vi "数据编码.vi"(0 "table输入":string(combo), 5 "错误常量 2":errorcluster caption="错误输入", 9 "QN":string, 13 "MN":string, 14 "PW":string) -> (4 "错误常量":errorcluster caption="错误输出", 15 "通讯包字符串":string)   [LabVIEW 2016, in "数据传输系统.lvlib"]
panel:
  in  "时间戳 2":string
  out "核查数据发送次数":i32
  out "小时数据发送次数":i32
  out "长度":i32
  in  "数据块":T1
  out "通讯包":T2={"包头（2）"="##", "数据段长度（4）"="", "数据段"="", "CRC校验"="", "包尾"=""}
  # "范例代码：\n\n##0101QN=20160801085857223;ST=32;CN=1062;PW=100000;MN=010000A8900016F000169DC0;Flag=5\n;CP=&&RtdInterval=30&&1C80\\r\\n"
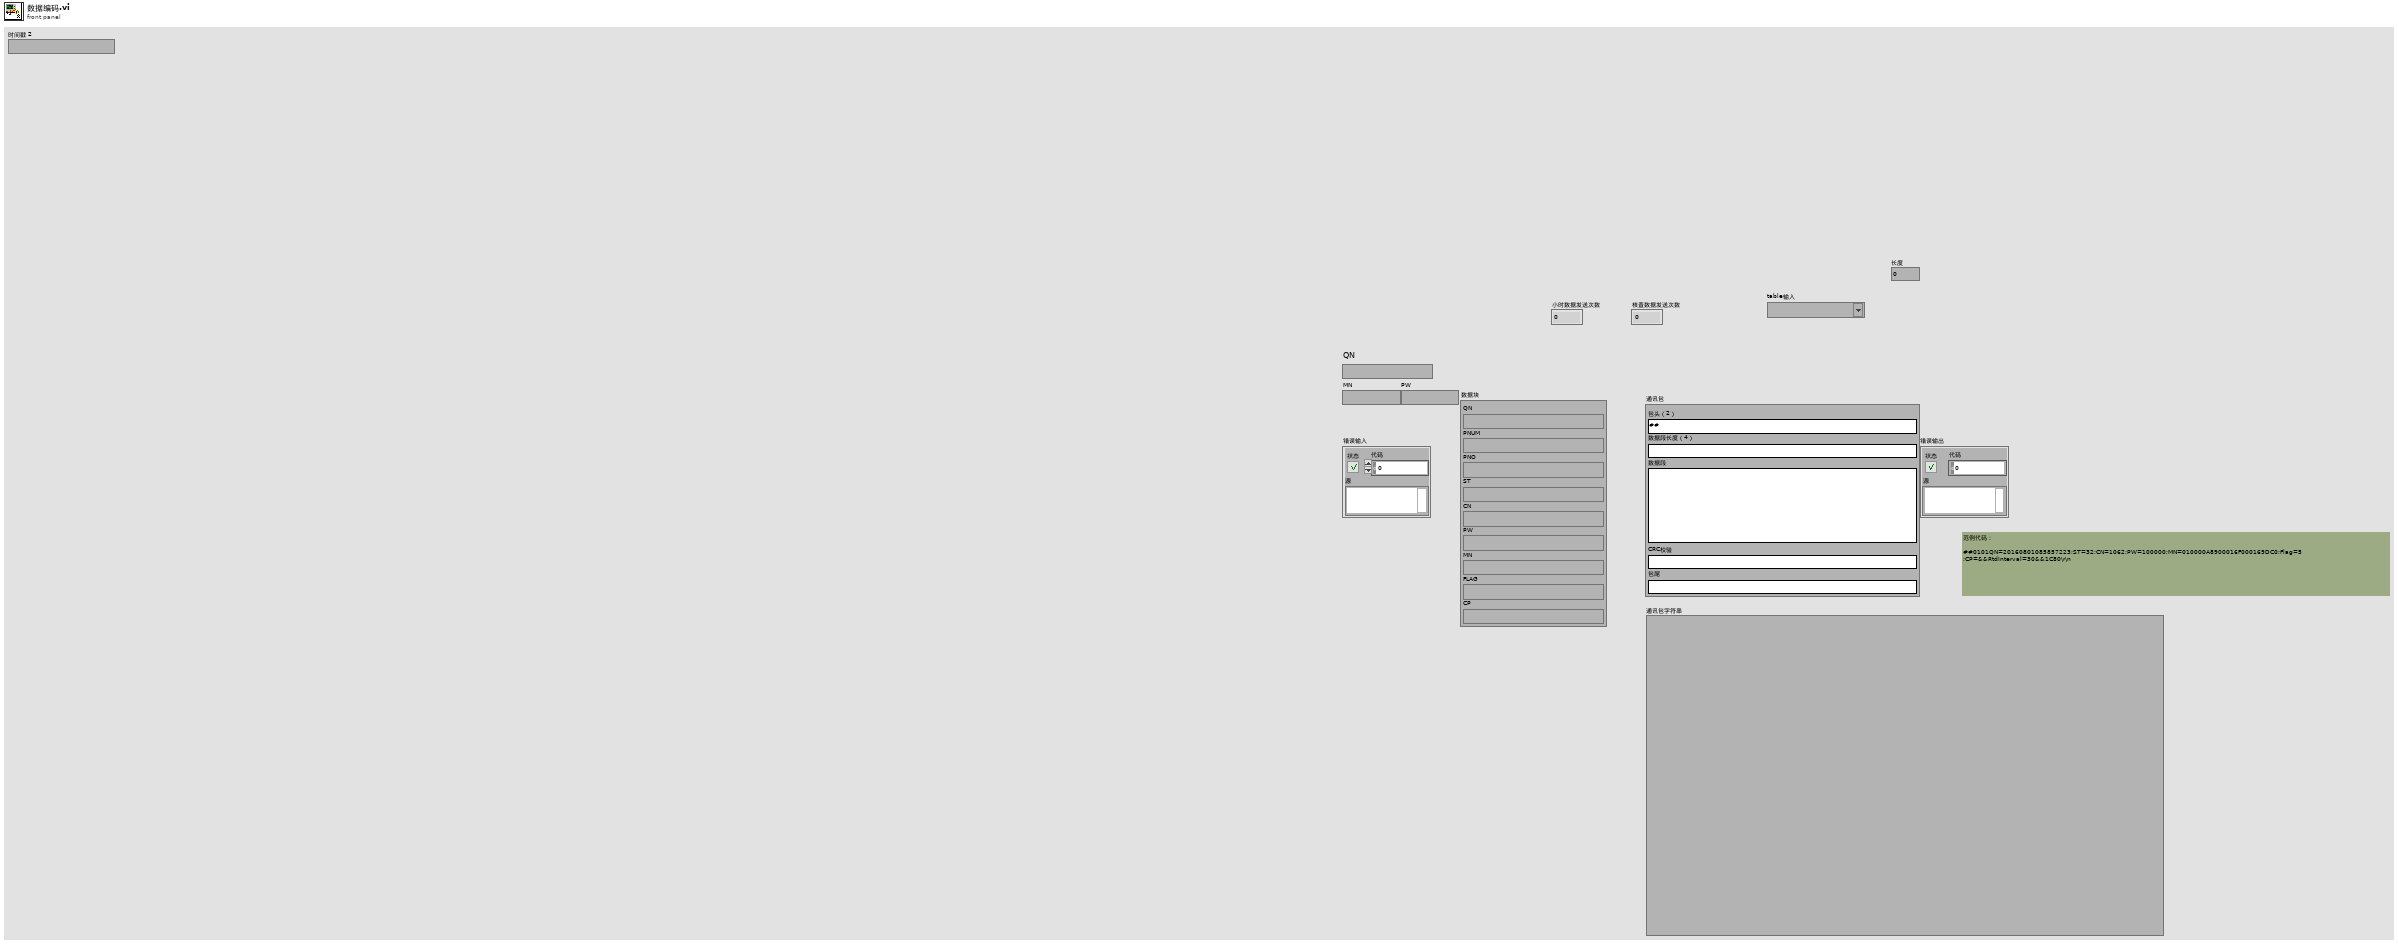
[diagram p1: front panel]
types:
  T1 = cluster{"QN":string, "ST":string, "CN":string, "PW":string, "MN":string, "FLAG":string, "PNUM":string, "PNO":string, "CP":string}
  T2 = cluster{"包头（2）":string, "数据段长度（4）":string, "数据段":string, "CRC校验":string, "包尾":string}
  T3 = cluster{"PH":string[][], "CODCr":string[][], "氨氮":string[][], "CODMn":string[][], "总氮":string[][], "总磷":string[][], "电导率":string[][], "水温":string[][], "DO":string[][], "浊度":string[][], "叶绿素":string[][], "藻密度":string[][], "铜":string[][], "盐度":string[][], "水位":string[][], "流速":string[][], "瞬时流量":string[][], "累积流量":string[][], "亚硝酸盐":string[][], "硫化物":string[][], "ORP":string[][], "铅":string[][], "镉":string[][], "锌":string[][], "镍":string[][], "锰":string[][], "汞":string[][]}
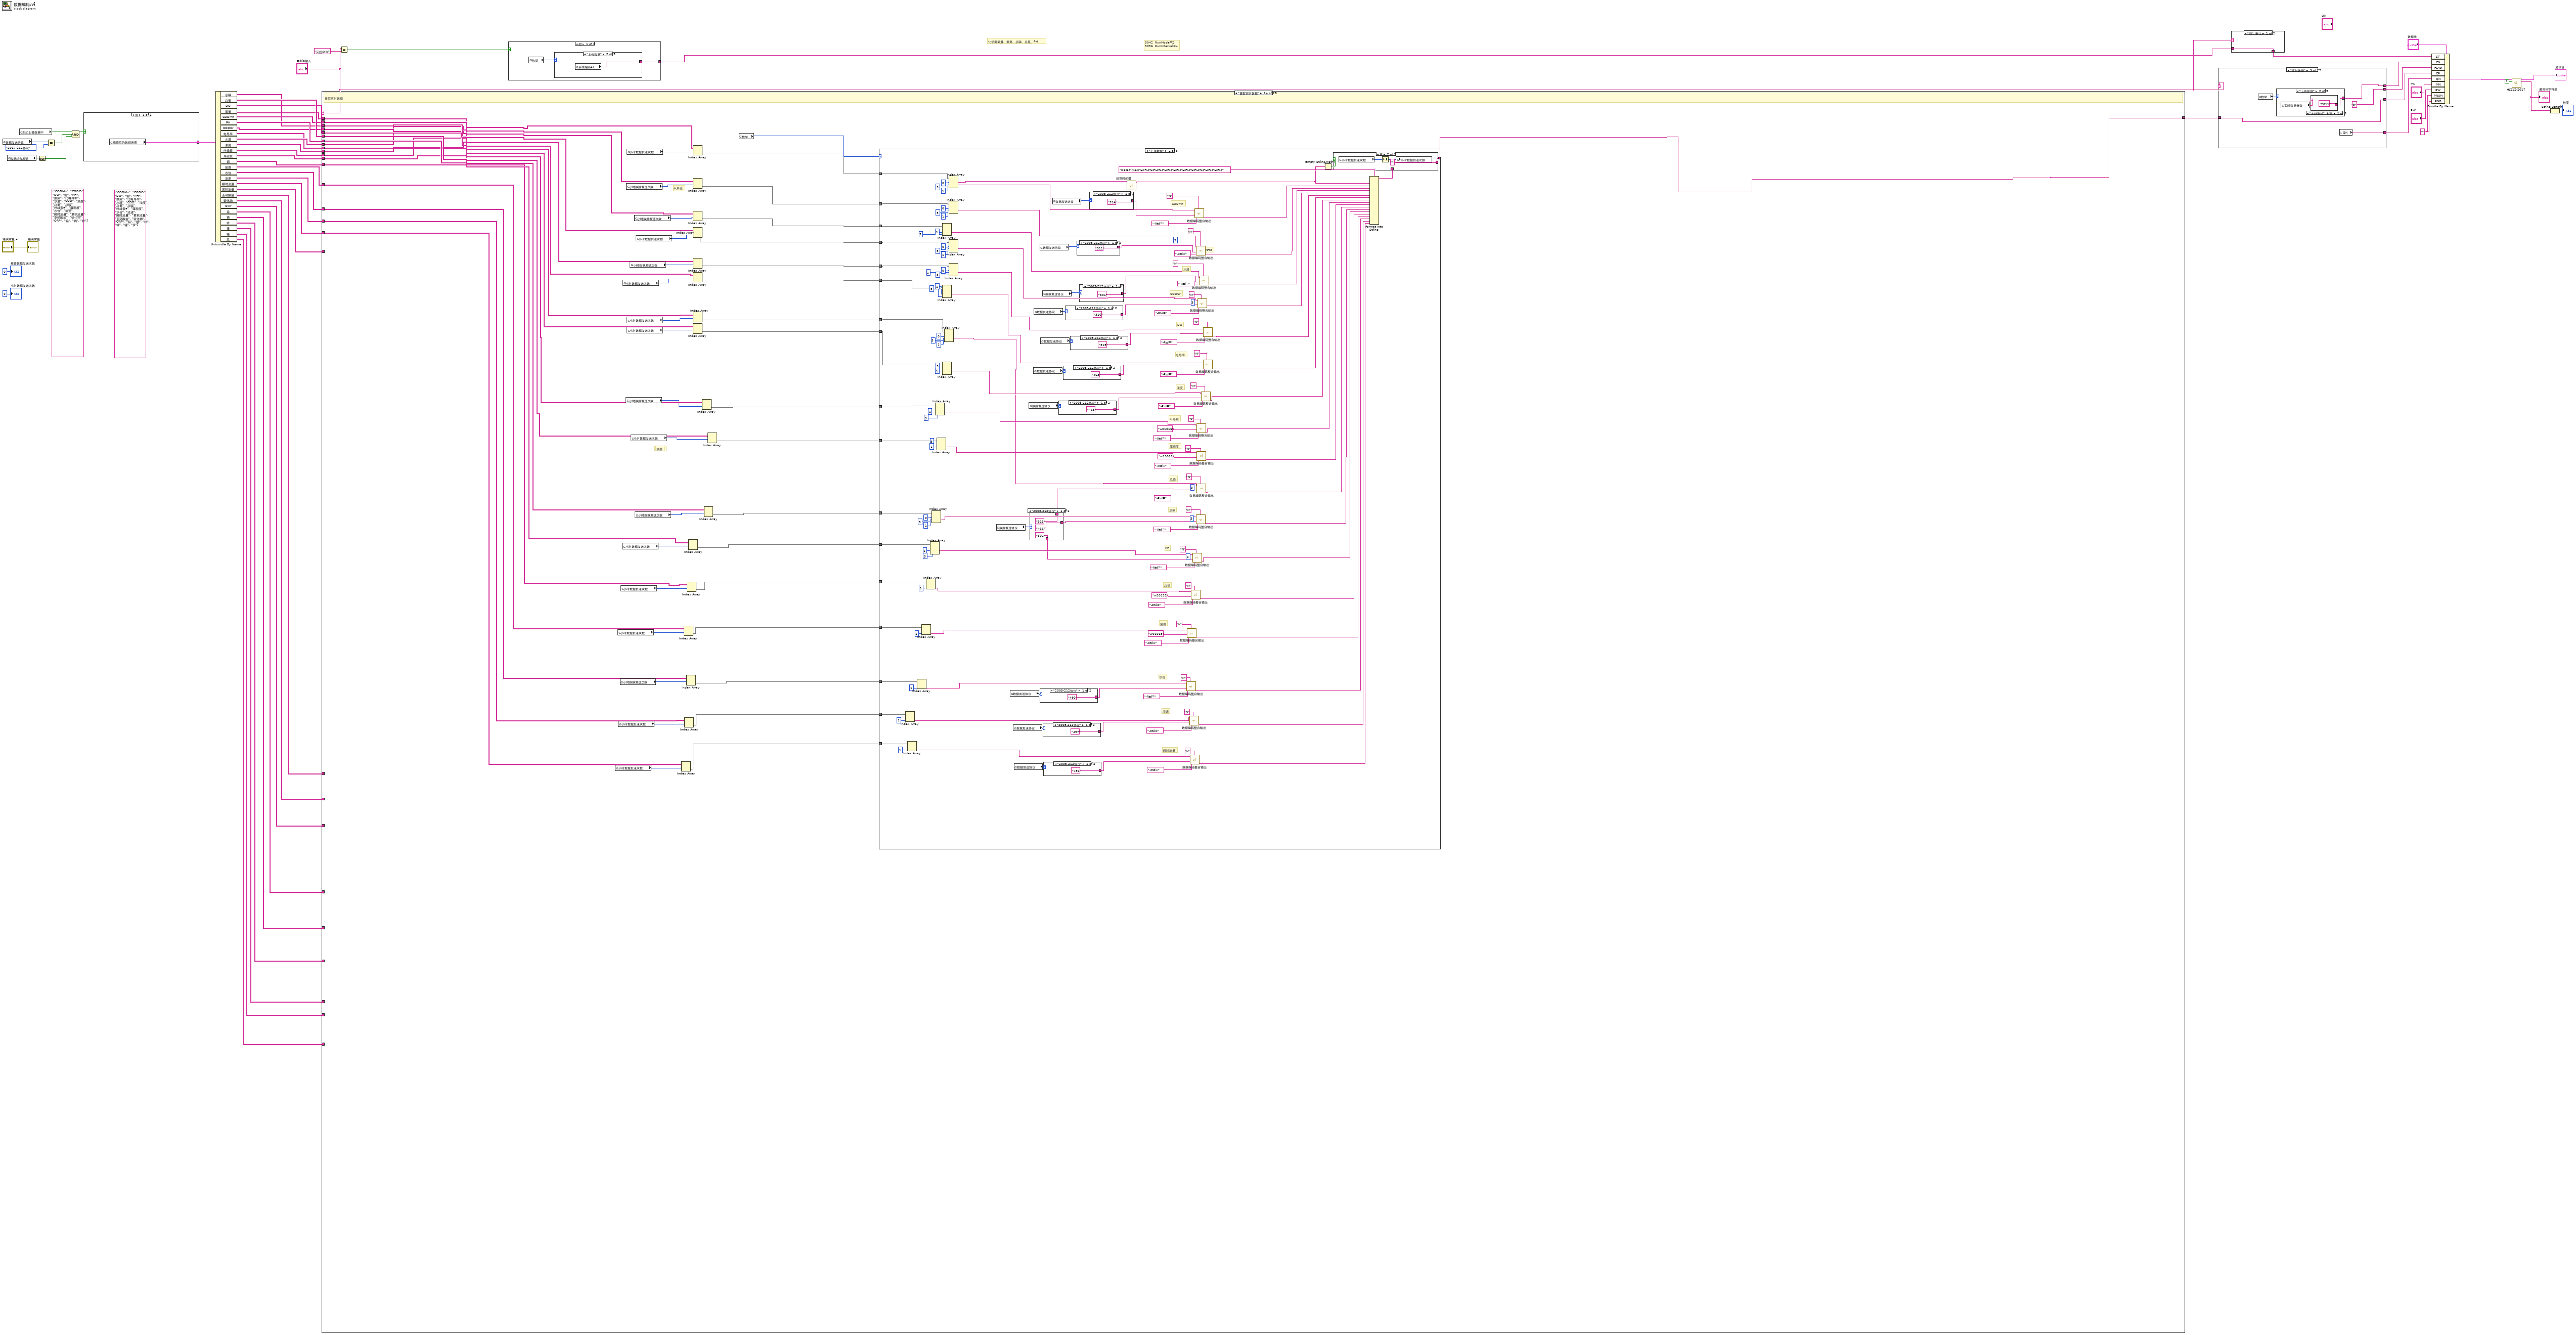
[diagram p0: block diagram]
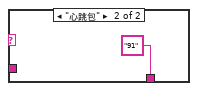
[diagram p2: hidden frame]
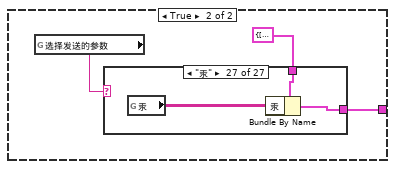
[diagram p3: hidden frame]
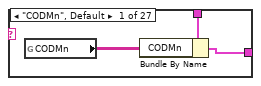
[diagram p4: hidden frame]
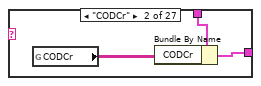
[diagram p5: hidden frame]
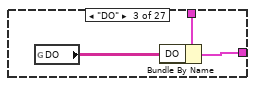
[diagram p6: hidden frame]
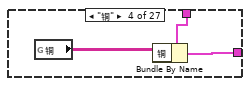
[diagram p7: hidden frame]
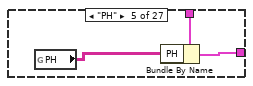
[diagram p8: hidden frame]
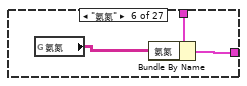
[diagram p9: hidden frame]
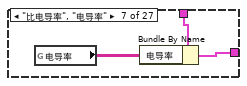
[diagram p10: hidden frame]
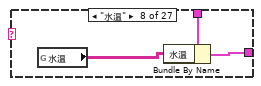
[diagram p11: hidden frame]
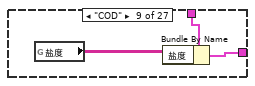
[diagram p12: hidden frame]
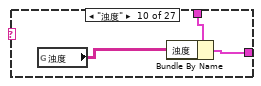
[diagram p13: hidden frame]
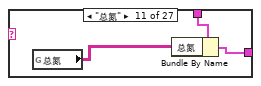
[diagram p14: hidden frame]
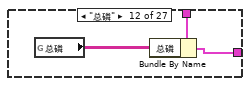
[diagram p15: hidden frame]
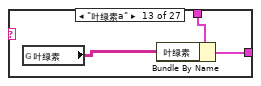
[diagram p16: hidden frame]
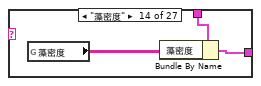
[diagram p17: hidden frame]
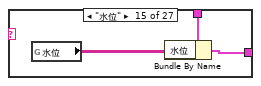
[diagram p18: hidden frame]
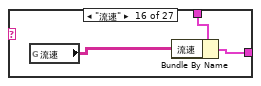
[diagram p19: hidden frame]
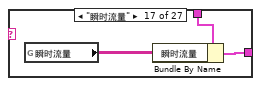
[diagram p20: hidden frame]
diagram:
  (unwired) string[] ["CODMn", "CODCr", "DO", "铜", "PH", "氨氮", "比电导率", "水温", "COD", "浊度", "总氮", "总磷", "叶绿素a", "藻密度", "水位", "流速", "瞬时流量", "累积流量", "亚硝酸盐", "硫化物", "ORP", "铅", "镉", "锌"] ("数组")
  (unwired) string[] ["CODMn", "CODCr", "DO", "铜", "PH", "氨氮", "比电导率", "水温", "COD", "浊度", "总氮", "总磷", "叶绿素a", "藻密度", "水位", "流速", "瞬时流量", "累积流量", "亚硝酸盐", "硫化物", "ORP", "铅", "镉", "锌", "镍", "锰", "汞"] ("数组")
  w42 = ""
  # "化学需氧量、氨氮、总磷、总氮、PH"
  # "3042  RunMode=2\n3056  RunInterval=4"
  n1 = global read "断电保存全局.vi" "数据发送协议"() -> (w15:enum16{"2005-212协议", "2017-212协议"})
  n2 = global read "断电保存全局.vi" "数据组合发送"() -> (w17:bool)
  n3 = global read "全局 数据发送重叠.vi" "主动上报数据中"() -> (w29:bool)
  n4 = Not(x=w17) -> (.not. x?=w16:bool)
  n5 = Equal?(x=w15, y=enum16{"2005-212协议", "2017-212协议"}."2017-212协议" ("数据发送版本")) -> (x = y?=w20:bool)
  n6 = Compound Arithmetic op=AND ("复合运算")(w29, w20, w16) -> (w21:bool)
  n7 = case shown="假" w21 {
    tunnel: [w58 w60] -> w30
    frame False {
      n8 = global read "插值后的新数组.vi" "插值后的数组元素"() -> (w58:T3)
    }
    frame True {
      n9 = global read "全局 水样时间.vi" "选择发送的参数"() -> (w61:string)
      n10 = case shown="\"汞\"" w61 {
        tunnel: T3 {"PH"=[], "CODCr"=[], "氨氮"=[], "CODMn"=[], "总氮"=[], "总磷"=[], "电导率"=[], "水温"=[], "DO"=[], "浊度"=[], "叶绿素"=[], "藻密度"=[], "铜"=[], "盐度"=[], "水位"=[], "流速"=[], "瞬时流量"=[], "累积流量"=[], "亚硝酸盐"=[], "硫化物"=[], "ORP"=[], "铅"=[], "镉"=[], "锌"=[], "镍"=[], "锰"=[], "汞"=[]} ("插值后的数组元素") -> [w63 w67 w70 w73 w76 w79 w82 w85 w88 w91 w94 w97 w100 w102 w106 w109 w111 w114 w117 w120 w123 w126 w129 w132 w135 w138 w141]
        tunnel: [w62 w65 w68 w71 w74 w77 w81 w84 w86 w89 w92 w95 w98 w101 w104 w107 w110 w113 w116 w119 w122 w125 w128 w131 w134 w137 w140] -> w60
        frame "CODMn", Default {
          n11 = global read "全局 所有参数.vi" "CODMn"() -> (w64:string[][])
          n12 = Bundle By Name(cluster=w63, "CODMn"=w64) -> (w62:T3)
        }
        frame "CODCr" {
          n13 = global read "全局 所有参数.vi" "CODCr"() -> (w66:string[][])
          n14 = Bundle By Name(cluster=w67, "CODCr"=w66) -> (w65:T3)
        }
        frame "DO" {
          n15 = global read "全局 所有参数.vi" "DO"() -> (w69:string[][])
          n16 = Bundle By Name(cluster=w70, "DO"=w69) -> (w68:T3)
        }
        frame "铜" {
          n17 = global read "全局 所有参数.vi" "铜"() -> (w72:string[][])
          n18 = Bundle By Name(cluster=w73, "铜"=w72) -> (w71:T3)
        }
        frame "PH" {
          n19 = global read "全局 所有参数.vi" "PH"() -> (w75:string[][])
          n20 = Bundle By Name(cluster=w76, "PH"=w75) -> (w74:T3)
        }
        frame "氨氮" {
          n21 = global read "全局 所有参数.vi" "氨氮"() -> (w78:string[][])
          n22 = Bundle By Name(cluster=w79, "氨氮"=w78) -> (w77:T3)
        }
        frame "比电导率", "电导率" {
          n23 = global read "全局 所有参数.vi" "电导率"() -> (w80:string[][])
          n24 = Bundle By Name(cluster=w82, "电导率"=w80) -> (w81:T3)
        }
        frame "水温" {
          n25 = global read "全局 所有参数.vi" "水温"() -> (w83:string[][])
          n26 = Bundle By Name(cluster=w85, "水温"=w83) -> (w84:T3)
        }
        frame "COD" {
          n27 = global read "全局 所有参数.vi" "盐度"() -> (w87:string[][])
          n28 = Bundle By Name(cluster=w88, "盐度"=w87) -> (w86:T3)
        }
        frame "浊度" {
          n29 = global read "全局 所有参数.vi" "浊度"() -> (w90:string[][])
          n30 = Bundle By Name(cluster=w91, "浊度"=w90) -> (w89:T3)
        }
        frame "总氮" {
          n31 = global read "全局 所有参数.vi" "总氮"() -> (w93:string[][])
          n32 = Bundle By Name(cluster=w94, "总氮"=w93) -> (w92:T3)
        }
        frame "总磷" {
          n33 = global read "全局 所有参数.vi" "总磷"() -> (w96:string[][])
          n34 = Bundle By Name(cluster=w97, "总磷"=w96) -> (w95:T3)
        }
        frame "叶绿素a" {
          n35 = global read "全局 所有参数.vi" "叶绿素"() -> (w99:string[][])
          n36 = Bundle By Name(cluster=w100, "叶绿素"=w99) -> (w98:T3)
        }
        frame "藻密度" {
          n37 = global read "全局 所有参数.vi" "藻密度"() -> (w103:string[][])
          n38 = Bundle By Name(cluster=w102, "藻密度"=w103) -> (w101:T3)
        }
        frame "水位" {
          n39 = global read "全局 所有参数.vi" "水位"() -> (w105:string[][])
          n40 = Bundle By Name(cluster=w106, "水位"=w105) -> (w104:T3)
        }
        frame "流速" {
          n41 = global read "全局 所有参数.vi" "流速"() -> (w108:string[][])
          n42 = Bundle By Name(cluster=w109, "流速"=w108) -> (w107:T3)
        }
        frame "瞬时流量" {
          n43 = global read "全局 所有参数.vi" "瞬时流量"() -> (w112:string[][])
          n44 = Bundle By Name(cluster=w111, "瞬时流量"=w112) -> (w110:T3)
        }
        frame "累积流量" {
          n45 = global read "全局 所有参数.vi" "累积流量"() -> (w115:string[][])
          n46 = Bundle By Name(cluster=w114, "累积流量"=w115) -> (w113:T3)
        }
        frame "亚硝氮" {
          n47 = global read "全局 所有参数.vi" "亚硝酸盐"() -> (w118:string[][])
          n48 = Bundle By Name(cluster=w117, "亚硝酸盐"=w118) -> (w116:T3)
        }
        frame "硫化物" {
          n49 = global read "全局 所有参数.vi" "硫化物"() -> (w121:string[][])
          n50 = Bundle By Name(cluster=w120, "硫化物"=w121) -> (w119:T3)
        }
        frame "ORP" {
          n51 = global read "全局 所有参数.vi" "ORP"() -> (w124:string[][])
          n52 = Bundle By Name(cluster=w123, "ORP"=w124) -> (w122:T3)
        }
        frame "铅" {
          n53 = global read "全局 所有参数.vi" "铅"() -> (w127:string[][])
          n54 = Bundle By Name(cluster=w126, "铅"=w127) -> (w125:T3)
        }
        frame "镉" {
          n55 = global read "全局 所有参数.vi" "镉"() -> (w130:string[][])
          n56 = Bundle By Name(cluster=w129, "镉"=w130) -> (w128:T3)
        }
        frame "锌" {
          n57 = global read "全局 所有参数.vi" "锌"() -> (w133:string[][])
          n58 = Bundle By Name(cluster=w132, "锌"=w133) -> (w131:T3)
        }
        frame "镍" {
          n59 = global read "全局 所有参数.vi" "镍"() -> (w136:string[][])
          n60 = Bundle By Name(cluster=w135, "镍"=w136) -> (w134:T3)
        }
        frame "锰" {
          n61 = global read "全局 所有参数.vi" "锰"() -> (w139:string[][])
          n62 = Bundle By Name(cluster=w138, "锰"=w139) -> (w137:T3)
        }
        frame "汞" {
          n63 = global read "全局 所有参数.vi" "汞"() -> (w142:string[][])
          n64 = Bundle By Name(cluster=w141, "汞"=w142) -> (w140:T3)
        }
      }
    }
  }
  n65 = Unbundle By Name(w30) -> ("总磷"=w23:string[][], "总氮"=w28:string[][], "DO"=w27:string[][], "氨氮"=w26:string[][], "CODMn"=w24:string[][], "PH"=w41:string[][], "CODCr"=w25:string[][], "电导率"=w19:string[][], "水温"=w40:string[][], "浊度"=w18:string[][], "叶绿素"=w39:string[][], "藻密度"=w36:string[][], "铜"=w35:string[][], "盐度"=w34:string[][], "水位"=w33:string[][], "流速"=w32:string[][], "瞬时流量"=w31:string[][], "累积流量"=w1:string[][], "亚硝酸盐"=w14:string[][], "硫化物"=w13:string[][], "ORP"=w12:string[][], "铅"=w10:string[][], "镉"=w9:string[][], "锌"=w8:string[][], "镍"=w7:string[][], "锰"=w6:string[][], "汞"=w5:string[][])
  n66 = case shown="\"提取实时数据\"" "table输入" {
    tunnel: [w144 w151 w165 w208 w231 _ w245 w254 w290 w1335 w1760 w1807 w1905 w2123 w2351 w2584 w2651 w2697 w2745 w2817 w2945 w3059 w3173 w3266 w3720 w3756 w3767 w3778] -> w37
    tunnel: w24 -> [_ _ _ _ _ _ _ _ w288 w1334 _ _ w1904 w2135 w2355 w2588 w2655 w2696 w2744 w2816 w2944 w3058 w3172 w3265 _ _ _ _]
    tunnel: w26 -> [_ _ _ _ _ _ _ _ w287 w1333 _ _ w1903 w2134 w2354 w2587 w2656 w2695 w2743 w2815 w2943 w3057 w3171 w3264 _ _ _ _]
    tunnel: w27 -> [_ _ _ _ _ _ _ _ w284 w1332 _ _ w1902 w2133 w2333 _ _ _ w2739 w2814 w2942 w3056 w3170 w3244 _ _ _ _]
    tunnel: w23 -> [_ _ _ _ _ _ _ _ w279 w1331 _ _ w1901 w2132 w2353 w2586 w2654 w2694 w2740 w2813 w2941 w3055 w3169 w3263 _ _ _ _]
    tunnel: w28 -> [_ _ _ _ _ _ _ _ w278 w1330 _ _ w1900 w2131 w2352 w2585 w2653 w2692 w2742 w2812 w2940 w3054 w3168 w3262 _ _ _ _]
    tunnel: w41 -> [_ _ _ _ _ _ _ _ w285 w1329 _ _ w1899 w2130 w2337 _ _ _ w2738 _ w2924 w3038 w3146 w3242 _ _ _ _]
    tunnel: w25 -> [_ _ _ _ _ _ _ _ w271 w1328 _ _ w1898 w2129 w2350 w2583 w2652 w2693 w2741 w2799 w2928 w3042 w3156 w3249 _ _ _ _]
    tunnel: w19 -> [_ _ _ _ _ _ _ _ w283 w1327 _ _ w1897 w2128 w2330 _ _ _ w2736 _ w2921 w3035 w3144 w3239 _ _ _ _]
    tunnel: w40 -> [_ _ _ _ _ _ _ _ w286 w1326 _ _ w1896 w2127 _ _ _ _ w2737 _ w2918 w3032 w3145 w3234 _ _ _ _]
    tunnel: w18 -> [_ _ _ _ _ _ _ _ w282 w1325 _ _ w1895 w2126 w2327 _ _ _ w2735 _ w2912 w3026 w3140 w3233 _ _ _ _]
    tunnel: w39 -> [_ _ _ _ _ _ _ _ w281 w1324 _ _ w1894 w2125 _ _ _ _ _ _ w2910 w3024 w3138 w3232 _ _ _ _]
    tunnel: w36 -> [_ _ _ _ _ _ _ _ w280 w1323 _ _ w1893 w2124 _ _ _ _ _ _ w2908 w3022 w3137 w3247 _ _ _ _]
    tunnel: w35 -> [_ _ _ _ _ _ _ _ w277 w1293 _ _ w1863 w2095 _ _ _ _ _ _ _ _ _ _ _ _ _ _]
    tunnel: w34 -> [_ _ _ _ _ _ _ _ w276 w1292 _ _ w1862 w2094 _ _ _ _ _ _ _ _ _ _ _ _ _ _]
    tunnel: w33 -> [_ _ _ _ _ _ _ _ w274 w1283 _ _ w1858 w2088 _ _ _ _ _ _ _ _ _ _ _ _ _ _]
    tunnel: w32 -> [_ _ _ _ _ _ _ _ w275 w1282 _ _ w1856 w2087 _ _ _ _ _ _ _ _ _ _ _ _ _ _]
    tunnel: w31 -> [_ _ _ _ _ _ _ _ w273 w1281 _ _ w1854 w2086 _ _ _ _ _ _ _ _ _ _ _ _ _ _]
    tunnel: w1 -> [_ _ _ _ _ _ _ _ w272 w1280 _ _ _ _ _ _ _ _ _ _ _ _ _ _ _ _ _ _]
    tunnel: w14 -> [_ _ _ _ _ _ _ _ w270 w1276 _ _ _ _ _ _ _ _ _ _ _ _ _ _ _ _ _ _]
    tunnel: w13 -> [_ _ _ _ _ _ _ _ w269 w1275 _ _ _ _ _ _ _ _ _ _ _ _ _ _ _ _ _ _]
    tunnel: w12 -> [_ _ _ _ _ _ _ _ w268 w1274 _ _ _ _ _ _ _ _ _ _ w2906 w3020 w3136 _ _ _ _ _]
    tunnel: w10 -> [_ _ _ _ _ _ _ _ w267 w1267 _ _ _ _ _ _ _ _ _ _ _ _ _ _ _ _ _ _]
    tunnel: w9 -> [_ _ _ _ _ _ _ _ w266 w1266 _ _ _ _ _ _ _ _ _ _ _ _ _ _ _ _ _ _]
    tunnel: w8 -> [_ _ _ _ _ _ _ _ w265 w1265 _ _ _ _ _ _ _ _ _ _ _ _ _ _ _ _ _ _]
    tunnel: w7 -> [_ _ _ _ _ _ _ _ w264 w1258 _ _ _ _ _ _ _ _ _ _ _ _ _ _ _ _ _ _]
    tunnel: w6 -> [_ _ _ _ _ _ _ _ w263 w1257 _ _ _ _ _ _ _ _ _ _ _ _ _ _ _ _ _ _]
    tunnel: w5 -> [_ _ _ _ _ _ _ _ w262 w1256 _ _ _ _ _ _ _ _ _ _ _ _ _ _ _ _ _ _]
    frame "反控命令" {
      n67 = global read "全局 反控命令枚举.vi" "反控命令枚举"() -> (w143:enum16{"返回请求应答", "返回执行结果"})
      n68 = case shown="\"返回执行结果\"" w143 {
        tunnel: ["QnRtn=1" w147] -> w144
        frame "返回请求应答", Default {
        }
        frame "返回执行结果" {
          n69 = global read "全局 反控命令枚举.vi" "执行结果定义"() -> (w148:u16)
          n70 = Number To Decimal String(number=w148) -> (decimal integer string=w146:string)  [unwired: 1 in]
          n71 = Concatenate Strings("ExeRtn=", w146) -> (w147:string)
        }
      }
    }
    frame "超标留样返回" {
      n72 = global read "全局1.vi" "枚举"() -> (w150:enum16{"返回请求应答", "上传数据", "返回执行结果"})
      n73 = case shown="\"返回请求应答\", 默认" w150 {
        tunnel: ["QnRtn=1" w153 "ExeRtn=1"] -> w151
        frame "返回请求应答", Default {
        }
        frame "上传数据" {
          n74 = global read "全局1.vi" "register values"() -> (w162:u16[])
          n75 = Index Array(array=w162, index=7 ("索引")) -> (element=w155:u16)
          n76 = Get Date/Time In Seconds() -> (seconds since 1Jan1904=w160:timestamp)
          n77 = Number To Decimal String(number=w155) -> (decimal integer string=w156:string)  [unwired: 1 in]
          n78 = Format Date/Time String(time format string (%c)="%Y%m%d%H%M%S" ("时间格式字符串(%c)"), seconds (now)=w160) -> (date/time string=w158:string)  [unwired: 1 in]
          n79 = Format Into String(format string="VaseNo=%s" ("格式字符串"), w156) -> (resulting string=w154:string)  [unwired: 2 in, 1 out]
          n80 = Format Into String(format string="DataTime=%s;%s" ("格式字符串"), w158, w154) -> (resulting string=w153:string)  [unwired: 2 in, 1 out]
        }
        frame "返回执行结果" {
        }
      }
    }
    frame "提取经纬度环境信息" {
      # "BDS纬度"
      # "BDS纬度"
      # "GPS纬度"
      # "GPS经度"
      # "湿度"
      # "温度"
      # "电压"
      # "时间"
      n81 = global read "全局1.vi" "枚举"() -> (w166:enum16{"返回请求应答", "上传数据", "返回执行结果"})
      n82 = case shown="\"上传数据\"" w166 {
        tunnel: ["QnRtn=1" w179 "ExeRtn=1"] -> w165
        frame "返回请求应答", Default {
        }
        frame "上传数据" {
          n83 = global read "全局 环境参数.vi" "columns输出"() -> (w176:string[])
          n84 = Array Subset(array=w176, index=1 ("索引")) -> (w177:string[])  [unwired: 1 in]
          n85 = for {
            tunnel: w177 -> [w185] mode=indexing
            tunnel: [w184] -> w178 mode=indexing
            n86 = case shown="\"BDS经度\"" w185 {
              tunnel: ["" "Volt=%s;" "Temp=%s;" ("格式字符串") "Hum=%s;" ("格式字符串") "Lng=%s;" "Lat=%s;" "Lng2=%s;" "Lat2=%s;"] -> w184
              frame "假", Default {
              }
              frame "电压" {
              }
              frame "室温" {
              }
              frame "湿度" {
              }
              frame "GPS经度" {
              }
              frame "GPS纬度" {
              }
              frame "BDS经度" {
              }
              frame "BDS纬度" {
              }
            }
          }
          n87 = global read "全局 环境参数.vi" "环境参数"() -> (w169:string[][])
          n88 = Index Array(array=w169, index (row)=0 ("索引 (行)")) -> (element=w172:string[])  [unwired: 1 in]
          n89 = Array Subset(array=w172, index=1 ("索引")) -> (w174:string[])  [unwired: 1 in]
          n90 = for {
            shift-right: [w199] -> w168
            shift-left: "" -> [w198]
            tunnel: w178 -> [w197] mode=indexing
            tunnel: w174 -> [w195] mode=indexing
            n91 = Fract/Exp String To Number(string=w195) -> (number=w196:dbl)  [unwired: 3 in, 1 out]
            n92 = Empty String/Path?(string/path=w195) -> (empty?=w201:bool)
            n93 = Number To Fractional String(number=w196) -> (F-format string=w194:string)  [unwired: 3 in]
            n94 = case shown="假" w201 {
              tunnel: [w204 w205] -> w200
              tunnel: w197 -> [w203 _]
              tunnel: w194 -> [w202 _]
              tunnel: w194 -> [_ w205]
              frame False {
                n95 = Format Into String(format string=w203, w202) -> (resulting string=w204:string)  [unwired: 2 in, 1 out]
              }
              frame True {
              }
            }
            n96 = Concatenate Strings(w198, w200) -> (w199:string)
          }
          n97 = Get Date/Time In Seconds() -> (seconds since 1Jan1904=w181:timestamp)
          n98 = Format Date/Time String(time format string (%c)="%Y%m%d%H%M%S" ("时间格式字符串(%c)"), seconds (now)=w181) -> (date/time string=w180:string)  [unwired: 1 in]
          n99 = Format Into String(format string="DataTime=%s;%s" ("格式字符串"), w180, w168) -> (resulting string=w179:string)  [unwired: 2 in, 1 out]
        }
        frame "返回执行结果" {
        }
      }
    }
    frame "提取现场系统信息" {
      n100 = global read "全局1.vi" "枚举"() -> (w207:enum16{"返回请求应答", "上传数据", "返回执行结果"})
      n101 = case shown="\"上传数据\"" w207 {
        tunnel: ["QnRtn=1" w228 "ExeRtn=1"] -> w208
        frame "返回请求应答", Default {
        }
        frame "上传数据" {
          n102 = global read "全局1.vi" "register values"() -> (w227:u16[])
          n103 = Get Date/Time In Seconds() -> (seconds since 1Jan1904=w213:timestamp)
          n104 = Index Array(array=w227, index #1=0 ("索引"), index #2=6 ("索引")) -> (element #1=w223:u16, element #2=w210:u16)
          n105 = Format Date/Time String(time format string (%c)="%Y%m%d%H%M%S%u" ("时间格式字符串(%c)"), seconds (now)=w213) -> (date/time string=w216:string)  [unwired: 1 in]
          n106 = Number To Decimal String(number=w223) -> (decimal integer string=w225:string)  [unwired: 1 in]
          n107 = Number To Decimal String(number=w210) -> (decimal integer string=w219:string)  [unwired: 1 in]
          n108 = Search and Replace String(input string=w216, search string="." ("搜索字符串")) -> (result string=w212:string)  [unwired: 6 in, 3 out]
          n109 = Format Into String(format string="RunMode=%s;" ("格式字符串"), w225) -> (resulting string=w222:string)  [unwired: 2 in, 1 out]
          n110 = Format Into String(format string="RunInterval=%s;" ("格式字符串"), w219) -> (resulting string=w220:string)  [unwired: 2 in, 1 out]
          n111 = Format Into String(format string="SystemTime=%s;" ("格式字符串"), w212) -> (resulting string=w217:string)  [unwired: 2 in, 1 out]
          n112 = Concatenate Strings(w222, w220, w217) -> (w228:string)
        }
        frame "返回执行结果" {
        }
      }
    }
    frame "提取监测仪表时间" {
      n113 = global read "全局1.vi" "枚举"() -> (w230:enum16{"返回请求应答", "上传数据", "返回执行结果"})
      n114 = case shown="\"上传数据\"" w230 {
        tunnel: ["QnRtn=1" w243 "ExeRtn=1"] -> w231
        frame "返回请求应答", Default {
        }
        frame "上传数据" {
          n115 = global read "全局 提取仪器参数.vi" "仪器编码"() -> (w233:string)
          n116 = Get Date/Time In Seconds() -> (seconds since 1Jan1904=w236:timestamp)
          n117 = Format Date/Time String(time format string (%c)="%Y%m%d%H%M%S%u" ("时间格式字符串(%c)"), seconds (now)=w236) -> (date/time string=w239:string)  [unwired: 1 in]
          n118 = Search and Replace String(input string=w239, search string="." ("搜索字符串")) -> (result string=w235:string)  [unwired: 6 in, 3 out]
          n119 = Format Into String(format string="PolId=%s;" ("格式字符串"), w233) -> (resulting string=w241:string)  [unwired: 2 in, 1 out]
          n120 = Format Into String(format string="SystemTime=%s;" ("格式字符串"), w235) -> (resulting string=w234:string)  [unwired: 2 in, 1 out]
          n121 = Concatenate Strings(w241, w234) -> (w243:string)
        }
        frame "返回执行结果" {
        }
      }
    }
    frame "心跳包", Default {
    }
    frame "提取数采仪时间" {
      (unwired) ""
      n122 = global read "全局1.vi" "枚举"() -> (w246:enum16{"返回请求应答", "上传数据", "返回执行结果"})
      n123 = case shown="\"上传数据\"" w246 {
        tunnel: ["QnRtn=1" w248 "ExeRtn=1"] -> w245
        frame "返回请求应答", Default {
        }
        frame "上传数据" {
          n124 = Get Date/Time In Seconds() -> (seconds since 1Jan1904=w252:timestamp)
          n125 = Format Date/Time String(time format string (%c)="%Y%m%d%H%M%S" ("时间格式字符串(%c)"), seconds (now)=w252) -> (date/time string=w249:string)  [unwired: 1 in]
          n126 = Concatenate Strings("SystemTime=", w249) -> (w248:string)
        }
        frame "返回执行结果" {
        }
      }
    }
    frame "提取实时数据间隔" {
      (unwired) ""
      n127 = global read "全局1.vi" "枚举"() -> (w255:enum16{"返回请求应答", "上传数据", "返回执行结果"})
      n128 = case shown="\"上传数据\"" w255 {
        tunnel: ["QnRtn=1" w259 "ExeRtn=1"] -> w254
        frame "返回请求应答", Default {
        }
        frame "上传数据" {
          n129 = global read "实时数据发送间隔全局.vi" "实时数据发送间隔"() -> (w258:u32)
          n130 = Number To Decimal String(number=w258) -> (decimal integer string=w257:string)  [unwired: 1 in]
          n131 = Concatenate Strings("RtdInterval=", w257) -> (w259:string)
        }
        frame "返回执行结果" {
        }
      }
    }
    frame "实时数据" {
      # "包含质控数据主动上传"
      n132 = global read "全局 实时数据参数.vi" "实时数据参数"() -> (w289:string)
      n133 = case shown="\"水样测试\", 默认" w289 {
        tunnel: [w318 w696 w747 w826 w1088 w1157] -> w290
        tunnel: w288 -> [w317 w695 w746 w813 w1086 w1155]
        tunnel: w287 -> [w316 w694 w745 w814 w1085 w1154]
        tunnel: w286 -> [w315 w693 w744 w815 _ _]
        tunnel: w285 -> [w314 w692 w743 w816 w1081 _]
        tunnel: w284 -> [w313 w691 w742 w817 w1080 _]
        tunnel: w283 -> [w312 w690 w741 w818 w1079 _]
        tunnel: w282 -> [w311 w689 w740 w819 w1078 _]
        tunnel: w281 -> [w310 w688 w739 w820 w1077 _]
        tunnel: w280 -> [w309 w687 w738 w821 w1076 _]
        tunnel: w279 -> [w308 w686 w737 w822 w1084 w1153]
        tunnel: w278 -> [w307 w685 w736 w823 w1083 w1152]
        tunnel: w271 -> [w306 w684 w735 w824 w1082 w1151]
        tunnel: w277 -> [w305 w683 w734 w812 _ _]
        tunnel: w276 -> [w304 w682 w733 w811 _ _]
        tunnel: w274 -> [w303 _ _ _ _ _]
        tunnel: w273 -> [w302 _ _ _ _ _]
        tunnel: w272 -> [w301 _ _ _ _ _]
        tunnel: w275 -> [w300 _ _ _ _ _]
        tunnel: w270 -> [w299 _ w732 _ w1073 w1150]
        tunnel: w269 -> [w298 _ w731 _ w1074 w1149]
        tunnel: w268 -> [w297 _ w730 _ w1075 w1148]
        tunnel: w267 -> [w296 _ _ _ _ _]
        tunnel: w266 -> [w295 _ _ _ _ _]
        tunnel: w265 -> [w294 _ _ _ _ _]
        tunnel: w264 -> [w293 _ _ _ _ _]
        tunnel: w263 -> [w292 _ _ _ _ _]
        tunnel: w262 -> [w291 _ _ _ _ _]
        frame "水样测试", Default {
          n134 = global read "全局1.vi" "枚举"() -> (w319:enum16{"返回请求应答", "上传数据", "返回执行结果"})
          n135 = case shown="\"上传数据\"" w319 {
            tunnel: ["QnRtn=1" w554 "ExeRtn=1"] -> w318
            tunnel: w317 -> [_ w566 _]
            tunnel: w316 -> [_ w565 _]
            tunnel: w315 -> [_ w564 _]
            tunnel: w314 -> [_ w563 _]
            tunnel: w313 -> [_ w562 _]
            tunnel: w312 -> [_ w561 _]
            tunnel: w311 -> [_ w560 _]
            tunnel: w310 -> [_ w559 _]
            tunnel: w309 -> [_ w558 _]
            tunnel: w308 -> [_ w557 _]
            tunnel: w307 -> [_ w556 _]
            tunnel: w306 -> [_ w555 _]
            tunnel: w305 -> [_ w513 _]
            tunnel: w304 -> [_ w512 _]
            tunnel: w303 -> [_ w509 _]
            tunnel: w300 -> [_ w508 _]
            tunnel: w302 -> [_ w507 _]
            tunnel: w301 -> [_ w439 _]
            tunnel: w299 -> [_ w446 _]
            tunnel: w298 -> [_ w445 _]
            tunnel: w297 -> [_ w444 _]
            tunnel: w296 -> [_ w359 _]
            tunnel: w295 -> [_ w358 _]
            tunnel: w294 -> [_ w357 _]
            tunnel: w293 -> [_ w326 _]
            tunnel: w292 -> [_ w325 _]
            tunnel: w291 -> [_ w324 _]
            frame "返回请求应答", Default {
            }
            frame "上传数据" {
              # "汞"
              # "锰"
              # "镍"
              # "锌"
              # "镉"
              # "铅"
              # "藻密度"
              # "叶绿素a"
              # "浊度"
              # "电导率"
              # "DO"
              # "水温"
              # "CODMn"
              # "ORP"
              # "硫化物"
              # "亚硝酸盐"
              # "CODCr"
              # "总氮"
              # "总磷"
              # "PH"
              # "NH3"
              n136 = global read "断电保存全局.vi" "数据发送协议"() -> (w475:enum16{"2005-212协议", "2017-212协议"})
              n137 = global read "断电保存全局.vi" "数据发送协议"() -> (w479:enum16{"2005-212协议", "2017-212协议"})
              n138 = global read "断电保存全局.vi" "数据发送协议"() -> (w474:enum16{"2005-212协议", "2017-212协议"})
              n139 = global read "断电保存全局.vi" "数据发送协议"() -> (w477:enum16{"2005-212协议", "2017-212协议"})
              n140 = global read "断电保存全局.vi" "数据发送协议"() -> (w478:enum16{"2005-212协议", "2017-212协议"})
              n141 = global read "断电保存全局.vi" "数据发送协议"() -> (w476:enum16{"2005-212协议", "2017-212协议"})
              n142 = case shown="\"2017-212协议\", 默认" w474 {
                tunnel: ["060" ("污染物编码") "w21003" ("污染物编码")] -> w550
                frame "2005-212协议" {
                }
                frame "2017-212协议", Default {
                }
              }
              n143 = case shown="\"2005-212协议\"" w475 {
                tunnel: ["001" ("污染物编码") "w01001" ("污染物编码")] -> w543
                frame "2005-212协议" {
                }
                frame "2017-212协议", Default {
                }
              }
              n144 = global read "全局 水样时间.vi" "选择发送的参数"() -> (w493:string)
              n145 = case shown="\"2005-212协议\"" w477 {
                tunnel: ["065" ("污染物编码") "w21001" ("污染物编码")] -> w528
                frame "2005-212协议" {
                }
                frame "2017-212协议", Default {
                }
              }
              n146 = case shown="\"2017-212协议\", 默认" w476 {
                tunnel: ["011" ("污染物编码") "w01018" ("污染物编码")] -> w522
                frame "2005-212协议" {
                }
                frame "2017-212协议", Default {
                }
              }
              n147 = case shown="\"2005-212协议\"" w478 {
                tunnel: ["101" ("污染物编码") "w21011" ("污染物编码")] -> w532
                frame "2005-212协议" {
                }
                frame "2017-212协议", Default {
                }
              }
              n148 = case shown="\"汞\"" w493 {
                tunnel: [w648 w649 w650 w651 w652 w653 w654 w655 w656 w657 w658 w659 w660 w661 w662 w663 w664 w665 w666 w667 w668 w669 w670 w671 w672 w673 w674] -> w491
                frame "CODMn", Default {
                  n149 = global read "全局 所有参数.vi" "CODMn"() -> (w648:string[][])
                }
                frame "CODCr" {
                  n150 = global read "全局 所有参数.vi" "CODCr"() -> (w649:string[][])
                }
                frame "DO" {
                  n151 = global read "全局 所有参数.vi" "DO"() -> (w650:string[][])
                }
                frame "铜" {
                  n152 = global read "全局 所有参数.vi" "铜"() -> (w651:string[][])
                }
                frame "PH" {
                  n153 = global read "全局 所有参数.vi" "PH"() -> (w652:string[][])
                }
                frame "氨氮" {
                  n154 = global read "全局 所有参数.vi" "氨氮"() -> (w653:string[][])
                }
                frame "比电导率", "电导率" {
                  n155 = global read "全局 所有参数.vi" "电导率"() -> (w654:string[][])
                }
                frame "水温" {
                  n156 = global read "全局 所有参数.vi" "水温"() -> (w655:string[][])
                }
                frame "COD" {
                  n157 = global read "全局 所有参数.vi" "盐度"() -> (w656:string[][])
                }
                frame "浊度" {
                  n158 = global read "全局 所有参数.vi" "浊度"() -> (w657:string[][])
                }
                frame "总氮" {
                  n159 = global read "全局 所有参数.vi" "总氮"() -> (w658:string[][])
                }
                frame "总磷" {
                  n160 = global read "全局 所有参数.vi" "总磷"() -> (w659:string[][])
                }
                frame "叶绿素a" {
                  n161 = global read "全局 所有参数.vi" "叶绿素"() -> (w660:string[][])
                }
                frame "藻密度" {
                  n162 = global read "全局 所有参数.vi" "藻密度"() -> (w661:string[][])
                }
                frame "水位" {
                  n163 = global read "全局 所有参数.vi" "水位"() -> (w662:string[][])
                }
                frame "流速" {
                  n164 = global read "全局 所有参数.vi" "流速"() -> (w663:string[][])
                }
                frame "瞬时流量" {
                  n165 = global read "全局 所有参数.vi" "瞬时流量"() -> (w664:string[][])
                }
                frame "累积流量" {
                  n166 = global read "全局 所有参数.vi" "累积流量"() -> (w665:string[][])
                }
                frame "亚硝氮" {
                  n167 = global read "全局 所有参数.vi" "亚硝酸盐"() -> (w666:string[][])
                }
                frame "硫化物" {
                  n168 = global read "全局 所有参数.vi" "硫化物"() -> (w667:string[][])
                }
                frame "ORP" {
                  n169 = global read "全局 所有参数.vi" "ORP"() -> (w668:string[][])
                }
                frame "铅" {
                  n170 = global read "全局 所有参数.vi" "铅"() -> (w669:string[][])
                }
                frame "镉" {
                  n171 = global read "全局 所有参数.vi" "镉"() -> (w670:string[][])
                }
                frame "锌" {
                  n172 = global read "全局 所有参数.vi" "锌"() -> (w671:string[][])
                }
                frame "镍" {
                  n173 = global read "全局 所有参数.vi" "镍"() -> (w672:string[][])
                }
                frame "锰" {
                  n174 = global read "全局 所有参数.vi" "锰"() -> (w673:string[][])
                }
                frame "汞" {
                  n175 = global read "全局 所有参数.vi" "汞"() -> (w674:string[][])
                }
              }
              n176 = global read "全局 小时数据发送次数.vi" "小时数据发送次数"() -> (w432:i32)
              n177 = global read "全局 小时数据发送次数.vi" "小时数据发送次数"() -> (w396:i32)
              n178 = global read "全局 小时数据发送次数.vi" "小时数据发送次数"() -> (w517:i32)
              n179 = global read "全局 小时数据发送次数.vi" "小时数据发送次数"() -> (w516:i32)
              n180 = global read "全局 小时数据发送次数.vi" "小时数据发送次数"() -> (w424:i32)
              n181 = global read "全局 小时数据发送次数.vi" "小时数据发送次数"() -> (w492:i32)
              n182 = global read "全局 小时数据发送次数.vi" "小时数据发送次数"() -> (w397:i32)
              n183 = global read "全局 小时数据发送次数.vi" "小时数据发送次数"() -> (w398:i32)
              n184 = global read "全局 小时数据发送次数.vi" "小时数据发送次数"() -> (w399:i32)
              n185 = global read "全局 小时数据发送次数.vi" "小时数据发送次数"() -> (w400:i32)
              n186 = global read "全局 小时数据发送次数.vi" "小时数据发送次数"() -> (w515:i32)
              n187 = case shown="\"2005-212协议\"" w479 {
                tunnel: w513 -> [_ w628]
                tunnel: w512 -> [_ w627]
                tunnel: [w571 w626] -> w511
                tunnel: [w571 w625] -> w510
                tunnel: w509 -> [_ w611]
                tunnel: w508 -> [_ w610]
                tunnel: w507 -> [w569 w609]
                tunnel: [w571 w608] -> w506
                tunnel: [w571 w607] -> w505
                tunnel: [w570 w606] -> w504
                tunnel: w439 -> [_ w583]
                tunnel: [w571 w582] -> w438
                frame "2005-212协议" {
                  w571 = "" ("编码输出")
                  # "瞬时流量"
                  n188 = global read "全局 小时数据发送次数.vi" "小时数据发送次数"() -> (w577:i32)
                  n189 = Index Array(array=w569, index (row)=w577) -> (element=w575:string[])  [unwired: 1 in]
                  n190 = Index Array(array=w575, index #1=5 ("索引"), index #2=1 ("索引")) -> (element #2=w574:string)  [unwired: 1 out]
                  n191 = call "数据编码整合输出.vi"("数据标识"="N", "数据类型"="-Rtd=", "污染物编码"="B01", "数据值"=w574) -> ("编码输出"=w570:string)  [unwired: 7 in]
                }
                frame "2017-212协议", Default {
                  # "累计流量"
                  # "瞬时流量"
                  # "流速"
                  # "水位"
                  # "盐度改COD"
                  # "总铜"
                  n192 = global read "全局 小时数据发送次数.vi" "小时数据发送次数"() -> (w630:i32)
                  n193 = global read "全局 小时数据发送次数.vi" "小时数据发送次数"() -> (w629:i32)
                  n194 = global read "全局 小时数据发送次数.vi" "小时数据发送次数"() -> (w624:i32)
                  n195 = global read "全局 小时数据发送次数.vi" "小时数据发送次数"() -> (w616:i32)
                  n196 = global read "全局 小时数据发送次数.vi" "小时数据发送次数"() -> (w615:i32)
                  n197 = global read "全局 小时数据发送次数.vi" "小时数据发送次数"() -> (w586:i32)
                  n198 = Index Array(array=w628, index (row)=w630) -> (element=w634:string[])  [unwired: 1 in]
                  n199 = Index Array(array=w627, index (row)=w629) -> (element=w633:string[])  [unwired: 1 in]
                  n200 = Index Array(array=w611, index (row)=w624) -> (element=w621:string[])  [unwired: 1 in]
                  n201 = Index Array(array=w610, index (row)=w616) -> (element=w620:string[])  [unwired: 1 in]
                  n202 = Index Array(array=w609, index (row)=w615) -> (element=w612:string[])  [unwired: 1 in]
                  n203 = Index Array(array=w583, index (row)=w586) -> (element=w589:string[])  [unwired: 1 in]
                  n204 = Index Array(array=w634, index #1=5 ("索引"), index #2=3 ("索引")) -> (element #1=w605:string, element #2=w604:string)
                  n205 = Index Array(array=w633, index #1=5 ("索引"), index #2=3 ("索引")) -> (element #1=w603:string, element #2=w602:string)
                  n206 = Index Array(array=w621, index #1=5 ("索引"), index #2=1 ("索引")) -> (element #2=w600:string)  [unwired: 1 out]
                  n207 = Index Array(array=w620, index #1=5 ("索引"), index #2=1 ("索引")) -> (element #2=w599:string)  [unwired: 1 out]
                  n208 = Index Array(array=w612, index #1=5 ("索引"), index #2=1 ("索引")) -> (element #2=w598:string)  [unwired: 1 out]
                  n209 = Index Array(array=w589, index #1=5 ("索引"), index #2=1 ("索引")) -> (element #2=w585:string)  [unwired: 1 out]
                  n210 = call "数据编码整合输出.vi"("数据标识"=w605, "数据类型"="-Rtd=", "污染物编码"="w20122", "数据值"=w604) -> ("编码输出"=w626:string)  [unwired: 7 in]
                  n211 = call "数据编码整合输出.vi"("数据标识"=w603, "数据类型"="-Rtd=", "污染物编码"="w01018", "数据值"=w602) -> ("编码输出"=w625:string)  [unwired: 7 in]
                  n212 = call "数据编码整合输出.vi"("数据标识"="N", "数据类型"="-Rtd=", "污染物编码"="e01201", "数据值"=w600) -> ("编码输出"=w608:string)  [unwired: 7 in]
                  n213 = call "数据编码整合输出.vi"("数据标识"="N", "数据类型"="-Rtd=", "污染物编码"="e01202", "数据值"=w599) -> ("编码输出"=w607:string)  [unwired: 7 in]
                  n214 = call "数据编码整合输出.vi"("数据标识"="N", "数据类型"="-Rtd=", "污染物编码"="e01203", "数据值"=w598) -> ("编码输出"=w606:string)  [unwired: 7 in]
                  n215 = call "数据编码整合输出.vi"("数据标识"="N", "数据类型"="-Rtd=", "污染物编码"="e01204", "数据值"=w585) -> ("编码输出"=w582:string)  [unwired: 7 in]
                }
              }
              n216 = global read "全局 小时数据发送次数.vi" "小时数据发送次数"() -> (w518:i32)
              n217 = global read "全局 小时数据发送次数.vi" "小时数据发送次数"() -> (w454:i32)
              n218 = global read "全局 小时数据发送次数.vi" "小时数据发送次数"() -> (w470:i32)
              n219 = global read "全局 小时数据发送次数.vi" "小时数据发送次数"() -> (w377:i32)
              n220 = global read "全局 小时数据发送次数.vi" "小时数据发送次数"() -> (w461:i32)
              n221 = global read "全局 小时数据发送次数.vi" "小时数据发送次数"() -> (w363:i32)
              n222 = global read "全局 小时数据发送次数.vi" "小时数据发送次数"() -> (w370:i32)
              n223 = global read "全局 小时数据发送次数.vi" "小时数据发送次数"() -> (w519:i32)
              n224 = global read "全局 小时数据发送次数.vi" "小时数据发送次数"() -> (w347:i32)
              n225 = global read "全局 小时数据发送次数.vi" "小时数据发送次数"() -> (w333:i32)
              n226 = global read "全局 小时数据发送次数.vi" "小时数据发送次数"() -> (w340:i32)
              n227 = Index Array(array=w491, index (row)=w492) -> (element=w490:string[])  [unwired: 1 in]
              n228 = Index Array(array=w565, index (row)=w517) -> (element=w547:string[])  [unwired: 1 in]
              n229 = Index Array(array=w566, index (row)=w432) -> (element=w434:string[])  [unwired: 1 in]
              n230 = Index Array(array=w564, index (row)=w424) -> (element=w428:string[])  [unwired: 1 in]
              n231 = Index Array(array=w562, index (row)=w396) -> (element=w420:string[])  [unwired: 1 in]
              n232 = Index Array(array=w563, index (row)=w516) -> (element=w541:string[])  [unwired: 1 in]
              n233 = Index Array(array=w561, index (row)=w397) -> (element=w413:string[])  [unwired: 1 in]
              n234 = Index Array(array=w490, index=0 ("索引")) -> (element=w488:string)
              n235 = Index Array(array=w560, index (row)=w398) -> (element=w412:string[])  [unwired: 1 in]
              n236 = Index Array(array=w558, index (row)=w400) -> (element=w401:string[])  [unwired: 1 in]
              n237 = Index Array(array=w559, index (row)=w399) -> (element=w408:string[])  [unwired: 1 in]
              n238 = Index Array(array=w557, index (row)=w518) -> (element=w534:string[])  [unwired: 1 in]
              n239 = Index Array(array=w547, index #1=3 ("索引"), index #2=5 ("索引")) -> (element #1=w546:string, element #2=w502:string)
              n240 = Index Array(array=w556, index (row)=w519) -> (element=w526:string[])  [unwired: 1 in]
              n241 = Index Array(array=w555, index (row)=w515) -> (element=w524:string[])  [unwired: 1 in]
              n242 = Index Array(array=w444, index (row)=w454) -> (element=w457:string[])  [unwired: 1 in]
              n243 = Index Array(array=w446, index (row)=w470) -> (element=w473:string[])  [unwired: 1 in]
              n244 = Index Array(array=w357, index (row)=w377) -> (element=w374:string[])  [unwired: 1 in]
              n245 = Index Array(array=w445, index (row)=w461) -> (element=w458:string[])  [unwired: 1 in]
              n246 = Index Array(array=w428, index #1=5 ("索引"), index #2=3 ("索引")) -> (element #1=w422:string, element #2=w423:string)
              n247 = Index Array(array=w359, index (row)=w363) -> (element=w360:string[])  [unwired: 1 in]
              n248 = Index Array(array=w358, index (row)=w370) -> (element=w373:string[])  [unwired: 1 in]
              n249 = Index Array(array=w434, index #1=3 ("索引"), index #2=0 ("索引"), index #3=5 ("索引")) -> (element #1=w433:string, element #3=w429:string)  [unwired: 1 out]
              n250 = Index Array(array=w324, index (row)=w347) -> (element=w344:string[])  [unwired: 1 in]
              n251 = Index Array(array=w420, index #1=5 ("索引"), index #2=3 ("索引")) -> (element #1=w393:string, element #2=w394:string)
              n252 = Index Array(array=w326, index (row)=w333) -> (element=w330:string[])  [unwired: 1 in]
              n253 = Index Array(array=w325, index (row)=w340) -> (element=w343:string[])  [unwired: 1 in]
              n254 = Index Array(array=w541, index #1=5 ("索引"), index #2=3 ("索引")) -> (element #1=w501:string, element #2=w500:string)
              n255 = Index Array(array=w413, index #1=5 ("索引"), index #2=3 ("索引")) -> (element #1=w392:string, element #2=w391:string)
              n256 = Index Array(array=w412, index #1=5 ("索引"), index #2=3 ("索引")) -> (element #1=w389:string, element #2=w390:string)
              n257 = Index Array(array=w401, index #1=5 ("索引"), index #2=3 ("索引")) -> (element #1=w385:string, element #2=w386:string)
              n258 = Index Array(array=w408, index #1=5 ("索引"), index #2=3 ("索引")) -> (element #1=w388:string, element #2=w387:string)
              n259 = Index Array(array=w534, index #1=5 ("索引"), index #2=3 ("索引")) -> (element #1=w499:string, element #2=w498:string)
              n260 = Index Array(array=w526, index #1=5 ("索引"), index #2=3 ("索引")) -> (element #1=w497:string, element #2=w496:string)
              n261 = Index Array(array=w524, index #1=5 ("索引"), index #2=3 ("索引")) -> (element #1=w495:string, element #2=w494:string)
              n262 = Index Array(array=w457, index #1=5 ("索引"), index #2=3 ("索引")) -> (element #1=w453:string, element #2=w452:string)
              n263 = Index Array(array=w473, index #1=5 ("索引"), index #2=3 ("索引")) -> (element #1=w469:string, element #2=w468:string)
              n264 = Index Array(array=w374, index #1=5 ("索引"), index #2=3 ("索引")) -> (element #1=w378:string, element #2=w379:string)
              n265 = Index Array(array=w458, index #1=5 ("索引"), index #2=3 ("索引")) -> (element #1=w462:string, element #2=w463:string)
              n266 = Index Array(array=w360, index #1=5 ("索引"), index #2=3 ("索引")) -> (element #1=w364:string, element #2=w365:string)
              n267 = Index Array(array=w373, index #1=5 ("索引"), index #2=3 ("索引")) -> (element #1=w369:string, element #2=w368:string)
              n268 = Index Array(array=w344, index #1=5 ("索引"), index #2=3 ("索引")) -> (element #1=w348:string, element #2=w349:string)
              n269 = Index Array(array=w330, index #1=5 ("索引"), index #2=3 ("索引")) -> (element #1=w334:string, element #2=w335:string)
              n270 = Index Array(array=w343, index #1=5 ("索引"), index #2=3 ("索引")) -> (element #1=w339:string, element #2=w338:string)
              n271 = call "规范时间戳.vi"("字符串"=w488) -> ("result string"=w486:string)  [unwired: 10 in]
              n272 = call "数据编码整合输出.vi"("数据标识"=w502, "数据类型"="-Rtd=", "污染物编码"=w550, "数据值"=w546) -> ("编码输出"=w549:string)  [unwired: 7 in]
              n273 = call "数据编码整合输出.vi"("数据标识"=w422, "数据类型"="-Rtd=", "污染物编码"="w01010", "数据值"=w423) -> ("编码输出"=w545:string)  [unwired: 7 in]
              n274 = call "数据编码整合输出.vi"("数据标识"=w393, "数据类型"="-Rtd=", "污染物编码"="w01009", "数据值"=w394) -> ("编码输出"=w539:string)  [unwired: 7 in]
              n275 = call "数据编码整合输出.vi"("数据标识"=w501, "数据类型"="-Rtd=", "污染物编码"=w543, "数据值"=w500) -> ("编码输出"=w540:string)  [unwired: 7 in]
              n276 = call "数据编码整合输出.vi"("数据标识"=w392, "数据类型"="-Rtd=", "污染物编码"="w01014", "数据值"=w391) -> ("编码输出"=w538:string)  [unwired: 7 in]
              n277 = call "数据编码整合输出.vi"("数据标识"=w389, "数据类型"="-Rtd=", "污染物编码"="w01003", "数据值"=w390) -> ("编码输出"=w537:string)  [unwired: 7 in]
              n278 = call "数据编码整合输出.vi"("数据标识"=w429, "数据类型"="-Rtd=", "污染物编码"="w01019", "数据值"=w433) -> ("编码输出"=w552:string)  [unwired: 7 in]
              n279 = call "数据编码整合输出.vi"("数据标识"=w385, "数据类型"="-Rtd=", "污染物编码"="w19011", "数据值"=w386) -> ("编码输出"=w535:string)  [unwired: 7 in]
              n280 = call "数据编码整合输出.vi"("数据标识"=w388, "数据类型"="-Rtd=", "污染物编码"="w01016", "数据值"=w387) -> ("编码输出"=w536:string)  [unwired: 7 in]
              n281 = call "数据编码整合输出.vi"("数据标识"=w499, "数据类型"="-Rtd=", "污染物编码"=w532, "数据值"=w498) -> ("编码输出"=w530:string)  [unwired: 7 in]
              n282 = call "数据编码整合输出.vi"("数据标识"=w497, "数据类型"="-Rtd=", "污染物编码"=w528, "数据值"=w496) -> ("编码输出"=w525:string)  [unwired: 7 in]
              n283 = call "数据编码整合输出.vi"("数据标识"=w495, "数据类型"="-Rtd=", "污染物编码"=w522, "数据值"=w494) -> ("编码输出"=w520:string)  [unwired: 7 in]
              n284 = call "数据编码整合输出.vi"("数据标识"=w453, "数据类型"="-Rtd=", "污染物编码"="w01100", "数据值"=w452) -> ("编码输出"=w447:string)  [unwired: 7 in]
              n285 = call "数据编码整合输出.vi"("数据标识"=w469, "数据类型"="-Rtd=", "污染物编码"="w21006", "数据值"=w468) -> ("编码输出"=w448:string)  [unwired: 7 in]
              n286 = call "数据编码整合输出.vi"("数据标识"=w378, "数据类型"="-Rtd=", "污染物编码"="w20123", "数据值"=w379) -> ("编码输出"=w353:string)  [unwired: 7 in]
              n287 = call "数据编码整合输出.vi"("数据标识"=w462, "数据类型"="-Rtd=", "污染物编码"="w21019", "数据值"=w463) -> ("编码输出"=w449:string)  [unwired: 7 in]
              n288 = call "数据编码整合输出.vi"("数据标识"=w364, "数据类型"="-Rtd=", "污染物编码"="w20120", "数据值"=w365) -> ("编码输出"=w351:string)  [unwired: 7 in]
              n289 = call "数据编码整合输出.vi"("数据标识"=w369, "数据类型"="-Rtd=", "污染物编码"="w20115", "数据值"=w368) -> ("编码输出"=w352:string)  [unwired: 7 in]
              n290 = call "数据编码整合输出.vi"("数据标识"=w348, "数据类型"="-Rtd=", "污染物编码"="w20111", "数据值"=w349) -> ("编码输出"=w321:string)  [unwired: 7 in]
              n291 = call "数据编码整合输出.vi"("数据标识"=w334, "数据类型"="-Rtd=", "污染物编码"="w20121", "数据值"=w335) -> ("编码输出"=w323:string)  [unwired: 7 in]
              n292 = call "数据编码整合输出.vi"("数据标识"=w339, "数据类型"="-Rtd=", "污染物编码"="w20124", "数据值"=w338) -> ("编码输出"=w322:string)  [unwired: 7 in]
              n293 = Format Into String(format string="DataTime=%s;", w486) -> (resulting string=w485:string)  [unwired: 2 in, 1 out]
              n294 = Format Into String(format string="%s%s%s%s%s%s%s%s%s%s%s%s%s%s%s%s%s%s%s%s%s%s%s%s%s%s%s" ("格式字符串"), w552, w549, w545, w540, w539, w538, w537, w536, w535, w530, w525, w520, w511, w510, w506, w505, w504, w438, w448, w449, w447, w351, w352, w353, w323, w322, w321) -> (resulting string=w484:string)  [unwired: 2 in, 1 out]
              n295 = Concatenate Strings(w485, w484) -> (w441:string)
              n296 = String Length(string=w441) -> (length=w443:i32)
              n297 = Empty String/Path?(string/path=w484) -> (empty?=w514:bool)
              n298 = Decrement(x=w443) -> (x-1=w442:i32)
              n299 = String Subset(string=w441, length (rest)=w442) -> (substring=w440:string)  [unwired: 1 in]
              n300 = case shown="假" w514 {
                tunnel: [w677 ""] -> w554
                tunnel: w440 -> [w677 _]
                frame False {
                  n301 = global read "全局 小时数据发送次数.vi" "小时数据发送次数"() -> (w676:i32)
                  n302 = Increment(x=w676) -> (x+1=w675:i32)
                  n303 = global write "全局 小时数据发送次数.vi" "小时数据发送次数"(w675) -> ()
                }
                frame True {
                  n304 = global read "全局 小时数据发送次数.vi" "小时数据发送次数"() -> (w679:i32)
                  n305 = Increment(x=w679) -> (x+1=w678:i32)
                  n306 = global write "全局 小时数据发送次数.vi" "小时数据发送次数"(w678) -> ()
                }
              }
            }
            frame "返回执行结果" {
            }
          }
        }
        frame "平行样测试" {
          n307 = global read "全局1.vi" "枚举"() -> (w697:enum16{"返回请求应答", "上传数据", "返回执行结果"})
          n308 = case shown="\"上传数据\"" w697 {
            tunnel: ["QnRtn=1" w720 "ExeRtn=1"] -> w696
            tunnel: w695 -> [_ w701 _]
            tunnel: w694 -> [_ w713 _]
            tunnel: w693 -> [_ _ _]
            tunnel: w692 -> [_ _ _]
            tunnel: w691 -> [_ _ _]
            tunnel: w690 -> [_ _ _]
            tunnel: w689 -> [_ _ _]
            tunnel: w688 -> [_ _ _]
            tunnel: w687 -> [_ _ _]
            tunnel: w686 -> [_ w710 _]
            tunnel: w685 -> [_ w708 _]
            tunnel: w684 -> [_ w704 _]
            tunnel: w683 -> [_ _ _]
            tunnel: w682 -> [_ _ _]
            frame "返回请求应答", Default {
            }
            frame "上传数据" {
              # "CODMn"
              n309 = global read "全局 小时数据发送次数.vi" "小时数据发送次数"() -> (w699:i32)
              n310 = Index Array(array=w701, index (row)=w699) -> (element=w718:string[])  [unwired: 1 in]
              n311 = Index Array(array=w718, index=0 ("索引")) -> (element=w715:string)
              n312 = call "规范时间戳.vi"("字符串"=w715) -> ("result string"=w716:string)  [unwired: 10 in]
              n313 = call "平行样集成干预数据组合(子VI).vi"("污染物编码"="w21001", "数据输入"=w708, "小时数据发送次数"=w699) -> ("输出组合"=w706:string)  [unwired: 8 in]
              n314 = call "平行样集成干预数据组合(子VI).vi"("污染物编码"="w01018", "数据输入"=w704, "小时数据发送次数"=w699) -> ("输出组合"=w703:string)  [unwired: 8 in]
              n315 = call "平行样集成干预数据组合(子VI).vi"("污染物编码"="w21011", "数据输入"=w710, "小时数据发送次数"=w699) -> ("输出组合"=w709:string)  [unwired: 8 in]
              n316 = call "平行样集成干预数据组合(子VI).vi"("污染物编码"="w21003", "数据输入"=w713, "小时数据发送次数"=w699) -> ("输出组合"=w712:string)  [unwired: 8 in]
              n317 = call "平行样集成干预数据组合(子VI).vi"("污染物编码"="w01019", "数据输入"=w701, "小时数据发送次数"=w699) -> ("输出组合"=w700:string)  [unwired: 8 in]
              n318 = Empty String/Path?(string/path=w715) -> (empty?=w719:bool)
              n319 = Format Into String(format string="DataTime=%s;%s%s%s%s%s" ("格式字符串"), w716, w700, w712, w709, w706, w703) -> (resulting string=w721:string)  [unwired: 2 in, 1 out]
              n320 = case shown="真" w719 {
                tunnel: [w725 ""] -> w720
                tunnel: w721 -> [w725 _]
                frame False {
                  n321 = global read "全局 小时数据发送次数.vi" "小时数据发送次数"() -> (w724:i32)
                  n322 = Increment(x=w724) -> (x+1=w723:i32)
                  n323 = global write "全局 小时数据发送次数.vi" "小时数据发送次数"(w723) -> ()
                }
                frame True {
                  n324 = global read "全局 小时数据发送次数.vi" "小时数据发送次数"() -> (w727:i32)
                  n325 = Increment(x=w727) -> (x+1=w726:i32)
                  n326 = global write "全局 小时数据发送次数.vi" "小时数据发送次数"(w726) -> ()
                }
              }
            }
            frame "返回执行结果" {
            }
          }
        }
        frame "集成干预测试" {
          n327 = global read "全局1.vi" "枚举"() -> (w748:enum16{"返回请求应答", "上传数据", "返回执行结果"})
          n328 = case shown="\"上传数据\"" w748 {
            tunnel: ["QnRtn=1" w801 "ExeRtn=1"] -> w747
            tunnel: w746 -> [_ w794 _]
            tunnel: w745 -> [_ w791 _]
            tunnel: w744 -> [_ w788 _]
            tunnel: w743 -> [_ w786 _]
            tunnel: w742 -> [_ w782 _]
            tunnel: w741 -> [_ w780 _]
            tunnel: w740 -> [_ w776 _]
            tunnel: w739 -> [_ w773 _]
            tunnel: w738 -> [_ w770 _]
            tunnel: w737 -> [_ w767 _]
            tunnel: w736 -> [_ w764 _]
            tunnel: w735 -> [_ w761 _]
            tunnel: w734 -> [_ _ _]
            tunnel: w733 -> [_ _ _]
            tunnel: w732 -> [_ w759 _]
            tunnel: w731 -> [_ w756 _]
            tunnel: w730 -> [_ w753 _]
            frame "返回请求应答", Default {
            }
            frame "上传数据" {
              # "CODMn"
              n329 = global read "全局 小时数据发送次数.vi" "小时数据发送次数"() -> (w752:i32)
              n330 = Index Array(array=w794, index (row)=w752) -> (element=w799:string[])  [unwired: 1 in]
              n331 = Index Array(array=w799, index=0 ("索引")) -> (element=w796:string)
              n332 = call "规范时间戳.vi"("字符串"=w796) -> ("result string"=w797:string)  [unwired: 10 in]
              n333 = call "平行样集成干预数据组合(子VI).vi"("污染物编码"="w21003", "数据输入"=w791, "小时数据发送次数"=w752) -> ("输出组合"=w790:string)  [unwired: 8 in]
              n334 = call "平行样集成干预数据组合(子VI).vi"("污染物编码"="w01019", "数据输入"=w794, "小时数据发送次数"=w752) -> ("输出组合"=w793:string)  [unwired: 8 in]
              n335 = call "平行样集成干预数据组合(子VI).vi"("污染物编码"="w01010", "数据输入"=w788, "小时数据发送次数"=w752) -> ("输出组合"=w787:string)  [unwired: 8 in]
              n336 = call "平行样集成干预数据组合(子VI).vi"("污染物编码"="w01001", "数据输入"=w786, "小时数据发送次数"=w752) -> ("输出组合"=w784:string)  [unwired: 8 in]
              n337 = call "平行样集成干预数据组合(子VI).vi"("污染物编码"="w01009", "数据输入"=w782, "小时数据发送次数"=w752) -> ("输出组合"=w781:string)  [unwired: 8 in]
              n338 = call "平行样集成干预数据组合(子VI).vi"("污染物编码"="w01003", "数据输入"=w776, "小时数据发送次数"=w752) -> ("输出组合"=w775:string)  [unwired: 8 in]
              n339 = call "平行样集成干预数据组合(子VI).vi"("污染物编码"="w01014", "数据输入"=w780, "小时数据发送次数"=w752) -> ("输出组合"=w778:string)  [unwired: 8 in]
              n340 = call "平行样集成干预数据组合(子VI).vi"("污染物编码"="w21019", "数据输入"=w756, "小时数据发送次数"=w752) -> ("输出组合"=w754:string)  [unwired: 8 in]
              n341 = call "平行样集成干预数据组合(子VI).vi"("污染物编码"="w01100", "数据输入"=w753, "小时数据发送次数"=w752) -> ("输出组合"=w750:string)  [unwired: 8 in]
              n342 = call "平行样集成干预数据组合(子VI).vi"("污染物编码"="w01016", "数据输入"=w773, "小时数据发送次数"=w752) -> ("输出组合"=w772:string)  [unwired: 8 in]
              n343 = call "平行样集成干预数据组合(子VI).vi"("污染物编码"="w19011", "数据输入"=w770, "小时数据发送次数"=w752) -> ("输出组合"=w769:string)  [unwired: 8 in]
              n344 = call "平行样集成干预数据组合(子VI).vi"("污染物编码"="w21001", "数据输入"=w764, "小时数据发送次数"=w752) -> ("输出组合"=w763:string)  [unwired: 8 in]
              n345 = call "平行样集成干预数据组合(子VI).vi"("污染物编码"="w21006", "数据输入"=w759, "小时数据发送次数"=w752) -> ("输出组合"=w757:string)  [unwired: 8 in]
              n346 = call "平行样集成干预数据组合(子VI).vi"("污染物编码"="w01018", "数据输入"=w761, "小时数据发送次数"=w752) -> ("输出组合"=w760:string)  [unwired: 8 in]
              n347 = call "平行样集成干预数据组合(子VI).vi"("污染物编码"="w21011", "数据输入"=w767, "小时数据发送次数"=w752) -> ("输出组合"=w766:string)  [unwired: 8 in]
              n348 = Empty String/Path?(string/path=w796) -> (empty?=w800:bool)
              n349 = Format Into String(format string="DataTime=%s;%s%s%s%s%s%s%s%s%s%s%s%s%s%s%s" ("格式字符串"), w797, w793, w790, w787, w784, w781, w778, w775, w772, w769, w766, w763, w760, w757, w754, w750) -> (resulting string=w802:string)  [unwired: 2 in, 1 out]
              n350 = case shown="真" w800 {
                tunnel: [w806 ""] -> w801
                tunnel: w802 -> [w806 _]
                frame False {
                  n351 = global read "全局 小时数据发送次数.vi" "小时数据发送次数"() -> (w805:i32)
                  n352 = Increment(x=w805) -> (x+1=w804:i32)
                  n353 = global write "全局 小时数据发送次数.vi" "小时数据发送次数"(w804) -> ()
                }
                frame True {
                  n354 = global read "全局 小时数据发送次数.vi" "小时数据发送次数"() -> (w808:i32)
                  n355 = Increment(x=w808) -> (x+1=w807:i32)
                  n356 = global write "全局 小时数据发送次数.vi" "小时数据发送次数"(w807) -> ()
                }
              }
            }
            frame "返回执行结果" {
            }
          }
        }
        frame "加标回收测试" {
          n357 = global read "全局1.vi" "枚举"() -> (w825:enum16{"返回请求应答", "上传数据", "返回执行结果"})
          n358 = case shown="\"上传数据\"" w825 {
            tunnel: ["QnRtn=1" w1048 "ExeRtn=1"] -> w826
            tunnel: w824 -> [_ w1054 _]
            tunnel: w823 -> [_ w1053 _]
            tunnel: w822 -> [_ w1052 _]
            tunnel: w821 -> [_ _ _]
            tunnel: w820 -> [_ _ _]
            tunnel: w819 -> [_ _ _]
            tunnel: w818 -> [_ _ _]
            tunnel: w817 -> [_ _ _]
            tunnel: w816 -> [_ _ _]
            tunnel: w815 -> [_ _ _]
            tunnel: w814 -> [_ w1051 _]
            tunnel: w813 -> [_ w1050 _]
            tunnel: w812 -> [_ _ _]
            tunnel: w811 -> [_ _ _]
            frame "返回请求应答", Default {
            }
            frame "上传数据" {
              # "w01001-Check=63.0,w01001-WaterTime=20160801080000,w01001-Water=45.23,w01001-Chroma=1000,w01001-Volume=0.2,w01001-DVolume=200,w01003-Flag=N;"
              # "CODCr"
              # "总氮"
              # "总磷"
              # "NH3"
              # "CODMn"
              n359 = global read "全局 小时数据发送次数.vi" "小时数据发送次数"() -> (w1055:i32)
              n360 = Index Array(array=w1053, index (row)=w1055) -> (element=w1060:string[])  [unwired: 1 in]
              n361 = Index Array(array=w1050, index (row)=w1055) -> (element=w1062:string[])  [unwired: 1 in]
              n362 = Index Array(array=w1051, index (row)=w1055) -> (element=w1064:string[])  [unwired: 1 in]
              n363 = Index Array(array=w1060, index #1=4 ("索引"), index #2=2 ("索引"), index #3=3 ("索引"), index #4=5 ("索引"), index #5=6 ("索引"), index #6=7 ("索引")) -> (element #1=w949:string, element #2=w843:string, element #3=w934:string, element #4=w933:string, element #5=w932:string, element #6=w931:string)
              n364 = Index Array(array=w1052, index (row)=w1055) -> (element=w1061:string[])  [unwired: 1 in]
              n365 = Index Array(array=w1054, index (row)=w1055) -> (element=w1059:string[])  [unwired: 1 in]
              n366 = Index Array(array=w1064, index #1=4 ("索引"), index #2=2 ("索引"), index #3=3 ("索引"), index #4=5 ("索引"), index #5=6 ("索引"), index #6=7 ("索引")) -> (element #1=w1019:string, element #2=w847:string, element #3=w999:string, element #4=w998:string, element #5=w997:string, element #6=w996:string)
              n367 = Index Array(array=w1062, index #1=0 ("索引"), index #2=4 ("索引"), index #3=2 ("索引"), index #4=3 ("索引"), index #5=5 ("索引"), index #6=6 ("索引"), index #7=7 ("索引")) -> (element #1=w1057:string, element #2=w1045:string, element #3=w869:string, element #4=w1037:string, element #5=w1034:string, element #6=w1030:string, element #7=w1029:string)
              n368 = Index Array(array=w1061, index #1=4 ("索引"), index #2=2 ("索引"), index #3=3 ("索引"), index #4=5 ("索引"), index #5=6 ("索引"), index #6=7 ("索引")) -> (element #1=w977:string, element #2=w845:string, element #3=w954:string, element #4=w953:string, element #5=w952:string, element #6=w951:string)
              n369 = Index Array(array=w1059, index #1=4 ("索引"), index #2=2 ("索引"), index #3=3 ("索引"), index #4=5 ("索引"), index #5=6 ("索引"), index #6=7 ("索引")) -> (element #1=w947:string, element #2=w841:string, element #3=w884:string, element #4=w885:string, element #5=w886:string, element #6=w887:string)
              n370 = call "规范时间戳.vi"("字符串"=w1057) -> ("result string"=w1056:string)  [unwired: 10 in]
              n371 = call "规范时间戳.vi"("字符串"=w869) -> ("result string"=w868:string)  [unwired: 10 in]
              n372 = call "规范时间戳.vi"("字符串"=w843) -> ("result string"=w842:string)  [unwired: 10 in]
              n373 = call "规范时间戳.vi"("字符串"=w845) -> ("result string"=w844:string)  [unwired: 10 in]
              n374 = call "规范时间戳.vi"("字符串"=w847) -> ("result string"=w846:string)  [unwired: 10 in]
              n375 = call "规范时间戳.vi"("字符串"=w841) -> ("result string"=w840:string)  [unwired: 10 in]
              n376 = call "核查数据编码整合输出.vi"("字段结束"=FALSE, "数据标识"="N" ("字符串"), "数据类型"="-Check=", "污染物编码"="w21011", "数据值"=w977) -> ("编码输出"=w976:string)  [unwired: 6 in]
              n377 = call "核查数据编码整合输出.vi"("字段结束"=FALSE, "数据标识"="N" ("字符串"), "数据类型"="-WaterTime=", "污染物编码"="w21011", "数据值"=w844) -> ("编码输出"=w959:string)  [unwired: 6 in]
              n378 = call "核查数据编码整合输出.vi"("字段结束"=FALSE, "数据标识"="N" ("字符串"), "数据类型"="-Water=", "污染物编码"="w21011", "数据精度"=2, "数据值"=w954) -> ("编码输出"=w958:string)  [unwired: 5 in]
              n379 = call "核查数据编码整合输出.vi"("字段结束"=TRUE, "数据标识"="N" ("字符串"), "数据类型"="-DVolume=", "污染物编码"="w21011", "数据值"=w951) -> ("编码输出"=w955:string)  [unwired: 6 in]
              n380 = call "核查数据编码整合输出.vi"("字段结束"=FALSE, "数据标识"="N" ("字符串"), "数据类型"="-Chroma=", "污染物编码"="w21011", "数据值"=w953) -> ("编码输出"=w957:string)  [unwired: 6 in]
              n381 = call "核查数据编码整合输出.vi"("字段结束"=FALSE, "数据标识"="N" ("字符串"), "数据类型"="-Volume=", "污染物编码"="w21011", "数据值"=w952) -> ("编码输出"=w956:string)  [unwired: 6 in]
              n382 = call "核查数据编码整合输出.vi"("字段结束"=FALSE, "数据标识"="N" ("字符串"), "数据类型"="-WaterTime=", "污染物编码"="w21001", "数据值"=w842) -> ("编码输出"=w929:string)  [unwired: 6 in]
              n383 = call "核查数据编码整合输出.vi"("字段结束"=FALSE, "数据类型"="-Volume=", "污染物编码"="w01019", "数据值"=w1030) -> ("编码输出"=w1022:string)  [unwired: 7 in]
              n384 = call "核查数据编码整合输出.vi"("字段结束"=FALSE, "数据标识"="N" ("字符串"), "数据类型"="-Check=", "污染物编码"="w21001", "数据值"=w949) -> ("编码输出"=w930:string)  [unwired: 6 in]
              n385 = call "核查数据编码整合输出.vi"("字段结束"=FALSE, "数据标识"="N" ("字符串"), "数据类型"="-Water=", "污染物编码"="w21001", "数据精度"=2, "数据值"=w934) -> ("编码输出"=w928:string)  [unwired: 5 in]
              n386 = call "核查数据编码整合输出.vi"("字段结束"=FALSE, "数据标识"="N" ("字符串"), "数据类型"="-Chroma=", "污染物编码"="w21001", "数据值"=w933) -> ("编码输出"=w927:string)  [unwired: 6 in]
              n387 = call "核查数据编码整合输出.vi"("字段结束"=FALSE, "数据标识"="N" ("字符串"), "数据类型"="-Volume=", "污染物编码"="w21001", "数据值"=w932) -> ("编码输出"=w926:string)  [unwired: 6 in]
              n388 = call "核查数据编码整合输出.vi"("字段结束"=TRUE, "数据标识"="N" ("字符串"), "数据类型"="-DVolume=", "污染物编码"="w21001", "数据值"=w931) -> ("编码输出"=w925:string)  [unwired: 6 in]
              n389 = call "核查数据编码整合输出.vi"("字段结束"=TRUE, "数据类型"="-DVolume=", "污染物编码"="w01019", "数据值"=w1029) -> ("编码输出"=w1021:string)  [unwired: 7 in]
              n390 = call "核查数据编码整合输出.vi"("字段结束"=FALSE, "数据类型"="-Chroma=", "污染物编码"="w01019", "数据值"=w1034) -> ("编码输出"=w1023:string)  [unwired: 7 in]
              n391 = call "核查数据编码整合输出.vi"("字段结束"=FALSE, "数据标识"="N" ("字符串"), "数据类型"="-Check=", "污染物编码"="w21003", "数据值"=w1019) -> ("编码输出"=w990:string)  [unwired: 6 in]
              n392 = call "核查数据编码整合输出.vi"("字段结束"=FALSE, "数据标识"="N" ("字符串"), "数据类型"="-WaterTime=", "污染物编码"="w21003", "数据值"=w846) -> ("编码输出"=w989:string)  [unwired: 6 in]
              n393 = call "核查数据编码整合输出.vi"("字段结束"=FALSE, "数据标识"="N" ("字符串"), "数据类型"="-Check=", "污染物编码"="w01019", "数据值"=w1045) -> ("编码输出"=w1026:string)  [unwired: 6 in]
              n394 = call "核查数据编码整合输出.vi"("字段结束"=FALSE, "数据类型"="-WaterTime=", "污染物编码"="w01019", "数据值"=w868) -> ("编码输出"=w1025:string)  [unwired: 7 in]
              n395 = call "核查数据编码整合输出.vi"("字段结束"=FALSE, "数据标识"="N" ("字符串"), "数据类型"="-Water=", "污染物编码"="w21003", "数据精度"=2, "数据值"=w999) -> ("编码输出"=w988:string)  [unwired: 5 in]
              n396 = call "核查数据编码整合输出.vi"("字段结束"=FALSE, "数据类型"="-Water=", "污染物编码"="w01019", "数据精度"=2, "数据值"=w1037) -> ("编码输出"=w1024:string)  [unwired: 6 in]
              n397 = call "核查数据编码整合输出.vi"("字段结束"=FALSE, "数据标识"="N" ("字符串"), "数据类型"="-Chroma=", "污染物编码"="w21003", "数据值"=w998) -> ("编码输出"=w987:string)  [unwired: 6 in]
              n398 = call "核查数据编码整合输出.vi"("字段结束"=FALSE, "数据标识"="N" ("字符串"), "数据类型"="-Volume=", "污染物编码"="w21003", "数据值"=w997) -> ("编码输出"=w986:string)  [unwired: 6 in]
              n399 = call "核查数据编码整合输出.vi"("字段结束"=TRUE, "数据标识"="N" ("字符串"), "数据类型"="-DVolume=", "污染物编码"="w21003", "数据值"=w996) -> ("编码输出"=w985:string)  [unwired: 6 in]
              n400 = call "核查数据编码整合输出.vi"("字段结束"=FALSE, "数据标识"="N" ("字符串"), "数据类型"="-Check=", "污染物编码"="w01018", "数据值"=w947) -> ("编码输出"=w902:string)  [unwired: 6 in]
              n401 = call "核查数据编码整合输出.vi"("字段结束"=FALSE, "数据标识"="N" ("字符串"), "数据类型"="-Water=", "污染物编码"="w01018", "数据精度"=2, "数据值"=w884) -> ("编码输出"=w900:string)  [unwired: 5 in]
              n402 = call "核查数据编码整合输出.vi"("字段结束"=FALSE, "数据标识"="N" ("字符串"), "数据类型"="-WaterTime=", "污染物编码"="w01018", "数据值"=w840) -> ("编码输出"=w901:string)  [unwired: 6 in]
              n403 = call "核查数据编码整合输出.vi"("字段结束"=FALSE, "数据标识"="N" ("字符串"), "数据类型"="-Chroma=", "污染物编码"="w01018", "数据值"=w885) -> ("编码输出"=w899:string)  [unwired: 6 in]
              n404 = call "核查数据编码整合输出.vi"("字段结束"=FALSE, "数据标识"="N" ("字符串"), "数据类型"="-Volume=", "污染物编码"="w01018", "数据值"=w886) -> ("编码输出"=w898:string)  [unwired: 6 in]
              n405 = call "核查数据编码整合输出.vi"("字段结束"=TRUE, "数据标识"="N" ("字符串"), "数据类型"="-DVolume=", "污染物编码"="w01018", "数据值"=w887) -> ("编码输出"=w897:string)  [unwired: 6 in]
              n406 = Concatenate Strings(w976, w959, w958, w957, w956, w955) -> (w945:string)
              n407 = Concatenate Strings(w1026, w1025, w1024, w1023, w1022, w1021) -> (w1020:string)
              n408 = Concatenate Strings(w990, w989, w988, w987, w986, w985) -> (w984:string)
              n409 = Concatenate Strings(w930, w929, w928, w927, w926, w925) -> (w880:string)
              n410 = Empty String/Path?(string/path=w1056) -> (empty?=w1047:bool)
              n411 = Concatenate Strings(w902, w901, w900, w899, w898, w897) -> (w879:string)
              n412 = Format Into String(format string="DataTime=%s;%s%s%s%s%s" ("格式字符串"), w1056, w1020, w984, w945, w880, w879) -> (resulting string=w1049:string)  [unwired: 2 in, 1 out]
              n413 = case shown="真" w1047 {
                tunnel: [w1068 ""] -> w1048
                tunnel: w1049 -> [w1068 _]
                frame False {
                  n414 = global read "全局 小时数据发送次数.vi" "小时数据发送次数"() -> (w1067:i32)
                  n415 = Increment(x=w1067) -> (x+1=w1066:i32)
                  n416 = global write "全局 小时数据发送次数.vi" "小时数据发送次数"(w1066) -> ()
                }
                frame True {
                  n417 = global read "全局 小时数据发送次数.vi" "小时数据发送次数"() -> (w1070:i32)
                  n418 = Increment(x=w1070) -> (x+1=w1069:i32)
                  n419 = global write "全局 小时数据发送次数.vi" "小时数据发送次数"(w1069) -> ()
                }
              }
            }
            frame "返回执行结果" {
            }
          }
        }
        frame "核查数据" {
          n420 = global read "全局1.vi" "枚举"() -> (w1087:enum16{"返回请求应答", "上传数据", "返回执行结果"})
          n421 = case shown="\"上传数据\"" w1087 {
            tunnel: ["QnRtn=1" w1135 "ExeRtn=1"] -> w1088
            tunnel: w1086 -> [_ w1128 _]
            tunnel: w1085 -> [_ w1133 _]
            tunnel: w1084 -> [_ w1125 _]
            tunnel: w1083 -> [_ w1122 _]
            tunnel: w1082 -> [_ w1119 _]
            tunnel: w1081 -> [_ w1116 _]
            tunnel: w1080 -> [_ w1113 _]
            tunnel: w1079 -> [_ w1110 _]
            tunnel: w1078 -> [_ w1107 _]
            tunnel: w1077 -> [_ w1095 _]
            tunnel: w1076 -> [_ w1092 _]
            tunnel: w1075 -> [_ w1104 _]
            tunnel: w1074 -> [_ w1101 _]
            tunnel: w1073 -> [_ w1098 _]
            frame "返回请求应答", Default {
            }
            frame "上传数据" {
              # "将非空数组的时间戳写入"
              n422 = global read "全局 小时数据发送次数.vi" "小时数据发送次数"() -> (w1091:i32)
              n423 = Index Array(array=w1128, index (row)=w1091) -> (element=w1134:string[])  [unwired: 1 in]
              n424 = Index Array(array=w1134, index=0 ("索引")) -> (element=w1132:string)
              n425 = call "规范分钟数据时间戳.vi"("字符串"=w1132) -> ("result string"=w1131:string)  [unwired: 10 in]
              n426 = call "标样核查数据组合(子VI).vi"("小时数据发送次数"=w1091, "数据输入"=w1098, "污染物编码"="w21006") -> ("输出组合"=w1097:string)  [unwired: 8 in]
              n427 = call "标样核查数据组合(子VI).vi"("小时数据发送次数"=w1091, "数据输入"=w1128, "污染物编码"="w01019") -> ("输出组合"=w1127:string)  [unwired: 8 in]
              n428 = call "标样核查数据组合(子VI).vi"("小时数据发送次数"=w1091, "数据输入"=w1104, "污染物编码"="w01100") -> ("输出组合"=w1103:string)  [unwired: 8 in]
              n429 = call "标样核查数据组合(子VI).vi"("小时数据发送次数"=w1091, "数据输入"=w1101, "污染物编码"="w21019") -> ("输出组合"=w1100:string)  [unwired: 8 in]
              n430 = call "标样核查数据组合(子VI).vi"("小时数据发送次数"=w1091, "数据输入"=w1092, "污染物编码"="w19011") -> ("输出组合"=w1090:string)  [unwired: 8 in]
              n431 = call "标样核查数据组合(子VI).vi"("小时数据发送次数"=w1091, "数据输入"=w1133, "污染物编码"="w21003") -> ("输出组合"=w1136:string)  [unwired: 8 in]
              n432 = call "标样核查数据组合(子VI).vi"("小时数据发送次数"=w1091, "数据输入"=w1095, "污染物编码"="w01016") -> ("输出组合"=w1094:string)  [unwired: 8 in]
              n433 = call "标样核查数据组合(子VI).vi"("小时数据发送次数"=w1091, "数据输入"=w1125, "污染物编码"="w21011") -> ("输出组合"=w1124:string)  [unwired: 8 in]
              n434 = call "标样核查数据组合(子VI).vi"("小时数据发送次数"=w1091, "数据输入"=w1122, "污染物编码"="w21001") -> ("输出组合"=w1121:string)  [unwired: 8 in]
              n435 = call "标样核查数据组合(子VI).vi"("小时数据发送次数"=w1091, "数据输入"=w1119, "污染物编码"="w01018") -> ("输出组合"=w1118:string)  [unwired: 8 in]
              n436 = call "标样核查数据组合(子VI).vi"("小时数据发送次数"=w1091, "数据输入"=w1116, "污染物编码"="w01001") -> ("输出组合"=w1115:string)  [unwired: 8 in]
              n437 = call "标样核查数据组合(子VI).vi"("小时数据发送次数"=w1091, "数据输入"=w1113, "污染物编码"="w01009") -> ("输出组合"=w1112:string)  [unwired: 8 in]
              n438 = call "标样核查数据组合(子VI).vi"("小时数据发送次数"=w1091, "数据输入"=w1110, "污染物编码"="w01014") -> ("输出组合"=w1109:string)  [unwired: 8 in]
              n439 = call "标样核查数据组合(子VI).vi"("小时数据发送次数"=w1091, "数据输入"=w1107, "污染物编码"="w01003") -> ("输出组合"=w1106:string)  [unwired: 8 in]
              n440 = Format Into String(format string="DataTime=%s;%s%s%s%s%s%s%s%s%s%s%s%s%s%s" ("格式字符串"), w1131, w1127, w1136, w1124, w1121, w1118, w1115, w1112, w1109, w1106, w1094, w1090, w1097, w1100, w1103) -> (resulting string=w1137:string)  [unwired: 2 in, 1 out]
              n441 = Empty String/Path?(string/path=w1131) -> (empty?=w1138:bool)
              n442 = case shown="假" w1138 {
                tunnel: [w1143 ""] -> w1135
                tunnel: w1137 -> [w1143 _]
                frame False {
                  n443 = global read "全局 小时数据发送次数.vi" "小时数据发送次数"() -> (w1142:i32)
                  n444 = Increment(x=w1142) -> (x+1=w1141:i32)
                  n445 = global write "全局 小时数据发送次数.vi" "小时数据发送次数"(w1141) -> ()
                }
                frame True {
                  n446 = global read "全局 小时数据发送次数.vi" "小时数据发送次数"() -> (w1145:i32)
                  n447 = Increment(x=w1145) -> (x+1=w1144:i32)
                  n448 = global write "全局 小时数据发送次数.vi" "小时数据发送次数"(w1144) -> ()
                }
              }
            }
            frame "返回执行结果" {
            }
          }
        }
        frame "空白测试", "跨度核查" {
          n449 = global read "全局1.vi" "枚举"() -> (w1156:enum16{"返回请求应答", "上传数据", "返回执行结果"})
          n450 = case shown="\"上传数据\"" w1156 {
            tunnel: ["QnRtn=1" w1221 "ExeRtn=1"] -> w1157
            tunnel: w1155 -> [_ w1227 _]
            tunnel: w1154 -> [_ w1226 _]
            tunnel: w1153 -> [_ w1225 _]
            tunnel: w1152 -> [_ w1224 _]
            tunnel: w1151 -> [_ w1223 _]
            tunnel: w1150 -> [_ w1198 _]
            tunnel: w1149 -> [_ w1197 _]
            tunnel: w1148 -> [_ w1196 _]
            frame "返回请求应答", Default {
            }
            frame "上传数据" {
              n451 = global read "全局 小时数据发送次数.vi" "小时数据发送次数"() -> (w1214:i32)
              n452 = global read "全局 小时数据发送次数.vi" "小时数据发送次数"() -> (w1215:i32)
              n453 = global read "全局 小时数据发送次数.vi" "小时数据发送次数"() -> (w1218:i32)
              n454 = global read "全局 小时数据发送次数.vi" "小时数据发送次数"() -> (w1217:i32)
              n455 = global read "全局 小时数据发送次数.vi" "小时数据发送次数"() -> (w1201:i32)
              n456 = global read "全局 小时数据发送次数.vi" "小时数据发送次数"() -> (w1200:i32)
              n457 = global read "全局 小时数据发送次数.vi" "小时数据发送次数"() -> (w1216:i32)
              n458 = global read "全局 小时数据发送次数.vi" "小时数据发送次数"() -> (w1199:i32)
              n459 = Index Array(array=w1226, index (row)=w1215) -> (element=w1243:string[])  [unwired: 1 in]
              n460 = Index Array(array=w1227, index (row)=w1214) -> (element=w1241:string[])  [unwired: 1 in]
              n461 = Index Array(array=w1224, index (row)=w1218) -> (element=w1237:string[])  [unwired: 1 in]
              n462 = Index Array(array=w1223, index (row)=w1217) -> (element=w1236:string[])  [unwired: 1 in]
              n463 = Index Array(array=w1197, index (row)=w1201) -> (element=w1207:string[])  [unwired: 1 in]
              n464 = Index Array(array=w1196, index (row)=w1200) -> (element=w1206:string[])  [unwired: 1 in]
              n465 = Index Array(array=w1225, index (row)=w1216) -> (element=w1240:string[])  [unwired: 1 in]
              n466 = Index Array(array=w1198, index (row)=w1199) -> (element=w1210:string[])  [unwired: 1 in]
              n467 = Index Array(array=w1243, index #1=3 ("索引"), index #2=7 ("索引")) -> (element #1=w1192:string, element #2=w1191:string)
              n468 = Index Array(array=w1241, index #1=0 ("索引"), index #2=3 ("索引"), index #3=7 ("索引")) -> (element #1=w1212:string, element #2=w1213:string, element #3=w1219:string)
              n469 = Index Array(array=w1237, index #1=3 ("索引"), index #2=7 ("索引")) -> (element #1=w1182:string, element #2=w1181:string)
              n470 = Index Array(array=w1236, index #1=3 ("索引"), index #2=7 ("索引")) -> (element #1=w1177:string, element #2=w1176:string)
              n471 = Index Array(array=w1207, index #1=3 ("索引"), index #2=7 ("索引")) -> (element #1=w1167:string, element #2=w1166:string)
              n472 = Index Array(array=w1206, index #1=3 ("索引"), index #2=7 ("索引")) -> (element #1=w1163:string, element #2=w1162:string)
              n473 = Index Array(array=w1240, index #1=3 ("索引"), index #2=7 ("索引")) -> (element #1=w1187:string, element #2=w1186:string)
              n474 = Index Array(array=w1210, index #1=3 ("索引"), index #2=7 ("索引")) -> (element #1=w1172:string, element #2=w1171:string)
              n475 = call "规范小时时间戳.vi"("字符串"=w1212) -> ("result string"=w1211:string)  [unwired: 10 in]
              n476 = call "零点跨度数据组合 (子VI).vi"("span value"="0", "standard value"=w1162, "check value"=w1163, "污染物编码"="w01100") -> ("组合输出"=w1159:string)  [unwired: 7 in]
              n477 = call "零点跨度数据组合 (子VI).vi"("span value"="0", "standard value"=w1166, "check value"=w1167, "污染物编码"="w21019") -> ("组合输出"=w1165:string)  [unwired: 7 in]
              n478 = call "零点跨度数据组合 (子VI).vi"("span value"="0", "standard value"=w1191, "check value"=w1192, "污染物编码"="w21003") -> ("组合输出"=w1189:string)  [unwired: 7 in]
              n479 = call "零点跨度数据组合 (子VI).vi"("span value"="0", "standard value"=w1219, "check value"=w1213, "污染物编码"="w01019") -> ("组合输出"=w1233:string)  [unwired: 7 in]
              n480 = call "零点跨度数据组合 (子VI).vi"("span value"="0", "standard value"=w1186, "check value"=w1187, "污染物编码"="w21011") -> ("组合输出"=w1185:string)  [unwired: 7 in]
              n481 = call "零点跨度数据组合 (子VI).vi"("span value"="0", "standard value"=w1181, "check value"=w1182, "污染物编码"="w21001") -> ("组合输出"=w1180:string)  [unwired: 7 in]
              n482 = call "零点跨度数据组合 (子VI).vi"("span value"="0", "standard value"=w1176, "check value"=w1177, "污染物编码"="w01018") -> ("组合输出"=w1175:string)  [unwired: 7 in]
              n483 = call "零点跨度数据组合 (子VI).vi"("span value"="0", "standard value"=w1171, "check value"=w1172, "污染物编码"="w21006") -> ("组合输出"=w1170:string)  [unwired: 7 in]
              n484 = Format Into String(format string="DataTime=%s;%s%s%s%s%s%s%s%s" ("格式字符串"), w1211, w1233, w1189, w1185, w1180, w1175, w1170, w1165, w1159) -> (resulting string=w1220:string)  [unwired: 2 in, 1 out]
              n485 = Empty String/Path?(string/path=w1211) -> (empty?=w1222:bool)
              n486 = case shown="假" w1222 {
                tunnel: [w1246 ""] -> w1221
                tunnel: w1220 -> [w1246 _]
                frame False {
                  n487 = global read "全局 小时数据发送次数.vi" "小时数据发送次数"() -> (w1248:i32)
                  n488 = Increment(x=w1248) -> (x+1=w1247:i32)
                  n489 = global write "全局 小时数据发送次数.vi" "小时数据发送次数"(w1247) -> ()
                }
                frame True {
                  n490 = global read "全局 小时数据发送次数.vi" "小时数据发送次数"() -> (w1250:i32)
                  n491 = Increment(x=w1250) -> (x+1=w1249:i32)
                  n492 = global write "全局 小时数据发送次数.vi" "小时数据发送次数"(w1249) -> ()
                }
              }
            }
            frame "返回执行结果" {
            }
          }
        }
      }
    }
    frame "小时数据" {
      # "藻密度"
      # "叶绿素"
      # "浊度"
      # "水温"
      # "发送小时数据"
      n493 = global read "全局 小时数据发送次数.vi" "小时数据发送次数"() -> (w1307:i32)
      n494 = global read "全局 小时数据发送次数.vi" "小时数据发送次数"() -> (w1308:i32)
      n495 = global read "全局 小时数据发送次数.vi" "小时数据发送次数"() -> (w1295:i32)
      n496 = global read "全局 小时数据发送次数.vi" "小时数据发送次数"() -> (w1291:i32)
      n497 = global read "全局 小时数据发送次数.vi" "小时数据发送次数"() -> (w1311:i32)
      n498 = global read "全局 小时数据发送次数.vi" "小时数据发送次数"() -> (w1290:i32)
      n499 = global read "全局 小时数据发送次数.vi" "小时数据发送次数"() -> (w1289:i32)
      n500 = global read "全局 小时数据发送次数.vi" "小时数据发送次数"() -> (w1288:i32)
      n501 = global read "全局 小时数据发送次数.vi" "小时数据发送次数"() -> (w1297:i32)
      n502 = global read "全局 小时数据发送次数.vi" "小时数据发送次数"() -> (w1317:i32)
      n503 = global read "全局 小时数据发送次数.vi" "小时数据发送次数"() -> (w1303:i32)
      n504 = global read "全局 小时数据发送次数.vi" "小时数据发送次数"() -> (w1315:i32)
      n505 = global read "全局 小时数据发送次数.vi" "小时数据发送次数"() -> (w1300:i32)
      n506 = global read "全局 小时数据发送次数.vi" "小时数据发送次数"() -> (w1269:i32)
      n507 = global read "全局 小时数据发送次数.vi" "小时数据发送次数"() -> (w1270:i32)
      n508 = global read "全局 小时数据发送次数.vi" "小时数据发送次数"() -> (w1278:i32)
      n509 = global read "全局 小时数据发送次数.vi" "小时数据发送次数"() -> (w1268:i32)
      n510 = global read "全局 小时数据发送次数.vi" "小时数据发送次数"() -> (w1277:i32)
      n511 = global read "全局 小时数据发送次数.vi" "小时数据发送次数"() -> (w1319:i32)
      n512 = global read "全局 小时数据发送次数.vi" "小时数据发送次数"() -> (w1279:i32)
      n513 = global read "全局 小时数据发送次数.vi" "小时数据发送次数"() -> (w1305:i32)
      n514 = global read "全局 小时数据发送次数.vi" "小时数据发送次数"() -> (w1313:i32)
      n515 = global read "全局 小时数据发送次数.vi" "小时数据发送次数"() -> (w1260:i32)
      n516 = global read "全局 小时数据发送次数.vi" "小时数据发送次数"() -> (w1259:i32)
      n517 = global read "全局 小时数据发送次数.vi" "小时数据发送次数"() -> (w1261:i32)
      n518 = global read "全局 小时数据发送次数.vi" "小时数据发送次数"() -> (w1301:i32)
      n519 = global read "全局 小时数据发送次数.vi" "小时数据发送次数"() -> (w1321:i32)
      n520 = Index Array(array=w1267, index (row)=w1270) -> (element=w1264:string[])  [unwired: 1 in]
      n521 = Index Array(array=w1276, index (row)=w1277) -> (element=w1273:string[])  [unwired: 1 in]
      n522 = Index Array(array=w1265, index (row)=w1269) -> (element=w1262:string[])  [unwired: 1 in]
      n523 = Index Array(array=w1274, index (row)=w1278) -> (element=w1271:string[])  [unwired: 1 in]
      n524 = Index Array(array=w1266, index (row)=w1268) -> (element=w1263:string[])  [unwired: 1 in]
      n525 = Index Array(array=w1275, index (row)=w1279) -> (element=w1272:string[])  [unwired: 1 in]
      n526 = Index Array(array=w1258, index (row)=w1259) -> (element=w1255:string[])  [unwired: 1 in]
      n527 = Index Array(array=w1328, index (row)=w1308) -> (element=w1309:string[])  [unwired: 1 in]
      n528 = Index Array(array=w1292, index (row)=w1295) -> (element=w1294:string[])  [unwired: 1 in]
      n529 = Index Array(array=w1283, index (row)=w1291) -> (element=w1287:string[])  [unwired: 1 in]
      n530 = Index Array(array=w1329, index (row)=w1311) -> (element=w1310:string[])  [unwired: 1 in]
      n531 = Index Array(array=w1282, index (row)=w1290) -> (element=w1286:string[])  [unwired: 1 in]
      n532 = Index Array(array=w1281, index (row)=w1289) -> (element=w1285:string[])  [unwired: 1 in]
      n533 = Index Array(array=w1280, index (row)=w1288) -> (element=w1284:string[])  [unwired: 1 in]
      n534 = Index Array(array=w1256, index (row)=w1260) -> (element=w1253:string[])  [unwired: 1 in]
      n535 = Index Array(array=w1293, index (row)=w1297) -> (element=w1296:string[])  [unwired: 1 in]
      n536 = Index Array(array=w1257, index (row)=w1261) -> (element=w1254:string[])  [unwired: 1 in]
      n537 = Index Array(array=w1333, index (row)=w1319) -> (element=w1318:string[])  [unwired: 1 in]
      n538 = Index Array(array=w1332, index (row)=w1317) -> (element=w1316:string[])  [unwired: 1 in]
      n539 = Index Array(array=w1331, index (row)=w1315) -> (element=w1314:string[])  [unwired: 1 in]
      n540 = Index Array(array=w1334, index (row)=w1321) -> (element=w1320:string[])  [unwired: 1 in]
      n541 = Index Array(array=w1327, index (row)=w1307) -> (element=w1306:string[])  [unwired: 1 in]
      n542 = Index Array(array=w1325, index (row)=w1303) -> (element=w1302:string[])  [unwired: 1 in]
      n543 = Index Array(array=w1326, index (row)=w1305) -> (element=w1304:string[])  [unwired: 1 in]
      n544 = Index Array(array=w1330, index (row)=w1313) -> (element=w1312:string[])  [unwired: 1 in]
      n545 = Index Array(array=w1323, index (row)=w1300) -> (element=w1298:string[])  [unwired: 1 in]
      n546 = Index Array(array=w1324, index (row)=w1301) -> (element=w1299:string[])  [unwired: 1 in]
      n547 = global read "全局1.vi" "枚举"() -> (w1322:enum16{"返回请求应答", "上传数据", "返回执行结果"})
      n548 = case shown="\"上传数据\"" w1322 {
        tunnel: ["QnRtn=1" w1563 "ExeRtn=1"] -> w1335
        tunnel: w1320 -> [_ w1590 _]
        tunnel: w1316 -> [_ w1604 _]
        tunnel: w1314 -> [_ w1603 _]
        tunnel: w1312 -> [_ w1602 _]
        tunnel: w1318 -> [_ w1600 _]
        tunnel: w1310 -> [_ w1589 _]
        tunnel: w1309 -> [_ w1595 _]
        tunnel: w1306 -> [_ w1592 _]
        tunnel: w1304 -> [_ w1591 _]
        tunnel: w1302 -> [_ w1588 _]
        tunnel: w1299 -> [_ w1587 _]
        tunnel: w1298 -> [_ w1586 _]
        tunnel: w1296 -> [_ w1568 _]
        tunnel: w1294 -> [_ w1567 _]
        tunnel: w1287 -> [_ w1562 _]
        tunnel: w1286 -> [_ w1561 _]
        tunnel: w1285 -> [_ w1560 _]
        tunnel: w1284 -> [_ w1559 _]
        tunnel: w1273 -> [_ w1480 _]
        tunnel: w1272 -> [_ w1479 _]
        tunnel: w1271 -> [_ w1478 _]
        tunnel: w1264 -> [_ w1380 _]
        tunnel: w1263 -> [_ w1379 _]
        tunnel: w1262 -> [_ w1378 _]
        tunnel: w1255 -> [_ w1347 _]
        tunnel: w1254 -> [_ w1346 _]
        tunnel: w1253 -> [_ w1345 _]
        frame "返回请求应答", Default {
          (unwired) 0 ("当前包数")
          n549 = global read "全局 数据数组大小.vi" "数据数组大小"() -> (w1336:i32)
          n550 = global write "全局1.vi" "枚举"(enum16{"返回请求应答", "上传数据", "返回执行结果"}."上传数据" ("枚举")) -> ()
          n551 = Equal To 0?(x=w1336) -> (x = 0?=w1337:bool)
          n552 = case shown="真" w1337 {
            frame False {
            }
            frame True {
              n553 = global read "全局 小时数据发送次数.vi" "小时数据发送次数"() -> (w1341:i32)
              n554 = Increment(x=w1341) -> (x+1=w1340:i32)
              n555 = global write "全局 小时数据发送次数.vi" "小时数据发送次数"(w1340) -> ()
            }
          }
        }
        frame "上传数据" {
          (unwired) 2 ("数据精度")
          (unwired) 3 ("数据精度")
          (unwired) 3 ("数据精度")
          (unwired) 3 ("数据精度")
          # "汞"
          # "锰"
          # "镍"
          # "锌"
          # "镉"
          # "铅"
          # "藻密度"
          # "叶绿素"
          # "浊度"
          # "电导率"
          # "DO"
          # "水温"
          # "CODMn"
          # "ORP"
          # "硫化物"
          # "亚硝酸盐"
          # "PH"
          # "总氮"
          # "总磷"
          # "CODCr"
          # "NH3"
          n556 = global read "断电保存全局.vi" "数据发送协议"() -> (w1513:enum16{"2005-212协议", "2017-212协议"})
          n557 = case shown="\"2017-212协议\", 默认" w1513 {
            tunnel: w1568 -> [_ w1730]
            tunnel: w1567 -> [_ w1729]
            tunnel: [w1684 w1728] -> w1566
            tunnel: [w1684 w1727] -> w1565
            tunnel: w1562 -> [_ w1714]
            tunnel: w1561 -> [_ w1713]
            tunnel: w1560 -> [w1676 w1712]
            tunnel: w1559 -> [_ w1711]
            tunnel: [w1684 w1710] -> w1558
            tunnel: [w1684 w1709] -> w1557
            tunnel: [w1677 w1708] -> w1556
            tunnel: [w1684 w1707] -> w1555
            frame "2005-212协议" {
              w1684 = "" ("编码输出")
              # "瞬时流量"
              n558 = Index Array(array=w1676, index #1=5 ("索引"), index #2=1 ("索引")) -> (element #2=w1682:string)  [unwired: 1 out]
              n559 = call "数据编码整合输出.vi"("数据标识"="N", "数据类型"="-Avg=", "污染物编码"="B01", "数据值"=w1682) -> ("编码输出"=w1677:string)  [unwired: 7 in]
            }
            frame "2017-212协议", Default {
              # "盐度改COD"
              # "总铜"
              n560 = Index Array(array=w1729, index #1=2 ("索引"), index #2=3 ("索引"), index #3=5 ("索引")) -> (element #1=w1701:string, element #2=w1700:string, element #3=w1685:string)
              n561 = Index Array(array=w1713, index=1 ("索引")) -> (element=w1689:string)
              n562 = Index Array(array=w1714, index=1 ("索引")) -> (element=w1690:string)
              n563 = Index Array(array=w1712, index=1 ("索引")) -> (element=w1691:string)
              n564 = Index Array(array=w1730, index #1=2 ("索引"), index #2=3 ("索引"), index #3=5 ("索引")) -> (element #1=w1704:string, element #2=w1703:string, element #3=w1687:string)
              n565 = Index Array(array=w1711, index=1 ("索引")) -> (element=w1692:string)
              n566 = case shown="\"M\"" w1704 {
                tunnel: [w1737 ""] -> w1702
                tunnel: w1703 -> [w1737 _]
                frame "N", Default {
                }
                frame "M" {
                }
              }
              n567 = case shown="\"M\"" w1701 {
                tunnel: [w1735 ""] -> w1699
                tunnel: w1700 -> [w1735 _]
                frame "N", Default {
                }
                frame "M" {
                }
              }
              n568 = call "数据编码整合输出.vi"("数据标识"="N" ("字符串"), "数据类型"="-Avg=", "污染物编码"="e01204", "数据值"=w1692) -> ("编码输出"=w1707:string)  [unwired: 7 in]
              n569 = call "数据编码整合输出.vi"("数据标识"="N" ("字符串"), "数据类型"="-Avg=", "污染物编码"="e01203", "数据值"=w1691) -> ("编码输出"=w1708:string)  [unwired: 7 in]
              n570 = call "数据编码整合输出.vi"("数据标识"=w1687, "数据类型"="-Avg=", "污染物编码"="w20122", "数据值"=w1702) -> ("编码输出"=w1728:string)  [unwired: 7 in]
              n571 = call "数据编码整合输出.vi"("数据标识"="N" ("字符串"), "数据类型"="-Avg=", "污染物编码"="e01201", "数据值"=w1690) -> ("编码输出"=w1710:string)  [unwired: 7 in]
              n572 = call "数据编码整合输出.vi"("数据标识"="N" ("字符串"), "数据类型"="-Avg=", "污染物编码"="e01202", "数据值"=w1689) -> ("编码输出"=w1709:string)  [unwired: 7 in]
              n573 = call "数据编码整合输出.vi"("数据标识"=w1685, "数据类型"="-Avg=", "污染物编码"="w01018", "数据值"=w1699) -> ("编码输出"=w1727:string)  [unwired: 7 in]
            }
          }
          n574 = Index Array(array=w1587, index #1=2 ("索引"), index #2=3 ("索引"), index #3=5 ("索引")) -> (element #1=w1423:string, element #2=w1425:string, element #3=w1410:string)
          n575 = Index Array(array=w1592, index #1=2 ("索引"), index #2=3 ("索引"), index #3=5 ("索引")) -> (element #1=w1430:string, element #2=w1431:string, element #3=w1414:string)
          n576 = Index Array(array=w1588, index #1=2 ("索引"), index #2=3 ("索引"), index #3=5 ("索引")) -> (element #1=w1428:string, element #2=w1427:string, element #3=w1412:string)
          n577 = Index Array(array=w1586, index #1=2 ("索引"), index #2=3 ("索引"), index #3=5 ("索引")) -> (element #1=w1422:string, element #2=w1421:string, element #3=w1408:string)
          n578 = Index Array(array=w1480, index #1=2 ("索引"), index #2=3 ("索引"), index #3=5 ("索引")) -> (element #1=w1491:string, element #2=w1489:string, element #3=w1493:string)
          n579 = Index Array(array=w1591, index #1=2 ("索引"), index #2=3 ("索引"), index #3=5 ("索引")) -> (element #1=w1457:string, element #2=w1458:string, element #3=w1453:string)
          n580 = Index Array(array=w1345, index #1=2 ("索引"), index #2=3 ("索引"), index #3=5 ("索引")) -> (element #1=w1372:string, element #2=w1370:string, element #3=w1374:string)
          n581 = Index Array(array=w1378, index #1=2 ("索引"), index #2=3 ("索引"), index #3=5 ("索引")) -> (element #1=w1383:string, element #2=w1385:string, element #3=w1381:string)
          n582 = Index Array(array=w1346, index #1=2 ("索引"), index #2=3 ("索引"), index #3=5 ("索引")) -> (element #1=w1359:string, element #2=w1361:string, element #3=w1357:string)
          n583 = Index Array(array=w1604, index #1=2 ("索引"), index #2=3 ("索引"), index #3=5 ("索引")) -> (element #1=w1434:string, element #2=w1433:string, element #3=w1416:string)
          n584 = Index Array(array=w1379, index #1=2 ("索引"), index #2=3 ("索引"), index #3=5 ("索引")) -> (element #1=w1396:string, element #2=w1394:string, element #3=w1398:string)
          n585 = Index Array(array=w1347, index #1=2 ("索引"), index #2=3 ("索引"), index #3=5 ("索引")) -> (element #1=w1354:string, element #2=w1352:string, element #3=w1356:string)
          n586 = Index Array(array=w1478, index #1=2 ("索引"), index #2=3 ("索引"), index #3=5 ("索引")) -> (element #1=w1503:string, element #2=w1501:string, element #3=w1505:string)
          n587 = Index Array(array=w1380, index #1=2 ("索引"), index #2=3 ("索引"), index #3=5 ("索引")) -> (element #1=w1401:string, element #2=w1403:string, element #3=w1399:string)
          n588 = Index Array(array=w1590, index #1=2 ("索引"), index #2=3 ("索引"), index #3=5 ("索引")) -> (element #1=w1466:string, element #2=w1465:string, element #3=w1462:string)
          n589 = Index Array(array=w1589, index #1=2 ("索引"), index #2=3 ("索引"), index #3=5 ("索引")) -> (element #1=w1536:string, element #2=w1535:string, element #3=w1519:string)
          n590 = Index Array(array=w1479, index #1=2 ("索引"), index #2=3 ("索引"), index #3=5 ("索引")) -> (element #1=w1498:string, element #2=w1496:string, element #3=w1507:string)
          n591 = Index Array(array=w1600, index #1=2 ("索引"), index #2=3 ("索引"), index #3=5 ("索引")) -> (element #1=w1546:string, element #2=w1548:string, element #3=w1527:string)
          n592 = Index Array(array=w1595, index #1=2 ("索引"), index #2=3 ("索引"), index #3=5 ("索引")) -> (element #1=w1544:string, element #2=w1545:string, element #3=w1525:string)
          n593 = Index Array(array=w1603, index #1=2 ("索引"), index #2=3 ("索引"), index #3=5 ("索引")) -> (element #1=w1542:string, element #2=w1541:string, element #3=w1523:string)
          n594 = global read "全局 水样时间.vi" "选择发送的参数"() -> (w1509:string)
          n595 = Index Array(array=w1602, index #1=2 ("索引"), index #2=3 ("索引"), index #3=5 ("索引")) -> (element #1=w1539:string, element #2=w1538:string, element #3=w1521:string)
          n596 = case shown="\"M\"" w1434 {
            tunnel: [w1627 ""] -> w1432
            tunnel: w1433 -> [w1627 _]
            frame "N", Default {
            }
            frame "M" {
            }
          }
          n597 = case shown="\"M\"" w1430 {
            tunnel: [w1625 ""] -> w1429
            tunnel: w1431 -> [w1625 _]
            frame "N", Default {
            }
            frame "M" {
            }
          }
          n598 = case shown="\"M\"" w1428 {
            tunnel: [w1623 ""] -> w1426
            tunnel: w1427 -> [w1623 _]
            frame "N", Default {
            }
            frame "M" {
            }
          }
          n599 = case shown="\"M\"" w1423 {
            tunnel: [w1621 ""] -> w1424
            tunnel: w1425 -> [w1621 _]
            frame "N", Default {
            }
            frame "M" {
            }
          }
          n600 = case shown="\"M\"" w1422 {
            tunnel: [w1619 ""] -> w1420
            tunnel: w1421 -> [w1619 _]
            frame "N", Default {
            }
            frame "M" {
            }
          }
          n601 = case shown="\"M\"" w1542 {
            tunnel: [w1743 ""] -> w1540
            tunnel: w1541 -> [w1743 _]
            frame "N", Default {
            }
            frame "M" {
            }
          }
          n602 = case shown="\"M\"" w1544 {
            tunnel: [w1745 ""] -> w1543
            tunnel: w1545 -> [w1745 _]
            frame "N", Default {
            }
            frame "M" {
            }
          }
          n603 = case shown="\"M\"" w1536 {
            tunnel: [w1739 ""] -> w1534
            tunnel: w1535 -> [w1739 _]
            frame "N", Default {
            }
            frame "M" {
            }
          }
          n604 = case shown="\"N\", 默认" w1491 {
            tunnel: [w1637 ""] -> w1492
            tunnel: w1489 -> [w1637 _]
            frame "N", Default {
            }
            frame "M" {
            }
          }
          n605 = case shown="\"M\"" w1539 {
            tunnel: [w1741 ""] -> w1537
            tunnel: w1538 -> [w1741 _]
            frame "N", Default {
            }
            frame "M" {
            }
          }
          n606 = case shown="\"N\", 默认" w1372 {
            tunnel: [w1607 ""] -> w1373
            tunnel: w1370 -> [w1607 _]
            frame "N", Default {
            }
            frame "M" {
            }
          }
          n607 = case shown="\"N\", 默认" w1383 {
            tunnel: [w1613 ""] -> w1382
            tunnel: w1385 -> [w1613 _]
            frame "N", Default {
            }
            frame "M" {
            }
          }
          n608 = case shown="\"N\", 默认" w1359 {
            tunnel: [w1609 ""] -> w1358
            tunnel: w1361 -> [w1609 _]
            frame "N", Default {
            }
            frame "M" {
            }
          }
          n609 = case shown="\"M\"" w1546 {
            tunnel: [w1747 ""] -> w1547
            tunnel: w1548 -> [w1747 _]
            frame "N", Default {
            }
            frame "M" {
            }
          }
          n610 = case shown="\"N\", 默认" w1396 {
            tunnel: [w1615 ""] -> w1397
            tunnel: w1394 -> [w1615 _]
            frame "N", Default {
            }
            frame "M" {
            }
          }
          n611 = case shown="\"N\", 默认" w1466 {
            tunnel: [w1631 ""] -> w1464
            tunnel: w1465 -> [w1631 _]
            frame "N", Default {
            }
            frame "M" {
            }
          }
          n612 = case shown="\"M\"" w1457 {
            tunnel: [w1629 ""] -> w1456
            tunnel: w1458 -> [w1629 _]
            frame "N", Default {
            }
            frame "M" {
            }
          }
          n613 = case shown="\"N\", 默认" w1354 {
            tunnel: [w1611 ""] -> w1355
            tunnel: w1352 -> [w1611 _]
            frame "N", Default {
            }
            frame "M" {
            }
          }
          n614 = case shown="\"N\", 默认" w1503 {
            tunnel: [w1633 ""] -> w1504
            tunnel: w1501 -> [w1633 _]
            frame "N", Default {
            }
            frame "M" {
            }
          }
          n615 = case shown="\"N\", 默认" w1401 {
            tunnel: [w1617 ""] -> w1400
            tunnel: w1403 -> [w1617 _]
            frame "N", Default {
            }
            frame "M" {
            }
          }
          n616 = case shown="\"N\", 默认" w1498 {
            tunnel: [w1635 ""] -> w1506
            tunnel: w1496 -> [w1635 _]
            frame "N", Default {
            }
            frame "M" {
            }
          }
          n617 = case shown="\"氨氮\"" w1509 {
            tunnel: [w1639 w1640 w1641 w1642 w1643 w1644 w1645 w1646 w1647 w1648 w1649 w1650 w1651 w1652 w1653 w1654 w1655 w1656 w1657 w1658 w1659 w1660 w1661 w1662 w1663 w1664 w1665] -> w1508
            frame "CODMn", Default {
              n618 = global read "全局 所有参数.vi" "CODMn"() -> (w1639:string[][])
            }
            frame "CODCr" {
              n619 = global read "全局 所有参数.vi" "CODCr"() -> (w1640:string[][])
            }
            frame "DO" {
              n620 = global read "全局 所有参数.vi" "DO"() -> (w1641:string[][])
            }
            frame "铜" {
              n621 = global read "全局 所有参数.vi" "铜"() -> (w1642:string[][])
            }
            frame "PH" {
              n622 = global read "全局 所有参数.vi" "PH"() -> (w1643:string[][])
            }
            frame "氨氮" {
              n623 = global read "全局 所有参数.vi" "氨氮"() -> (w1644:string[][])
            }
            frame "比电导率", "电导率" {
              n624 = global read "全局 所有参数.vi" "电导率"() -> (w1645:string[][])
            }
            frame "水温" {
              n625 = global read "全局 所有参数.vi" "水温"() -> (w1646:string[][])
            }
            frame "COD" {
              n626 = global read "全局 所有参数.vi" "盐度"() -> (w1647:string[][])
            }
            frame "浊度" {
              n627 = global read "全局 所有参数.vi" "浊度"() -> (w1648:string[][])
            }
            frame "总氮" {
              n628 = global read "全局 所有参数.vi" "总氮"() -> (w1649:string[][])
            }
            frame "总磷" {
              n629 = global read "全局 所有参数.vi" "总磷"() -> (w1650:string[][])
            }
            frame "叶绿素a" {
              n630 = global read "全局 所有参数.vi" "叶绿素"() -> (w1651:string[][])
            }
            frame "藻密度" {
              n631 = global read "全局 所有参数.vi" "藻密度"() -> (w1652:string[][])
            }
            frame "水位" {
              n632 = global read "全局流量数据小时.vi" "水位"() -> (w1653:string[][])
            }
            frame "流速" {
              n633 = global read "全局流量数据小时.vi" "流速"() -> (w1654:string[][])
            }
            frame "瞬时流量" {
              n634 = global read "全局流量数据小时.vi" "瞬时流量"() -> (w1655:string[][])
            }
            frame "累积流量" {
              n635 = global read "全局流量数据小时.vi" "累积流量"() -> (w1656:string[][])
            }
            frame "亚硝氮" {
              n636 = global read "全局 所有参数.vi" "亚硝酸盐"() -> (w1657:string[][])
            }
            frame "硫化物" {
              n637 = global read "全局 所有参数.vi" "硫化物"() -> (w1658:string[][])
            }
            frame "ORP" {
              n638 = global read "全局 所有参数.vi" "ORP"() -> (w1659:string[][])
            }
            frame "铅" {
              n639 = global read "全局 所有参数.vi" "铅"() -> (w1660:string[][])
            }
            frame "镉" {
              n640 = global read "全局 所有参数.vi" "镉"() -> (w1661:string[][])
            }
            frame "锌" {
              n641 = global read "全局 所有参数.vi" "锌"() -> (w1662:string[][])
            }
            frame "镍" {
              n642 = global read "全局 所有参数.vi" "镍"() -> (w1663:string[][])
            }
            frame "锰" {
              n643 = global read "全局 所有参数.vi" "锰"() -> (w1664:string[][])
            }
            frame "汞" {
              n644 = global read "全局 所有参数.vi" "汞"() -> (w1665:string[][])
            }
          }
          n645 = global read "全局 小时数据发送次数.vi" "小时数据发送次数"() -> (w1553:i32)
          n646 = Index Array(array=w1508, index (row)=w1553) -> (element=w1552:string[])  [unwired: 1 in]
          n647 = global read "断电保存全局.vi" "数据发送协议"() -> (w1512:enum16{"2005-212协议", "2017-212协议"})
          n648 = global read "断电保存全局.vi" "数据发送协议"() -> (w1511:enum16{"2005-212协议", "2017-212协议"})
          n649 = global read "断电保存全局.vi" "数据发送协议"() -> (w1510:enum16{"2005-212协议", "2017-212协议"})
          n650 = Index Array(array=w1552, index=0 ("索引")) -> (element=w1550:string)
          n651 = case shown="\"2017-212协议\", 默认" w1510 {
            tunnel: ["011" ("污染物编码") "w01018" ("污染物编码")] -> w1514
            frame "2005-212协议" {
            }
            frame "2017-212协议", Default {
            }
          }
          n652 = case shown="\"2017-212协议\", 默认" w1512 {
            tunnel: ["101" ("污染物编码") "w21011" ("污染物编码")] -> w1518
            tunnel: ["065" ("污染物编码") "w21001" ("污染物编码")] -> w1517
            tunnel: ["001" ("污染物编码") "w01001" ("污染物编码")] -> w1516
            frame "2005-212协议" {
            }
            frame "2017-212协议", Default {
            }
          }
          n653 = case shown="\"2005-212协议\"" w1511 {
            tunnel: ["060" ("污染物编码") "w21003" ("污染物编码")] -> w1515
            frame "2005-212协议" {
            }
            frame "2017-212协议", Default {
            }
          }
          n654 = call "数据编码整合输出.vi"("数据标识"=w1374, "数据类型"="-Avg=", "污染物编码"="w20111", "数据值"=w1373) -> ("编码输出"=w1342:string)  [unwired: 7 in]
          n655 = call "数据编码整合输出.vi"("数据标识"=w1381, "数据类型"="-Avg=", "污染物编码"="w20123", "数据值"=w1382) -> ("编码输出"=w1377:string)  [unwired: 7 in]
          n656 = call "数据编码整合输出.vi"("数据标识"=w1357, "数据类型"="-Avg=", "污染物编码"="w20124", "数据值"=w1358) -> ("编码输出"=w1343:string)  [unwired: 7 in]
          n657 = call "数据编码整合输出.vi"("数据标识"=w1398, "数据类型"="-Avg=", "污染物编码"="w20115", "数据值"=w1397) -> ("编码输出"=w1376:string)  [unwired: 7 in]
          n658 = call "数据编码整合输出.vi"("数据标识"=w1356, "数据类型"="-Avg=", "污染物编码"="w20121", "数据值"=w1355) -> ("编码输出"=w1344:string)  [unwired: 7 in]
          n659 = call "数据编码整合输出.vi"("数据标识"=w1505, "数据类型"="-Avg=", "污染物编码"="w01100", "数据值"=w1504) -> ("编码输出"=w1477:string)  [unwired: 7 in]
          n660 = call "数据编码整合输出.vi"("数据标识"=w1399, "数据类型"="-Avg=", "污染物编码"="w20120", "数据值"=w1400) -> ("编码输出"=w1375:string)  [unwired: 7 in]
          n661 = call "数据编码整合输出.vi"("数据标识"=w1493, "数据类型"="-Avg=", "污染物编码"="w21006", "数据值"=w1492) -> ("编码输出"=w1475:string)  [unwired: 7 in]
          n662 = call "数据编码整合输出.vi"("数据标识"=w1507, "数据类型"="-Avg=", "污染物编码"="w21019", "数据值"=w1506) -> ("编码输出"=w1476:string)  [unwired: 7 in]
          n663 = call "规范小时时间戳.vi"("字符串"=w1550) -> ("result string"=w1530:string)  [unwired: 10 in]
          n664 = call "数据编码整合输出.vi"("数据标识"=w1462, "数据类型"="-Avg=", "污染物编码"="w01019", "数据值"=w1464) -> ("编码输出"=w1585:string)  [unwired: 7 in]
          n665 = call "数据编码整合输出.vi"("数据标识"=w1453, "数据类型"="-Avg=", "污染物编码"="w01010", "数据值"=w1456) -> ("编码输出"=w1582:string)  [unwired: 7 in]
          n666 = call "数据编码整合输出.vi"("数据标识"=w1525, "数据类型"="-Avg=", "污染物编码"=w1514, "数据值"=w1543) -> ("编码输出"=w1580:string)  [unwired: 7 in]
          n667 = call "数据编码整合输出.vi"("数据标识"=w1527, "数据类型"="-Avg=", "污染物编码"=w1515, "数据值"=w1547) -> ("编码输出"=w1583:string)  [unwired: 7 in]
          n668 = call "数据编码整合输出.vi"("数据标识"=w1521, "数据类型"="-Avg=", "污染物编码"=w1517, "数据值"=w1537) -> ("编码输出"=w1571:string)  [unwired: 7 in]
          n669 = call "数据编码整合输出.vi"("数据标识"=w1519, "数据类型"="-Avg=", "污染物编码"=w1516, "数据值"=w1534) -> ("编码输出"=w1569:string)  [unwired: 7 in]
          n670 = call "数据编码整合输出.vi"("数据标识"=w1414, "数据类型"="-Avg=", "污染物编码"="w01014", "数据值"=w1429) -> ("编码输出"=w1578:string)  [unwired: 7 in]
          n671 = call "数据编码整合输出.vi"("数据标识"=w1416, "数据类型"="-Avg=", "污染物编码"="w01009", "数据值"=w1432) -> ("编码输出"=w1579:string)  [unwired: 7 in]
          n672 = call "数据编码整合输出.vi"("数据标识"=w1408, "数据类型"="-Avg=", "污染物编码"="w19011", "数据值"=w1420) -> ("编码输出"=w1575:string)  [unwired: 7 in]
          n673 = call "数据编码整合输出.vi"("数据标识"=w1412, "数据类型"="-Avg=", "污染物编码"="w01003", "数据值"=w1426) -> ("编码输出"=w1577:string)  [unwired: 7 in]
          n674 = call "数据编码整合输出.vi"("数据标识"=w1410, "数据类型"="-Avg=", "污染物编码"="w01016", "数据值"=w1424) -> ("编码输出"=w1576:string)  [unwired: 7 in]
          n675 = call "数据编码整合输出.vi"("数据标识"=w1523, "数据类型"="-Avg=", "污染物编码"=w1518, "数据值"=w1540) -> ("编码输出"=w1573:string)  [unwired: 7 in]
          n676 = Format Into String(format string="DataTime=%s;", w1530) -> (resulting string=w1533:string)  [unwired: 2 in, 1 out]
          n677 = Format Into String(format string="%s%s%s%s%s%s%s%s%s%s%s%s%s%s%s%s%s%s%s%s%s%s%s%s%s%s%s" ("格式字符串"), w1585, w1583, w1582, w1580, w1579, w1578, w1577, w1576, w1575, w1573, w1571, w1569, w1566, w1565, w1558, w1557, w1556, w1555, w1475, w1476, w1477, w1375, w1376, w1377, w1344, w1343, w1342) -> (resulting string=w1531:string)  [unwired: 2 in, 1 out]
          n678 = Empty String/Path?(string/path=w1531) -> (empty?=w1564:bool)
          n679 = Concatenate Strings(w1533, w1531) -> (w1472:string)
          n680 = String Length(string=w1472) -> (length=w1474:i32)
          n681 = Decrement(x=w1474) -> (x-1=w1473:i32)
          n682 = String Subset(string=w1472, length (rest)=w1473) -> (substring=w1471:string)  [unwired: 1 in]
          n683 = global read "全局 数据发送重叠.vi" "主动上报数据中"() -> (w1549:bool)
          n684 = case shown="假" w1564 {
            tunnel: [w1750 ""] -> w1563
            tunnel: w1471 -> [w1750 _]
            tunnel: w1549 -> [w1749 w1753]
            frame False {
              n685 = case shown="真" w1749 {
                frame False {
                  n686 = global read "全局 小时数据发送次数.vi" "小时数据发送次数"() -> (w1752:i32)
                  n687 = Increment(x=w1752) -> (x+1=w1751:i32)
                  n688 = global write "全局 小时数据发送次数.vi" "小时数据发送次数"(w1751) -> ()
                }
                frame True {
                }
              }
            }
            frame True {
              n689 = case shown="假" w1753 {
                frame False {
                  n690 = global read "全局 小时数据发送次数.vi" "小时数据发送次数"() -> (w1756:i32)
                  n691 = Increment(x=w1756) -> (x+1=w1755:i32)
                  n692 = global write "全局 小时数据发送次数.vi" "小时数据发送次数"(w1755) -> ()
                }
                frame True {
                }
              }
            }
          }
        }
        frame "返回执行结果" {
          (unwired) 0 ("当前包数")
          n693 = global write "全局1.vi" "枚举"(enum16{"返回请求应答", "上传数据", "返回执行结果"}."返回请求应答" ("枚举")) -> ()
        }
      }
    }
    frame "剖面多参数H" {
      # "发送小时数据"
      n694 = global read "全局1.vi" "枚举"() -> (w1759:enum16{"返回请求应答", "上传数据", "返回执行结果"})
      n695 = case shown="\"上传数据\"" w1759 {
        tunnel: ["QnRtn=1" w1769 "ExeRtn=1"] -> w1760
        frame "返回请求应答", Default {
          (unwired) 0 ("当前包数")
          n696 = global read "全局 数据数组大小.vi" "数据数组大小"() -> (w1761:i32)
          n697 = global write "全局1.vi" "枚举"(enum16{"返回请求应答", "上传数据", "返回执行结果"}."上传数据" ("枚举")) -> ()
          n698 = Equal To 0?(x=w1761) -> (x = 0?=w1762:bool)
          n699 = case shown="真" w1762 {
            frame False {
            }
            frame True {
              n700 = global read "全局 小时数据发送次数.vi" "小时数据发送次数"() -> (w1766:i32)
              n701 = Increment(x=w1766) -> (x+1=w1765:i32)
              n702 = global write "全局 小时数据发送次数.vi" "小时数据发送次数"(w1765) -> ()
            }
          }
        }
        frame "上传数据" {
          n703 = global read "断电保存全局.vi" "数据发送协议"() -> (w1768:enum16{"2005-212协议", "2017-212协议"})
          n704 = case shown="\"2017-212协议\", 默认" w1768 {
            tunnel: ["" ("编码输出") w1774] -> w1767
            frame "2005-212协议" {
            }
            frame "2017-212协议", Default {
              (unwired) "w01010" ("污染物编码")
              (unwired) "w01016" ("污染物编码")
              (unwired) "w01003" ("污染物编码")
              (unwired) "w01009" ("污染物编码")
              (unwired) "w01001" ("污染物编码")
              (unwired) "w01014" ("污染物编码")
              (unwired) "w01100" ("污染物编码")
              # "时间,测量模式,数据类型,数据标识,层数,Temp,SpCond,Cond,Sal,TDS,pH,pHmV,ORP,ODO%,ODOmg/L,Turb,Chla,Depth,"
              n705 = global read "全局 小时数据发送次数.vi" "小时数据发送次数"() -> (w1792:i32)
              n706 = global read "全局 所有参数.vi" "剖面多参数"() -> (w1795:string[][])
              n707 = Index Array(array=w1795, index (row)=w1792) -> (element=w1793:string[])  [unwired: 1 in]
              n708 = Index Array(array=w1793, index #1=0 ("索引")) -> (element #1=w1777:string, element #3=w1791:string, element #4=w1790:string, element #5=w1789:string, element #6=w1788:string, element #7=w1787:string, element #11=w1785:string, element #13=w1784:string, element #15=w1783:string, element #16=w1782:string, element #17=w1781:string)  [unwired: 16 in, 6 out]
              n709 = Build Array(w1788, w1787, w1785, w1784, w1783, w1782, w1781) -> (w1786:string[])
              n710 = call "剖面多参数组合(子VI).vi"("数据类型实时小时"="-Avg=", "数据值"=w1786, "层数"=w1789, "数据标识"=w1790, "数据类型"=w1791) -> ("编码输出"=w1773:string)  [unwired: 6 in]
              n711 = call "规范小时时间戳.vi"("字符串"=w1777) -> ("result string"=w1778:string)  [unwired: 10 in]
              n712 = Format Into String(format string="DataTime=%s;", w1778) -> (resulting string=w1779:string)  [unwired: 2 in, 1 out]
              n713 = Concatenate Strings(w1779, w1773) -> (w1775:string)
              n714 = Empty String/Path?(string/path=w1773) -> (empty?=w1776:bool)
              n715 = case shown="真" w1776 {
                tunnel: [w1796 ""] -> w1774
                tunnel: w1775 -> [w1796 _]
                frame False {
                }
                frame True {
                }
              }
            }
          }
          n716 = Empty String/Path?(string/path=w1767) -> (empty?=w1770:bool)
          n717 = case shown="假" w1770 {
            tunnel: [w1800 ""] -> w1769
            tunnel: w1767 -> [w1800 _]
            frame False {
              n718 = global read "全局 小时数据发送次数.vi" "小时数据发送次数"() -> (w1799:i32)
              n719 = Increment(x=w1799) -> (x+1=w1798:i32)
              n720 = global write "全局 小时数据发送次数.vi" "小时数据发送次数"(w1798) -> ()
            }
            frame True {
              n721 = global read "全局 小时数据发送次数.vi" "小时数据发送次数"() -> (w1802:i32)
              n722 = Increment(x=w1802) -> (x+1=w1801:i32)
              n723 = global write "全局 小时数据发送次数.vi" "小时数据发送次数"(w1801) -> ()
            }
          }
        }
        frame "返回执行结果" {
          (unwired) 0 ("当前包数")
          n724 = global write "全局1.vi" "枚举"(enum16{"返回请求应答", "上传数据", "返回执行结果"}."返回请求应答" ("枚举")) -> ()
        }
      }
    }
    frame "剖面多参数S" {
      # "发送实时数据"
      n725 = global read "全局1.vi" "枚举"() -> (w1806:enum16{"返回请求应答", "上传数据", "返回执行结果"})
      n726 = case shown="\"上传数据\"" w1806 {
        tunnel: ["QnRtn=1" w1816 "ExeRtn=1"] -> w1807
        frame "返回请求应答", Default {
          (unwired) 0 ("当前包数")
          n727 = global read "全局 数据数组大小.vi" "数据数组大小"() -> (w1808:i32)
          n728 = global write "全局1.vi" "枚举"(enum16{"返回请求应答", "上传数据", "返回执行结果"}."上传数据" ("枚举")) -> ()
          n729 = Equal To 0?(x=w1808) -> (x = 0?=w1809:bool)
          n730 = case shown="真" w1809 {
            frame False {
            }
            frame True {
              n731 = global read "全局 小时数据发送次数.vi" "小时数据发送次数"() -> (w1813:i32)
              n732 = Increment(x=w1813) -> (x+1=w1812:i32)
              n733 = global write "全局 小时数据发送次数.vi" "小时数据发送次数"(w1812) -> ()
            }
          }
        }
        frame "上传数据" {
          n734 = global read "断电保存全局.vi" "数据发送协议"() -> (w1815:enum16{"2005-212协议", "2017-212协议"})
          n735 = case shown="\"2017-212协议\", 默认" w1815 {
            tunnel: ["" ("编码输出") w1823] -> w1814
            frame "2005-212协议" {
            }
            frame "2017-212协议", Default {
              (unwired) "w01010" ("污染物编码")
              (unwired) "w01016" ("污染物编码")
              (unwired) "w01003" ("污染物编码")
              (unwired) "w01009" ("污染物编码")
              (unwired) "w01001" ("污染物编码")
              (unwired) "w01014" ("污染物编码")
              (unwired) "w01100" ("污染物编码")
              # "时间,测量模式,数据类型,数据标识,层数,Temp,SpCond,Cond,Sal,TDS,pH,pHmV,ORP,ODO%,ODOmg/L,Turb,Chla,Depth,"
              n736 = global read "全局 小时数据发送次数.vi" "小时数据发送次数"() -> (w1839:i32)
              n737 = global read "全局 所有参数.vi" "剖面多参数"() -> (w1842:string[][])
              n738 = Index Array(array=w1842, index (row)=w1839) -> (element=w1840:string[])  [unwired: 1 in]
              n739 = Index Array(array=w1840, index #1=0 ("索引")) -> (element #1=w1820:string, element #3=w1838:string, element #4=w1837:string, element #5=w1836:string, element #6=w1835:string, element #7=w1834:string, element #11=w1832:string, element #13=w1831:string, element #15=w1830:string, element #16=w1829:string, element #17=w1828:string)  [unwired: 16 in, 6 out]
              n740 = Build Array(w1835, w1834, w1832, w1831, w1830, w1829, w1828) -> (w1833:string[])
              n741 = call "剖面多参数组合(子VI).vi"("数据类型实时小时"="-Rtd=", "数据值"=w1833, "层数"=w1836, "数据标识"=w1837, "数据类型"=w1838) -> ("编码输出"=w1822:string)  [unwired: 6 in]
              n742 = call "规范时间戳.vi"("字符串"=w1820) -> ("result string"=w1819:string)  [unwired: 10 in]
              n743 = Format Into String(format string="DataTime=%s;", w1819) -> (resulting string=w1826:string)  [unwired: 2 in, 1 out]
              n744 = Concatenate Strings(w1826, w1822) -> (w1824:string)
              n745 = Empty String/Path?(string/path=w1822) -> (empty?=w1825:bool)
              n746 = case shown="假" w1825 {
                tunnel: [w1843 ""] -> w1823
                tunnel: w1824 -> [w1843 _]
                frame False {
                }
                frame True {
                }
              }
            }
          }
          n747 = Empty String/Path?(string/path=w1814) -> (empty?=w1817:bool)
          n748 = case shown="假" w1817 {
            tunnel: [w1847 ""] -> w1816
            tunnel: w1814 -> [w1847 _]
            frame False {
              n749 = global read "全局 小时数据发送次数.vi" "小时数据发送次数"() -> (w1846:i32)
              n750 = Increment(x=w1846) -> (x+1=w1845:i32)
              n751 = global write "全局 小时数据发送次数.vi" "小时数据发送次数"(w1845) -> ()
            }
            frame True {
              n752 = global read "全局 小时数据发送次数.vi" "小时数据发送次数"() -> (w1849:i32)
              n753 = Increment(x=w1849) -> (x+1=w1848:i32)
              n754 = global write "全局 小时数据发送次数.vi" "小时数据发送次数"(w1848) -> ()
            }
          }
        }
        frame "返回执行结果" {
          (unwired) 0 ("当前包数")
          n755 = global write "全局1.vi" "枚举"(enum16{"返回请求应答", "上传数据", "返回执行结果"}."返回请求应答" ("枚举")) -> ()
        }
      }
    }
    frame "提取小时数据" {
      # "藻密度"
      # "叶绿素"
      # "浊度"
      # "水温"
      # "发送小时数据"
      n756 = global read "全局 小时数据发送次数.vi" "小时数据发送次数"() -> (w1877:i32)
      n757 = global read "全局 小时数据发送次数.vi" "小时数据发送次数"() -> (w1860:i32)
      n758 = global read "全局 小时数据发送次数.vi" "小时数据发送次数"() -> (w1859:i32)
      n759 = global read "全局 小时数据发送次数.vi" "小时数据发送次数"() -> (w1878:i32)
      n760 = global read "全局 小时数据发送次数.vi" "小时数据发送次数"() -> (w1865:i32)
      n761 = global read "全局 小时数据发送次数.vi" "小时数据发送次数"() -> (w1881:i32)
      n762 = global read "全局 小时数据发送次数.vi" "小时数据发送次数"() -> (w1867:i32)
      n763 = global read "全局 小时数据发送次数.vi" "小时数据发送次数"() -> (w1887:i32)
      n764 = global read "全局 小时数据发送次数.vi" "小时数据发送次数"() -> (w1873:i32)
      n765 = global read "全局 小时数据发送次数.vi" "小时数据发送次数"() -> (w1885:i32)
      n766 = global read "全局 小时数据发送次数.vi" "小时数据发送次数"() -> (w1870:i32)
      n767 = global read "全局 小时数据发送次数.vi" "小时数据发送次数"() -> (w1861:i32)
      n768 = global read "全局 小时数据发送次数.vi" "小时数据发送次数"() -> (w1889:i32)
      n769 = global read "全局 小时数据发送次数.vi" "小时数据发送次数"() -> (w1875:i32)
      n770 = global read "全局 小时数据发送次数.vi" "小时数据发送次数"() -> (w1883:i32)
      n771 = global read "全局 小时数据发送次数.vi" "小时数据发送次数"() -> (w1871:i32)
      n772 = global read "全局 小时数据发送次数.vi" "小时数据发送次数"() -> (w1891:i32)
      n773 = Index Array(array=w1856, index (row)=w1860) -> (element=w1855:string[])  [unwired: 1 in]
      n774 = Index Array(array=w1854, index (row)=w1859) -> (element=w1853:string[])  [unwired: 1 in]
      n775 = Index Array(array=w1898, index (row)=w1878) -> (element=w1879:string[])  [unwired: 1 in]
      n776 = Index Array(array=w1862, index (row)=w1865) -> (element=w1864:string[])  [unwired: 1 in]
      n777 = Index Array(array=w1899, index (row)=w1881) -> (element=w1880:string[])  [unwired: 1 in]
      n778 = Index Array(array=w1863, index (row)=w1867) -> (element=w1866:string[])  [unwired: 1 in]
      n779 = Index Array(array=w1903, index (row)=w1889) -> (element=w1888:string[])  [unwired: 1 in]
      n780 = Index Array(array=w1902, index (row)=w1887) -> (element=w1886:string[])  [unwired: 1 in]
      n781 = Index Array(array=w1901, index (row)=w1885) -> (element=w1884:string[])  [unwired: 1 in]
      n782 = Index Array(array=w1904, index (row)=w1891) -> (element=w1890:string[])  [unwired: 1 in]
      n783 = Index Array(array=w1897, index (row)=w1877) -> (element=w1876:string[])  [unwired: 1 in]
      n784 = Index Array(array=w1858, index (row)=w1861) -> (element=w1857:string[])  [unwired: 1 in]
      n785 = Index Array(array=w1895, index (row)=w1873) -> (element=w1872:string[])  [unwired: 1 in]
      n786 = Index Array(array=w1896, index (row)=w1875) -> (element=w1874:string[])  [unwired: 1 in]
      n787 = Index Array(array=w1900, index (row)=w1883) -> (element=w1882:string[])  [unwired: 1 in]
      n788 = Index Array(array=w1893, index (row)=w1870) -> (element=w1868:string[])  [unwired: 1 in]
      n789 = Index Array(array=w1894, index (row)=w1871) -> (element=w1869:string[])  [unwired: 1 in]
      n790 = global read "全局1.vi" "枚举"() -> (w1892:enum16{"返回请求应答", "上传数据", "返回执行结果"})
      n791 = case shown="\"上传数据\"" w1892 {
        tunnel: ["QnRtn=1" w1982 "ExeRtn=1"] -> w1905
        tunnel: w1890 -> [_ w2036 _]
        tunnel: w1886 -> [_ w2049 _]
        tunnel: w1884 -> [_ w2048 _]
        tunnel: w1882 -> [_ w2047 _]
        tunnel: w1888 -> [_ w2046 _]
        tunnel: w1880 -> [_ w2035 _]
        tunnel: w1879 -> [_ w2040 _]
        tunnel: w1876 -> [_ w2038 _]
        tunnel: w1874 -> [_ w2037 _]
        tunnel: w1872 -> [_ w2034 _]
        tunnel: w1869 -> [_ w2033 _]
        tunnel: w1868 -> [_ w2032 _]
        tunnel: w1866 -> [_ w1987 _]
        tunnel: w1864 -> [_ w1986 _]
        tunnel: w1857 -> [_ w1919 _]
        tunnel: w1855 -> [_ w1917 _]
        tunnel: w1853 -> [_ w1915 _]
        frame "返回请求应答", Default {
          n792 = global read "全局 数据数组大小.vi" "数据数组大小"() -> (w1906:i32)
          n793 = Equal To 0?(x=w1906) -> (x = 0?=w1907:bool)
          n794 = case shown="真" w1907 {
            frame False {
            }
            frame True {
              n795 = global read "全局 小时数据发送次数.vi" "小时数据发送次数"() -> (w1910:i32)
              n796 = Increment(x=w1910) -> (x+1=w1909:i32)
              n797 = global write "全局 小时数据发送次数.vi" "小时数据发送次数"(w1909) -> ()
            }
          }
        }
        frame "上传数据" {
          (unwired) 2 ("数据精度")
          (unwired) 3 ("数据精度")
          (unwired) 3 ("数据精度")
          (unwired) 3 ("数据精度")
          (unwired) 3 ("数据精度")
          # "瞬时流量"
          # "流速"
          # "水位"
          # "盐度"
          # "总铜"
          # "PH"
          # "总氮"
          # "总磷"
          # "藻密度"
          # "叶绿素"
          # "浊度"
          # "电导率"
          # "DO"
          # "CODCr"
          # "水温"
          # "NH3"
          # "CODMn"
          n798 = Index Array(array=w2033, index #2=1 ("索引")) -> (element #2=w1968:string)  [unwired: 1 in, 1 out]
          n799 = Index Array(array=w2038, index #2=1 ("索引")) -> (element #2=w1970:string)  [unwired: 1 in, 1 out]
          n800 = Index Array(array=w2034, index #2=1 ("索引")) -> (element #2=w1969:string)  [unwired: 1 in, 1 out]
          n801 = Index Array(array=w1917, index #2=1 ("索引")) -> (element #2=w1916:string)  [unwired: 1 in, 1 out]
          n802 = Index Array(array=w1915, index #2=1 ("索引")) -> (element #2=w1914:string)  [unwired: 1 in, 1 out]
          n803 = Index Array(array=w2032, index #2=1 ("索引")) -> (element #2=w1967:string)  [unwired: 1 in, 1 out]
          n804 = Index Array(array=w2037, index #2=1 ("索引")) -> (element #2=w1973:string)  [unwired: 1 in, 1 out]
          n805 = Index Array(array=w2049, index #2=1 ("索引")) -> (element #2=w1971:string)  [unwired: 1 in, 1 out]
          n806 = Index Array(array=w2036, index #2=1 ("索引")) -> (element #1=w1956:string, element #2=w1975:string)  [unwired: 1 in]
          n807 = Index Array(array=w2035, index #2=1 ("索引")) -> (element #2=w1964:string)  [unwired: 1 in, 1 out]
          n808 = Index Array(array=w1986, index #2=1 ("索引")) -> (element #2=w1962:string)  [unwired: 1 in, 1 out]
          n809 = Index Array(array=w1919, index #2=1 ("索引")) -> (element #2=w1918:string)  [unwired: 1 in, 1 out]
          n810 = Index Array(array=w1987, index #2=1 ("索引")) -> (element #2=w1963:string)  [unwired: 1 in, 1 out]
          n811 = Index Array(array=w2046, index #2=1 ("索引")) -> (element #2=w1974:string)  [unwired: 1 in, 1 out]
          n812 = Index Array(array=w2040, index #2=1 ("索引")) -> (element #2=w1972:string)  [unwired: 1 in, 1 out]
          n813 = Index Array(array=w2048, index #2=1 ("索引")) -> (element #2=w1966:string)  [unwired: 1 in, 1 out]
          n814 = Index Array(array=w2047, index #2=1 ("索引")) -> (element #2=w1965:string)  [unwired: 1 in, 1 out]
          n815 = global read "断电保存全局.vi" "数据发送协议"() -> (w1944:enum16{"2005-212协议", "2017-212协议"})
          n816 = global read "断电保存全局.vi" "数据发送协议"() -> (w1938:enum16{"2005-212协议", "2017-212协议"})
          n817 = global read "断电保存全局.vi" "数据发送协议"() -> (w1939:enum16{"2005-212协议", "2017-212协议"})
          n818 = global read "断电保存全局.vi" "数据发送协议"() -> (w1929:enum16{"2005-212协议", "2017-212协议"})
          n819 = global read "断电保存全局.vi" "数据发送协议"() -> (w1950:enum16{"2005-212协议", "2017-212协议"})
          n820 = global read "断电保存全局.vi" "数据发送协议"() -> (w1926:enum16{"2005-212协议", "2017-212协议"})
          n821 = global read "断电保存全局.vi" "数据发送协议"() -> (w1940:enum16{"2005-212协议", "2017-212协议"})
          n822 = global read "断电保存全局.vi" "数据发送协议"() -> (w1921:enum16{"2005-212协议", "2017-212协议"})
          n823 = global read "断电保存全局.vi" "数据发送协议"() -> (w1952:enum16{"2005-212协议", "2017-212协议"})
          n824 = global read "断电保存全局.vi" "数据发送协议"() -> (w1942:enum16{"2005-212协议", "2017-212协议"})
          n825 = global read "断电保存全局.vi" "数据发送协议"() -> (w1948:enum16{"2005-212协议", "2017-212协议"})
          n826 = case shown="\"2005-212协议\"" w1938 {
            tunnel: ["465" ("污染物编码") "w01003" ("污染物编码")] -> w1935
            frame "2005-212协议" {
            }
            frame "2017-212协议", Default {
            }
          }
          n827 = case shown="\"2005-212协议\"" w1944 {
            tunnel: ["314" ("污染物编码") "w01019" ("污染物编码")] -> w1943
            frame "2005-212协议" {
            }
            frame "2017-212协议", Default {
            }
          }
          n828 = case shown="\"2005-212协议\"" w1939 {
            tunnel: ["463" ("污染物编码") "w01014" ("污染物编码")] -> w1936
            frame "2005-212协议" {
            }
            frame "2017-212协议", Default {
            }
          }
          n829 = case shown="\"2005-212协议\"" w1929 {
            tunnel: ["490" ("污染物编码") "w01003" ("污染物编码")] -> w1928
            frame "2005-212协议" {
            }
            frame "2017-212协议", Default {
            }
          }
          n830 = case shown="\"2005-212协议\"" w1950 {
            tunnel: ["316" ("污染物编码") "w01018" ("污染物编码")] -> w1949
            frame "2005-212协议" {
            }
            frame "2017-212协议", Default {
            }
          }
          n831 = case shown="\"2005-212协议\"" w1926 {
            tunnel: ["497" ("污染物编码") "w01003" ("污染物编码")] -> w1927
            frame "2005-212协议" {
            }
            frame "2017-212协议", Default {
            }
          }
          n832 = case shown="\"2005-212协议\"" w1940 {
            tunnel: ["315" ("污染物编码") "w01009" ("污染物编码")] -> w1937
            frame "2005-212协议" {
            }
            frame "2017-212协议", Default {
            }
          }
          n833 = case shown="\"2005-212协议\"" w1921 {
            tunnel: ["492" ("污染物编码") "w01003" ("污染物编码")] -> w1920
            frame "2005-212协议" {
            }
            frame "2017-212协议", Default {
            }
          }
          n834 = case shown="\"2005-212协议\"" w1952 {
            tunnel: ["311" ("污染物编码") "w21003" ("污染物编码")] -> w1951
            frame "2005-212协议" {
            }
            frame "2017-212协议", Default {
            }
          }
          n835 = case shown="\"2005-212协议\"" w1942 {
            tunnel: ["301" ("污染物编码") "w01010" ("污染物编码")] -> w1941
            frame "2005-212协议" {
            }
            frame "2017-212协议", Default {
            }
          }
          n836 = case shown="\"2005-212协议\"" w1948 {
            tunnel: ["313" ("污染物编码") "w21011" ("污染物编码")] -> w1947
            tunnel: ["466" ("污染物编码") "w21001" ("污染物编码")] -> w1946
            tunnel: ["302" ("污染物编码") "w01001" ("污染物编码")] -> w1945
            frame "2005-212协议" {
            }
            frame "2017-212协议", Default {
            }
          }
          n837 = call "规范小时时间戳.vi"("字符串"=w1956) -> ("result string"=w1957:string)  [unwired: 10 in]
          n838 = call "数据编码整合输出.vi"("数据标识"="N" ("字符串"), "数据类型"="-Avg=", "污染物编码"=w1943, "数据值"=w1975) -> ("编码输出"=w2031:string)  [unwired: 7 in]
          n839 = call "数据编码整合输出.vi"("数据标识"="N" ("字符串"), "数据类型"="-Avg=", "污染物编码"=w1941, "数据值"=w1973) -> ("编码输出"=w2023:string)  [unwired: 7 in]
          n840 = call "数据编码整合输出.vi"("数据标识"="N" ("字符串"), "数据类型"="-Avg=", "污染物编码"=w1949, "数据值"=w1972) -> ("编码输出"=w2020:string)  [unwired: 7 in]
          n841 = call "数据编码整合输出.vi"("数据标识"="N" ("字符串"), "数据类型"="-Avg=", "污染物编码"=w1951, "数据值"=w1974) -> ("编码输出"=w2026:string)  [unwired: 7 in]
          n842 = call "数据编码整合输出.vi"("数据标识"="N" ("字符串"), "数据类型"="-Avg=", "污染物编码"="w20122", "数据值"=w1963) -> ("编码输出"=w1985:string)  [unwired: 7 in]
          n843 = call "数据编码整合输出.vi"("数据标识"="N" ("字符串"), "数据类型"="-Avg=", "污染物编码"=w1946, "数据值"=w1965) -> ("编码输出"=w1997:string)  [unwired: 7 in]
          n844 = call "数据编码整合输出.vi"("数据标识"="N" ("字符串"), "数据类型"="-Avg=", "污染物编码"=w1945, "数据值"=w1964) -> ("编码输出"=w1994:string)  [unwired: 7 in]
          n845 = call "数据编码整合输出.vi"("数据标识"="N" ("字符串"), "数据类型"="-Avg=", "污染物编码"="w01015", "数据值"=w1962) -> ("编码输出"=w1984:string)  [unwired: 7 in]
          n846 = call "数据编码整合输出.vi"("数据标识"="N" ("字符串"), "数据类型"="-Avg=", "污染物编码"=w1936, "数据值"=w1970) -> ("编码输出"=w2014:string)  [unwired: 7 in]
          n847 = call "数据编码整合输出.vi"("数据标识"="N" ("字符串"), "数据类型"="-Avg=", "污染物编码"=w1937, "数据值"=w1971) -> ("编码输出"=w2017:string)  [unwired: 7 in]
          n848 = call "数据编码整合输出.vi"("数据标识"="N" ("字符串"), "数据类型"="-Avg=", "污染物编码"="w19011", "数据值"=w1967) -> ("编码输出"=w2003:string)  [unwired: 7 in]
          n849 = call "数据编码整合输出.vi"("数据标识"="N" ("字符串"), "数据类型"="-Avg=", "污染物编码"=w1935, "数据值"=w1969) -> ("编码输出"=w2011:string)  [unwired: 7 in]
          n850 = call "数据编码整合输出.vi"("数据标识"="N" ("字符串"), "数据类型"="-Avg=", "污染物编码"="w01016", "数据值"=w1968) -> ("编码输出"=w2007:string)  [unwired: 7 in]
          n851 = call "数据编码整合输出.vi"("数据标识"="N" ("字符串"), "数据类型"="-Avg=", "污染物编码"=w1947, "数据值"=w1966) -> ("编码输出"=w2000:string)  [unwired: 7 in]
          n852 = call "数据编码整合输出.vi"("数据标识"="N" ("字符串"), "数据类型"="-Avg=", "污染物编码"=w1928, "数据值"=w1918) -> ("编码输出"=w1913:string)  [unwired: 7 in]
          n853 = call "数据编码整合输出.vi"("数据标识"="N" ("字符串"), "数据类型"="-Avg=", "污染物编码"=w1927, "数据值"=w1916) -> ("编码输出"=w1912:string)  [unwired: 7 in]
          n854 = call "数据编码整合输出.vi"("数据标识"="N" ("字符串"), "数据类型"="-Avg=", "污染物编码"=w1920, "数据值"=w1914) -> ("编码输出"=w1911:string)  [unwired: 7 in]
          n855 = Format Into String(format string="DataTime=%s;", w1957) -> (resulting string=w1961:string)  [unwired: 2 in, 1 out]
          n856 = Format Into String(format string="%s%s%s%s%s%s%s%s%s%s%s%s%s%s%s%s%s" ("格式字符串"), w2031, w2026, w2023, w2020, w2017, w2014, w2011, w2007, w2003, w2000, w1997, w1994, w1985, w1984, w1913, w1912, w1911) -> (resulting string=w1959:string)  [unwired: 2 in, 1 out]
          n857 = Concatenate Strings(w1961, w1959) -> (w1958:string)
          n858 = Empty String/Path?(string/path=w1959) -> (empty?=w1983:bool)
          n859 = case shown="假" w1983 {
            tunnel: [w2078 ""] -> w1982
            tunnel: w1958 -> [w2078 _]
            frame False {
              n860 = global read "全局 小时数据发送次数.vi" "小时数据发送次数"() -> (w2077:i32)
              n861 = Increment(x=w2077) -> (x+1=w2076:i32)
              n862 = global write "全局 小时数据发送次数.vi" "小时数据发送次数"(w2076) -> ()
            }
            frame True {
              n863 = global read "全局 小时数据发送次数.vi" "小时数据发送次数"() -> (w2080:i32)
              n864 = Increment(x=w2080) -> (x+1=w2079:i32)
              n865 = global write "全局 小时数据发送次数.vi" "小时数据发送次数"(w2079) -> ()
            }
          }
        }
        frame "返回执行结果" {
        }
      }
    }
    frame "提取实时数据" {
      # "叶绿素"
      # "浊度"
      # "电导率"
      # "提取实时数据"
      n866 = global read "全局 小时数据发送次数.vi" "小时数据发送次数"() -> (w2089:i32)
      n867 = global read "全局 小时数据发送次数.vi" "小时数据发送次数"() -> (w2096:i32)
      n868 = global read "全局 小时数据发送次数.vi" "小时数据发送次数"() -> (w2090:i32)
      n869 = global read "全局 小时数据发送次数.vi" "小时数据发送次数"() -> (w2091:i32)
      n870 = global read "全局 小时数据发送次数.vi" "小时数据发送次数"() -> (w2097:i32)
      n871 = global read "全局 小时数据发送次数.vi" "小时数据发送次数"() -> (w2111:i32)
      n872 = global read "全局 小时数据发送次数.vi" "小时数据发送次数"() -> (w2107:i32)
      n873 = global read "全局 小时数据发送次数.vi" "小时数据发送次数"() -> (w2101:i32)
      n874 = global read "全局 小时数据发送次数.vi" "小时数据发送次数"() -> (w2119:i32)
      n875 = global read "全局 小时数据发送次数.vi" "小时数据发送次数"() -> (w2121:i32)
      n876 = global read "全局 小时数据发送次数.vi" "小时数据发送次数"() -> (w2115:i32)
      n877 = global read "全局 小时数据发送次数.vi" "小时数据发送次数"() -> (w2103:i32)
      n878 = global read "全局 小时数据发送次数.vi" "小时数据发送次数"() -> (w2117:i32)
      n879 = global read "全局 小时数据发送次数.vi" "小时数据发送次数"() -> (w2100:i32)
      n880 = global read "全局 小时数据发送次数.vi" "小时数据发送次数"() -> (w2105:i32)
      n881 = global read "全局 小时数据发送次数.vi" "小时数据发送次数"() -> (w2113:i32)
      n882 = global read "全局 小时数据发送次数.vi" "小时数据发送次数"() -> (w2108:i32)
      n883 = Index Array(array=w2086, index (row)=w2089) -> (element=w2083:string[])  [unwired: 1 in]
      n884 = Index Array(array=w2094, index (row)=w2096) -> (element=w2092:string[])  [unwired: 1 in]
      n885 = Index Array(array=w2087, index (row)=w2090) -> (element=w2084:string[])  [unwired: 1 in]
      n886 = Index Array(array=w2088, index (row)=w2091) -> (element=w2085:string[])  [unwired: 1 in]
      n887 = Index Array(array=w2095, index (row)=w2097) -> (element=w2093:string[])  [unwired: 1 in]
      n888 = Index Array(array=w2130, index (row)=w2111) -> (element=w2110:string[])  [unwired: 1 in]
      n889 = Index Array(array=w2135, index (row)=w2121) -> (element=w2120:string[])  [unwired: 1 in]
      n890 = Index Array(array=w2134, index (row)=w2119) -> (element=w2118:string[])  [unwired: 1 in]
      n891 = Index Array(array=w2127, index (row)=w2105) -> (element=w2104:string[])  [unwired: 1 in]
      n892 = Index Array(array=w2129, index (row)=w2108) -> (element=w2109:string[])  [unwired: 1 in]
      n893 = Index Array(array=w2133, index (row)=w2117) -> (element=w2116:string[])  [unwired: 1 in]
      n894 = Index Array(array=w2128, index (row)=w2107) -> (element=w2106:string[])  [unwired: 1 in]
      n895 = Index Array(array=w2132, index (row)=w2115) -> (element=w2114:string[])  [unwired: 1 in]
      n896 = Index Array(array=w2126, index (row)=w2103) -> (element=w2102:string[])  [unwired: 1 in]
      n897 = Index Array(array=w2125, index (row)=w2101) -> (element=w2099:string[])  [unwired: 1 in]
      n898 = Index Array(array=w2131, index (row)=w2113) -> (element=w2112:string[])  [unwired: 1 in]
      n899 = Index Array(array=w2124, index (row)=w2100) -> (element=w2098:string[])  [unwired: 1 in]
      n900 = global read "全局1.vi" "枚举"() -> (w2122:enum16{"返回请求应答", "上传数据", "返回执行结果"})
      n901 = case shown="\"上传数据\"" w2122 {
        tunnel: ["QnRtn=1" w2199 "ExeRtn=1"] -> w2123
        tunnel: w2120 -> [_ w2274 _]
        tunnel: w2116 -> [_ w2289 _]
        tunnel: w2114 -> [_ w2288 _]
        tunnel: w2112 -> [_ w2287 _]
        tunnel: w2118 -> [_ w2285 _]
        tunnel: w2110 -> [_ w2273 _]
        tunnel: w2109 -> [_ w2279 _]
        tunnel: w2106 -> [_ w2276 _]
        tunnel: w2104 -> [_ w2275 _]
        tunnel: w2102 -> [_ w2272 _]
        tunnel: w2099 -> [_ w2271 _]
        tunnel: w2098 -> [_ w2270 _]
        tunnel: w2093 -> [_ w2209 _]
        tunnel: w2092 -> [_ w2208 _]
        tunnel: w2085 -> [_ w2147 _]
        tunnel: w2084 -> [_ w2146 _]
        tunnel: w2083 -> [_ w2145 _]
        frame "返回请求应答", Default {
          n902 = global read "全局 数据数组大小.vi" "数据数组大小"() -> (w2136:i32)
          n903 = Equal To 0?(x=w2136) -> (x = 0?=w2137:bool)
          n904 = case shown="假" w2137 {
            frame False {
            }
            frame True {
              n905 = global read "全局 小时数据发送次数.vi" "小时数据发送次数"() -> (w2140:i32)
              n906 = Increment(x=w2140) -> (x+1=w2139:i32)
              n907 = global write "全局 小时数据发送次数.vi" "小时数据发送次数"(w2139) -> ()
            }
          }
        }
        frame "上传数据" {
          (unwired) 2 ("数据精度")
          (unwired) 3 ("数据精度")
          (unwired) 3 ("数据精度")
          (unwired) "-Rtd=" ("数据类型")
          (unwired) 3 ("数据精度")
          (unwired) 3 ("精度")
          # "瞬时流量"
          # "流速"
          # "水位"
          # "盐度"
          # "总铜"
          # "PH"
          # "总氮"
          # "总磷"
          # "藻密度"
          # "叶绿素"
          # "浊度"
          # "电导率"
          # "DO"
          # "CODCr"
          # "水温"
          # "NH3"
          # "CODMn"
          n908 = Index Array(array=w2146, index #2=1 ("索引")) -> (element #2=w2148:string)  [unwired: 1 in, 1 out]
          n909 = Index Array(array=w2145, index #2=1 ("索引")) -> (element #2=w2144:string)  [unwired: 1 in, 1 out]
          n910 = Index Array(array=w2147, index #2=1 ("索引")) -> (element #2=w2149:string)  [unwired: 1 in, 1 out]
          n911 = Index Array(array=w2208, index #2=1 ("索引")) -> (element #2=w2166:string)  [unwired: 1 in, 1 out]
          n912 = Index Array(array=w2209, index #2=1 ("索引")) -> (element #2=w2165:string)  [unwired: 1 in, 1 out]
          n913 = Index Array(array=w2273, index #2=1 ("索引"), index #3=5 ("索引")) -> (element #2=w2214:string)  [unwired: 1 in, 2 out]
          n914 = Index Array(array=w2287, index #1=0 ("索引"), index #2=1 ("索引"), index #3=5 ("索引")) -> (element #2=w2216:string)  [unwired: 2 out]
          n915 = Index Array(array=w2271, index #2=1 ("索引"), index #3=5 ("索引")) -> (element #2=w2222:string)  [unwired: 1 in, 2 out]
          n916 = Index Array(array=w2270, index #2=1 ("索引"), index #3=5 ("索引")) -> (element #2=w2220:string)  [unwired: 1 in, 2 out]
          n917 = Index Array(array=w2275, index #2=1 ("索引"), index #3=5 ("索引")) -> (element #2=w2243:string)  [unwired: 1 in, 2 out]
          n918 = Index Array(array=w2276, index #2=1 ("索引"), index #3=5 ("索引")) -> (element #2=w2234:string)  [unwired: 1 in, 2 out]
          n919 = Index Array(array=w2272, index #2=1 ("索引"), index #3=5 ("索引")) -> (element #2=w2225:string)  [unwired: 1 in, 2 out]
          n920 = Index Array(array=w2288, index #1=0 ("索引"), index #2=1 ("索引"), index #3=5 ("索引")) -> (element #2=w2218:string)  [unwired: 2 out]
          n921 = Index Array(array=w2274, index #1=0 ("索引"), index #2=1 ("索引"), index #3=5 ("索引")) -> (element #1=w2213:string, element #2=w2249:string)  [unwired: 1 out]
          n922 = Index Array(array=w2285, index #1=0 ("索引"), index #2=1 ("索引"), index #3=5 ("索引")) -> (element #2=w2245:string)  [unwired: 2 out]
          n923 = Index Array(array=w2279, index #1=0 ("索引"), index #2=1 ("索引"), index #3=5 ("索引")) -> (element #2=w2238:string)  [unwired: 2 out]
          n924 = Index Array(array=w2289, index #1=0 ("索引"), index #2=1 ("索引"), index #3=5 ("索引")) -> (element #2=w2236:string)  [unwired: 2 out]
          n925 = global read "断电保存全局.vi" "数据发送协议"() -> (w2184:enum16{"2005-212协议", "2017-212协议"})
          n926 = global read "断电保存全局.vi" "数据发送协议"() -> (w2159:enum16{"2005-212协议", "2017-212协议"})
          n927 = global read "断电保存全局.vi" "数据发送协议"() -> (w2156:enum16{"2005-212协议", "2017-212协议"})
          n928 = global read "断电保存全局.vi" "数据发送协议"() -> (w2151:enum16{"2005-212协议", "2017-212协议"})
          n929 = global read "断电保存全局.vi" "数据发送协议"() -> (w2188:enum16{"2005-212协议", "2017-212协议"})
          n930 = case shown="\"2005-212协议\"" w2184 {
            tunnel: ["313" ("污染物编码") "w21011" ("污染物编码")] -> w2183
            tunnel: ["466" ("污染物编码") "w21001" ("污染物编码")] -> w2182
            tunnel: ["302" ("污染物编码") "w01001" ("污染物编码")] -> w2181
            frame "2005-212协议" {
            }
            frame "2017-212协议", Default {
            }
          }
          n931 = global read "断电保存全局.vi" "数据发送协议"() -> (w2189:enum16{"2005-212协议", "2017-212协议"})
          n932 = global read "断电保存全局.vi" "数据发送协议"() -> (w2195:enum16{"2005-212协议", "2017-212协议"})
          n933 = global read "断电保存全局.vi" "数据发送协议"() -> (w2196:enum16{"2005-212协议", "2017-212协议"})
          n934 = case shown="\"2005-212协议\"" w2159 {
            tunnel: ["490" ("污染物编码") "w01003" ("污染物编码")] -> w2158
            frame "2005-212协议" {
            }
            frame "2017-212协议", Default {
            }
          }
          n935 = global read "断电保存全局.vi" "数据发送协议"() -> (w2190:enum16{"2005-212协议", "2017-212协议"})
          n936 = global read "断电保存全局.vi" "数据发送协议"() -> (w2194:enum16{"2005-212协议", "2017-212协议"})
          n937 = case shown="\"2005-212协议\"" w2156 {
            tunnel: ["497" ("污染物编码") "w01003" ("污染物编码")] -> w2157
            frame "2005-212协议" {
            }
            frame "2017-212协议", Default {
            }
          }
          n938 = case shown="\"2005-212协议\"" w2151 {
            tunnel: ["492" ("污染物编码") "w01003" ("污染物编码")] -> w2150
            frame "2005-212协议" {
            }
            frame "2017-212协议", Default {
            }
          }
          n939 = global read "断电保存全局.vi" "数据发送协议"() -> (w2198:enum16{"2005-212协议", "2017-212协议"})
          n940 = case shown="\"2005-212协议\"" w2188 {
            tunnel: ["465" ("污染物编码") "w01003" ("污染物编码")] -> w2185
            frame "2005-212协议" {
            }
            frame "2017-212协议", Default {
            }
          }
          n941 = case shown="\"2005-212协议\"" w2189 {
            tunnel: ["463" ("污染物编码") "w01014" ("污染物编码")] -> w2186
            frame "2005-212协议" {
            }
            frame "2017-212协议", Default {
            }
          }
          n942 = case shown="\"2005-212协议\"" w2195 {
            tunnel: ["316" ("污染物编码") "w01018" ("污染物编码")] -> w2191
            frame "2005-212协议" {
            }
            frame "2017-212协议", Default {
            }
          }
          n943 = case shown="\"2005-212协议\"" w2190 {
            tunnel: ["315" ("污染物编码") "w01009" ("污染物编码")] -> w2187
            frame "2005-212协议" {
            }
            frame "2017-212协议", Default {
            }
          }
          n944 = case shown="\"2005-212协议\"" w2196 {
            tunnel: ["311" ("污染物编码") "w21003" ("污染物编码")] -> w2193
            frame "2005-212协议" {
            }
            frame "2017-212协议", Default {
            }
          }
          n945 = case shown="\"2005-212协议\"" w2194 {
            tunnel: ["301" ("污染物编码") "w01010" ("污染物编码")] -> w2192
            frame "2005-212协议" {
            }
            frame "2017-212协议", Default {
            }
          }
          n946 = case shown="\"2005-212协议\"" w2198 {
            tunnel: ["314" ("污染物编码") "w01019" ("污染物编码")] -> w2197
            frame "2005-212协议" {
            }
            frame "2017-212协议", Default {
            }
          }
          n947 = call "规范时间戳.vi"("字符串"=w2213) -> ("result string"=w2212:string)  [unwired: 10 in]
          n948 = call "数据编码整合输出.vi"("数据标识"="N" ("字符串"), "数据类型"="-Rtd=", "污染物编码"=w2158, "数据值"=w2149) -> ("编码输出"=w2143:string)  [unwired: 7 in]
          n949 = call "数据编码整合输出.vi"("数据标识"="N" ("字符串"), "数据类型"="-Rtd=", "污染物编码"="w01015", "数据值"=w2166) -> ("编码输出"=w2202:string)  [unwired: 7 in]
          n950 = call "数据编码整合输出.vi"("数据标识"="N" ("字符串"), "数据类型"="-Rtd=", "污染物编码"=w2157, "数据值"=w2148) -> ("编码输出"=w2142:string)  [unwired: 7 in]
          n951 = call "数据编码整合输出.vi"("数据标识"="N" ("字符串"), "数据类型"="-Rtd=", "污染物编码"=w2150, "数据值"=w2144) -> ("编码输出"=w2141:string)  [unwired: 7 in]
          n952 = call "数据编码整合输出.vi"("数据标识"="N" ("字符串"), "数据类型"="-Rtd=", "污染物编码"="w20122", "数据值"=w2165) -> ("编码输出"=w2203:string)  [unwired: 7 in]
          n953 = call "数据编码整合输出.vi"("数据标识"="N" ("字符串"), "数据类型"="-Rtd=", "污染物编码"=w2181, "数据值"=w2214) -> ("编码输出"=w2215:string)  [unwired: 7 in]
          n954 = call "数据编码整合输出.vi"("数据标识"="N" ("字符串"), "数据类型"="-Rtd=", "污染物编码"=w2197, "数据值"=w2249) -> ("编码输出"=w2248:string)  [unwired: 7 in]
          n955 = call "数据编码整合输出.vi"("数据标识"="N" ("字符串"), "数据类型"="-Rtd=", "污染物编码"=w2193, "数据值"=w2245) -> ("编码输出"=w2244:string)  [unwired: 7 in]
          n956 = call "数据编码整合输出.vi"("数据标识"="N" ("字符串"), "数据类型"="-Rtd=", "污染物编码"=w2182, "数据值"=w2216) -> ("编码输出"=w2217:string)  [unwired: 7 in]
          n957 = call "数据编码整合输出.vi"("数据标识"="N" ("字符串"), "数据类型"="-Rtd=", "污染物编码"="w01016", "数据值"=w2222) -> ("编码输出"=w2223:string)  [unwired: 7 in]
          n958 = call "数据编码整合输出.vi"("数据标识"="N" ("字符串"), "数据类型"="-Rtd=", "污染物编码"="w19011", "数据值"=w2220) -> ("编码输出"=w2221:string)  [unwired: 7 in]
          n959 = call "数据编码整合输出.vi"("数据标识"="N" ("字符串"), "污染物编码"=w2183, "数据值"=w2218) -> ("编码输出"=w2219:string)  [unwired: 8 in]
          n960 = call "数据编码整合输出.vi"("数据标识"="N" ("字符串"), "数据类型"="-Rtd=", "污染物编码"=w2191, "数据值"=w2238) -> ("编码输出"=w2237:string)  [unwired: 7 in]
          n961 = call "数据编码整合输出.vi"("数据标识"="N" ("字符串"), "数据类型"="-Rtd=", "污染物编码"=w2192, "数据值"=w2243) -> ("编码输出"=w2242:string)  [unwired: 7 in]
          n962 = call "数据编码整合输出.vi"("数据标识"="N" ("字符串"), "数据类型"="-Rtd=", "污染物编码"=w2185, "数据值"=w2225) -> ("编码输出"=w2224:string)  [unwired: 7 in]
          n963 = call "数据编码整合输出.vi"("数据标识"="N" ("字符串"), "数据类型"="-Rtd=", "污染物编码"=w2186, "数据值"=w2234) -> ("编码输出"=w2233:string)  [unwired: 7 in]
          n964 = call "数据编码整合输出.vi"("数据标识"="N" ("字符串"), "数据类型"="-Rtd=", "污染物编码"=w2187, "数据值"=w2236) -> ("编码输出"=w2235:string)  [unwired: 7 in]
          n965 = Empty String/Path?(string/path=w2212) -> (empty?=w2201:bool)
          n966 = Format Into String(format string="DataTime=%s;%s%s%s%s%s%s%s%s%s%s%s%s%s%s%s%s%s" ("格式字符串"), w2212, w2248, w2244, w2242, w2237, w2235, w2233, w2224, w2223, w2221, w2219, w2217, w2215, w2203, w2202, w2143, w2142, w2141) -> (resulting string=w2200:string)  [unwired: 2 in, 1 out]
          n967 = case shown="真" w2201 {
            tunnel: [w2320 ""] -> w2199
            tunnel: w2200 -> [w2320 _]
            frame False {
              n968 = global read "全局 小时数据发送次数.vi" "小时数据发送次数"() -> (w2322:i32)
              n969 = Increment(x=w2322) -> (x+1=w2321:i32)
              n970 = global write "全局 小时数据发送次数.vi" "小时数据发送次数"(w2321) -> ()
            }
            frame True {
              n971 = global read "全局 小时数据发送次数.vi" "小时数据发送次数"() -> (w2324:i32)
              n972 = Increment(x=w2324) -> (x+1=w2323:i32)
              n973 = global write "全局 小时数据发送次数.vi" "小时数据发送次数"(w2323) -> ()
            }
          }
        }
        frame "返回执行结果" {
        }
      }
    }
    frame "核查数据" {
      # "提取标样核查数据"
      n974 = global read "全局 小时数据发送次数.vi" "小时数据发送次数"() -> (w2329:i32)
      n975 = global read "全局 小时数据发送次数.vi" "小时数据发送次数"() -> (w2346:i32)
      n976 = global read "全局 小时数据发送次数.vi" "小时数据发送次数"() -> (w2348:i32)
      n977 = global read "全局 小时数据发送次数.vi" "小时数据发送次数"() -> (w2344:i32)
      n978 = global read "全局 小时数据发送次数.vi" "小时数据发送次数"() -> (w2340:i32)
      n979 = global read "全局 小时数据发送次数.vi" "小时数据发送次数"() -> (w2332:i32)
      n980 = global read "全局 小时数据发送次数.vi" "小时数据发送次数"() -> (w2338:i32)
      n981 = global read "全局 小时数据发送次数.vi" "小时数据发送次数"() -> (w2335:i32)
      n982 = global read "全局 小时数据发送次数.vi" "小时数据发送次数"() -> (w2342:i32)
      n983 = Index Array(array=w2327, index (row)=w2329) -> (element=w2328:string[])  [unwired: 1 in]
      n984 = Index Array(array=w2354, index (row)=w2346) -> (element=w2345:string[])  [unwired: 1 in]
      n985 = Index Array(array=w2355, index (row)=w2348) -> (element=w2347:string[])  [unwired: 1 in]
      n986 = Index Array(array=w2353, index (row)=w2344) -> (element=w2343:string[])  [unwired: 1 in]
      n987 = Index Array(array=w2350, index (row)=w2340) -> (element=w2339:string[])  [unwired: 1 in]
      n988 = Index Array(array=w2330, index (row)=w2332) -> (element=w2331:string[])  [unwired: 1 in]
      n989 = Index Array(array=w2337, index (row)=w2338) -> (element=w2336:string[])  [unwired: 1 in]
      n990 = Index Array(array=w2333, index (row)=w2335) -> (element=w2334:string[])  [unwired: 1 in]
      n991 = Index Array(array=w2352, index (row)=w2342) -> (element=w2341:string[])  [unwired: 1 in]
      n992 = global read "全局1.vi" "枚举"() -> (w2349:enum16{"返回请求应答", "上传数据", "返回执行结果"})
      n993 = case shown="\"上传数据\"" w2349 {
        tunnel: ["QnRtn=1" w2406 "ExeRtn=1"] -> w2351
        tunnel: w2347 -> [_ w2426 _]
        tunnel: w2343 -> [_ w2425 _]
        tunnel: w2341 -> [_ w2424 _]
        tunnel: w2345 -> [_ w2422 _]
        tunnel: w2339 -> [_ w2410 _]
        tunnel: w2336 -> [_ w2385 _]
        tunnel: w2334 -> [_ w2377 _]
        tunnel: w2331 -> [_ w2373 _]
        tunnel: w2328 -> [_ w2365 _]
        frame "返回请求应答", Default {
          n994 = global read "全局 数据数组大小.vi" "数据数组大小"() -> (w2357:i32)
          n995 = Equal To 0?(x=w2357) -> (x = 0?=w2356:bool)
          n996 = case shown="真" w2356 {
            frame False {
            }
            frame True {
              n997 = global read "全局 小时数据发送次数.vi" "小时数据发送次数"() -> (w2360:i32)
              n998 = Increment(x=w2360) -> (x+1=w2359:i32)
              n999 = global write "全局 小时数据发送次数.vi" "小时数据发送次数"(w2359) -> ()
            }
          }
        }
        frame "上传数据" {
          # "将非空数组的时间戳写入"
          n1000 = Index Array(array=w2365, index #1=0 ("索引"), index #2=3 ("索引"), index #3=7 ("索引")) -> (element #2=w2366:string, element #3=w2367:string)  [unwired: 1 out]
          n1001 = Index Array(array=w2373, index #1=0 ("索引"), index #2=3 ("索引"), index #3=7 ("索引")) -> (element #2=w2372:string, element #3=w2371:string)  [unwired: 1 out]
          n1002 = Index Array(array=w2385, index #1=0 ("索引"), index #2=3 ("索引"), index #3=7 ("索引")) -> (element #2=w2384:string, element #3=w2383:string)  [unwired: 1 out]
          n1003 = Index Array(array=w2377, index #1=0 ("索引"), index #2=3 ("索引"), index #3=7 ("索引")) -> (element #2=w2378:string, element #3=w2379:string)  [unwired: 1 out]
          n1004 = Index Array(array=w2424, index #1=0 ("索引"), index #2=3 ("索引"), index #3=7 ("索引")) -> (element #2=w2394:string, element #3=w2393:string)  [unwired: 1 out]
          n1005 = Index Array(array=w2422, index #1=0 ("索引"), index #2=3 ("索引"), index #3=7 ("索引")) -> (element #1=w2405:string, element #2=w2400:string, element #3=w2399:string)
          n1006 = Index Array(array=w2426, index #1=0 ("索引"), index #2=3 ("索引"), index #3=7 ("索引")) -> (element #2=w2403:string, element #3=w2402:string)  [unwired: 1 out]
          n1007 = Index Array(array=w2425, index #1=0 ("索引"), index #2=3 ("索引"), index #3=7 ("索引")) -> (element #2=w2396:string, element #3=w2395:string)  [unwired: 1 out]
          n1008 = Index Array(array=w2410, index #1=0 ("索引"), index #2=3 ("索引"), index #3=7 ("索引")) -> (element #2=w2389:string, element #3=w2391:string)  [unwired: 1 out]
          n1009 = case shown="\"真\", 默认" w2366 {
            tunnel: [w2430 w2441] -> w2361
            tunnel: w2366 -> [w2430 w2435]
            tunnel: w2367 -> [_ w2434]
            frame "" {
            }
            frame "真", Default {
              n1010 = call "核查数据编码整合输出.vi"("字段结束"=FALSE, "数据标识"="N" ("字符串"), "数据类型"="-Check=", "污染物编码"="w01003", "数据值"=w2435) -> ("编码输出"=w2442:string)  [unwired: 6 in]
              n1011 = call "核查数据编码整合输出.vi"("字段结束"=TRUE, "数据标识"="N" ("字符串"), "数据类型"="-StandardValue=", "污染物编码"="w01003", "数据精度"=2, "数据值"=w2434) -> ("编码输出"=w2438:string)  [unwired: 5 in]
              n1012 = Concatenate Strings(w2442, w2438) -> (w2441:string)
            }
          }
          n1013 = case shown="\"真\", 默认" w2378 {
            tunnel: w2378 -> [w2460 w2473]
            tunnel: [w2460 w2470] -> w2363
            tunnel: w2379 -> [_ w2466]
            frame "" {
            }
            frame "真", Default {
              n1014 = call "核查数据编码整合输出.vi"("字段结束"=FALSE, "数据标识"="N" ("字符串"), "数据类型"="-Check=", "污染物编码"="w01009", "数据值"=w2473) -> ("编码输出"=w2471:string)  [unwired: 6 in]
              n1015 = call "核查数据编码整合输出.vi"("字段结束"=TRUE, "数据标识"="N" ("字符串"), "数据类型"="-StandardValue=", "污染物编码"="w01009", "数据精度"=2, "数据值"=w2466) -> ("编码输出"=w2467:string)  [unwired: 5 in]
              n1016 = Concatenate Strings(w2471, w2467) -> (w2470:string)
            }
          }
          n1017 = case shown="\"真\", 默认" w2372 {
            tunnel: [w2445 w2456] -> w2362
            tunnel: w2372 -> [w2445 w2448]
            tunnel: w2371 -> [_ w2447]
            frame "" {
            }
            frame "真", Default {
              n1018 = call "核查数据编码整合输出.vi"("字段结束"=FALSE, "数据标识"="N" ("字符串"), "数据类型"="-Check=", "污染物编码"="w01014", "数据值"=w2448) -> ("编码输出"=w2457:string)  [unwired: 6 in]
              n1019 = call "核查数据编码整合输出.vi"("字段结束"=TRUE, "数据标识"="N" ("字符串"), "数据类型"="-StandardValue=", "污染物编码"="w01014", "数据精度"=2, "数据值"=w2447) -> ("编码输出"=w2453:string)  [unwired: 5 in]
              n1020 = Concatenate Strings(w2457, w2453) -> (w2456:string)
            }
          }
          n1021 = case shown="\"真\", 默认" w2384 {
            tunnel: w2384 -> [w2475 w2488]
            tunnel: [w2475 w2485] -> w2364
            tunnel: w2383 -> [_ w2481]
            frame "" {
            }
            frame "真", Default {
              n1022 = call "核查数据编码整合输出.vi"("字段结束"=FALSE, "数据标识"="N" ("字符串"), "数据类型"="-Check=", "污染物编码"="w01001", "数据值"=w2488) -> ("编码输出"=w2486:string)  [unwired: 6 in]
              n1023 = call "核查数据编码整合输出.vi"("字段结束"=TRUE, "数据标识"="N" ("字符串"), "数据类型"="-StandardValue=", "污染物编码"="w01001", "数据精度"=2, "数据值"=w2481) -> ("编码输出"=w2482:string)  [unwired: 5 in]
              n1024 = Concatenate Strings(w2486, w2482) -> (w2485:string)
            }
          }
          n1025 = case shown="\"真\", 默认" w2403 {
            tunnel: w2403 -> [w2550 w2563]
            tunnel: [w2550 w2559] -> w2401
            tunnel: w2402 -> [_ w2554]
            frame "" {
            }
            frame "真", Default {
              # "CODMn"
              n1026 = call "核查数据编码整合输出.vi"("字段结束"=FALSE, "数据标识"="N" ("字符串"), "数据类型"="-Check=", "污染物编码"="w01019", "数据值"=w2563) -> ("编码输出"=w2560:string)  [unwired: 6 in]
              n1027 = call "核查数据编码整合输出.vi"("字段结束"=TRUE, "数据标识"="N" ("字符串"), "数据类型"="-StandardValue=", "污染物编码"="w01019", "数据精度"=2, "数据值"=w2554) -> ("编码输出"=w2555:string)  [unwired: 5 in]
              n1028 = Concatenate Strings(w2560, w2555) -> (w2559:string)
            }
          }
          n1029 = case shown="\"真\", 默认" w2389 {
            tunnel: w2389 -> [w2490 w2503]
            tunnel: [w2490 w2500] -> w2390
            tunnel: w2391 -> [_ w2496]
            frame "" {
            }
            frame "真", Default {
              n1030 = call "核查数据编码整合输出.vi"("字段结束"=FALSE, "数据标识"="N" ("字符串"), "数据类型"="-Check=", "污染物编码"="w01018", "数据值"=w2503) -> ("编码输出"=w2501:string)  [unwired: 6 in]
              n1031 = call "核查数据编码整合输出.vi"("字段结束"=TRUE, "数据标识"="N" ("字符串"), "数据类型"="-StandardValue=", "污染物编码"="w01018", "数据精度"=2, "数据值"=w2496) -> ("编码输出"=w2497:string)  [unwired: 5 in]
              n1032 = Concatenate Strings(w2501, w2497) -> (w2500:string)
            }
          }
          n1033 = case shown="\"真\", 默认" w2400 {
            tunnel: w2400 -> [w2535 w2548]
            tunnel: [w2535 w2545] -> w2398
            tunnel: w2399 -> [_ w2541]
            frame "" {
            }
            frame "真", Default {
              n1034 = call "核查数据编码整合输出.vi"("字段结束"=FALSE, "数据标识"="N" ("字符串"), "数据类型"="-Check=", "污染物编码"="w21003", "数据值"=w2548) -> ("编码输出"=w2546:string)  [unwired: 6 in]
              n1035 = call "核查数据编码整合输出.vi"("字段结束"=TRUE, "数据标识"="N" ("字符串"), "数据类型"="-StandardValue=", "污染物编码"="w21003", "数据精度"=2, "数据值"=w2541) -> ("编码输出"=w2542:string)  [unwired: 5 in]
              n1036 = Concatenate Strings(w2546, w2542) -> (w2545:string)
            }
          }
          n1037 = case shown="\"真\", 默认" w2396 {
            tunnel: w2396 -> [w2520 w2533]
            tunnel: [w2520 w2530] -> w2397
            tunnel: w2395 -> [_ w2526]
            frame "" {
            }
            frame "真", Default {
              n1038 = call "核查数据编码整合输出.vi"("字段结束"=FALSE, "数据标识"="N" ("字符串"), "数据类型"="-Check=", "污染物编码"="w21011", "数据值"=w2533) -> ("编码输出"=w2531:string)  [unwired: 6 in]
              n1039 = call "核查数据编码整合输出.vi"("字段结束"=TRUE, "数据标识"="N" ("字符串"), "数据类型"="-StandardValue=", "污染物编码"="w21011", "数据精度"=2, "数据值"=w2526) -> ("编码输出"=w2527:string)  [unwired: 5 in]
              n1040 = Concatenate Strings(w2531, w2527) -> (w2530:string)
            }
          }
          n1041 = case shown="\"真\", 默认" w2394 {
            tunnel: w2394 -> [w2505 w2518]
            tunnel: [w2505 w2515] -> w2392
            tunnel: w2393 -> [_ w2511]
            frame "" {
            }
            frame "真", Default {
              n1042 = call "核查数据编码整合输出.vi"("字段结束"=FALSE, "数据标识"="N" ("字符串"), "数据类型"="-Check=", "污染物编码"="w21001", "数据值"=w2518) -> ("编码输出"=w2516:string)  [unwired: 6 in]
              n1043 = call "核查数据编码整合输出.vi"("字段结束"=TRUE, "数据标识"="N" ("字符串"), "数据类型"="-StandardValue=", "污染物编码"="w21001", "数据精度"=2, "数据值"=w2511) -> ("编码输出"=w2512:string)  [unwired: 5 in]
              n1044 = Concatenate Strings(w2516, w2512) -> (w2515:string)
            }
          }
          n1045 = call "规范时间戳.vi"("字符串"=w2405) -> ("result string"=w2404:string)  [unwired: 10 in]
          n1046 = Format Into String(format string="DataTime=%s;%s%s%s%s%s%s%s%s%s" ("格式字符串"), w2404, w2401, w2398, w2397, w2392, w2390, w2364, w2363, w2362, w2361) -> (resulting string=w2407:string)  [unwired: 2 in, 1 out]
          n1047 = Empty String/Path?(string/path=w2404) -> (empty?=w2408:bool)
          n1048 = case shown="假" w2408 {
            tunnel: [w2567 ""] -> w2406
            tunnel: w2407 -> [w2567 _]
            frame False {
              n1049 = global read "全局 小时数据发送次数.vi" "小时数据发送次数"() -> (w2566:i32)
              n1050 = Increment(x=w2566) -> (x+1=w2565:i32)
              n1051 = global write "全局 小时数据发送次数.vi" "小时数据发送次数"(w2565) -> ()
            }
            frame True {
              n1052 = global read "全局 小时数据发送次数.vi" "小时数据发送次数"() -> (w2569:i32)
              n1053 = Increment(x=w2569) -> (x+1=w2568:i32)
              n1054 = global write "全局 小时数据发送次数.vi" "小时数据发送次数"(w2568) -> ()
            }
          }
        }
        frame "返回执行结果" {
        }
      }
    }
    frame "空白测试", "跨度核查", "零点核查" {
      # "提取空白测试数据/零点核查数据/跨度核查数据"
      n1055 = global read "全局 小时数据发送次数.vi" "小时数据发送次数"() -> (w2579:i32)
      n1056 = global read "全局 小时数据发送次数.vi" "小时数据发送次数"() -> (w2581:i32)
      n1057 = global read "全局 小时数据发送次数.vi" "小时数据发送次数"() -> (w2577:i32)
      n1058 = global read "全局 小时数据发送次数.vi" "小时数据发送次数"() -> (w2573:i32)
      n1059 = global read "全局 小时数据发送次数.vi" "小时数据发送次数"() -> (w2575:i32)
      n1060 = Index Array(array=w2587, index (row)=w2579) -> (element=w2578:string[])  [unwired: 1 in]
      n1061 = Index Array(array=w2588, index (row)=w2581) -> (element=w2580:string[])  [unwired: 1 in]
      n1062 = Index Array(array=w2586, index (row)=w2577) -> (element=w2576:string[])  [unwired: 1 in]
      n1063 = Index Array(array=w2583, index (row)=w2573) -> (element=w2572:string[])  [unwired: 1 in]
      n1064 = Index Array(array=w2585, index (row)=w2575) -> (element=w2574:string[])  [unwired: 1 in]
      n1065 = global read "全局1.vi" "枚举"() -> (w2582:enum16{"返回请求应答", "上传数据", "返回执行结果"})
      n1066 = case shown="\"上传数据\"" w2582 {
        tunnel: ["QnRtn=1" w2620 "ExeRtn=1"] -> w2584
        tunnel: w2580 -> [_ w2640 _]
        tunnel: w2576 -> [_ w2639 _]
        tunnel: w2574 -> [_ w2638 _]
        tunnel: w2578 -> [_ w2636 _]
        tunnel: w2572 -> [_ w2624 _]
        frame "返回请求应答", Default {
          (unwired) 0 ("当前包数")
          n1067 = global read "全局 数据数组大小.vi" "数据数组大小"() -> (w2590:i32)
          n1068 = Equal To 0?(x=w2590) -> (x = 0?=w2589:bool)
          n1069 = case shown="真" w2589 {
            frame False {
            }
            frame True {
              n1070 = global read "全局 小时数据发送次数.vi" "小时数据发送次数"() -> (w2593:i32)
              n1071 = Increment(x=w2593) -> (x+1=w2592:i32)
              n1072 = global write "全局 小时数据发送次数.vi" "小时数据发送次数"(w2592) -> ()
            }
          }
        }
        frame "上传数据" {
          # "将非空数组的时间戳写入"
          n1073 = Index Array(array=w2638, index #1=0 ("索引"), index #2=3 ("索引"), index #3=7 ("索引")) -> (element #2=w2601:string, element #3=w2600:string)  [unwired: 1 out]
          n1074 = Index Array(array=w2636, index #1=0 ("索引"), index #2=3 ("索引"), index #3=7 ("索引")) -> (element #1=w2619:string, element #2=w2611:string, element #3=w2610:string)
          n1075 = Index Array(array=w2640, index #1=0 ("索引"), index #2=3 ("索引"), index #3=7 ("索引")) -> (element #2=w2616:string, element #3=w2615:string)  [unwired: 1 out]
          n1076 = Index Array(array=w2639, index #1=0 ("索引"), index #2=3 ("索引"), index #3=7 ("索引")) -> (element #2=w2606:string, element #3=w2605:string)  [unwired: 1 out]
          n1077 = Index Array(array=w2624, index #1=0 ("索引"), index #2=3 ("索引"), index #3=7 ("索引")) -> (element #2=w2596:string, element #3=w2595:string)  [unwired: 1 out]
          n1078 = call "规范时间戳.vi"("字符串"=w2619) -> ("result string"=w2618:string)  [unwired: 10 in]
          n1079 = call "零点跨度数据组合 (子VI).vi"("span value"="0", "standard value"=w2615, "check value"=w2616, "污染物编码"="w01019") -> ("组合输出"=w2614:string)  [unwired: 7 in]
          n1080 = call "零点跨度数据组合 (子VI).vi"("standard value"=w2595, "check value"=w2596, "污染物编码"="w01018") -> ("组合输出"=w2594:string)  [unwired: 8 in]
          n1081 = call "零点跨度数据组合 (子VI).vi"("span value"="0", "standard value"=w2600, "check value"=w2601, "污染物编码"="w21001") -> ("组合输出"=w2598:string)  [unwired: 7 in]
          n1082 = call "零点跨度数据组合 (子VI).vi"("span value"="0", "standard value"=w2610, "check value"=w2611, "污染物编码"="w21003") -> ("组合输出"=w2608:string)  [unwired: 7 in]
          n1083 = call "零点跨度数据组合 (子VI).vi"("span value"="0", "standard value"=w2605, "check value"=w2606, "污染物编码"="w21011") -> ("组合输出"=w2604:string)  [unwired: 7 in]
          n1084 = Format Into String(format string="DataTime=%s;%s%s%s%s%s" ("格式字符串"), w2618, w2614, w2608, w2604, w2598, w2594) -> (resulting string=w2621:string)  [unwired: 2 in, 1 out]
          n1085 = Empty String/Path?(string/path=w2618) -> (empty?=w2622:bool)
          n1086 = case shown="假" w2622 {
            tunnel: [w2646 ""] -> w2620
            tunnel: w2621 -> [w2646 _]
            frame False {
              n1087 = global read "全局 小时数据发送次数.vi" "小时数据发送次数"() -> (w2645:i32)
              n1088 = Increment(x=w2645) -> (x+1=w2644:i32)
              n1089 = global write "全局 小时数据发送次数.vi" "小时数据发送次数"(w2644) -> ()
            }
            frame True {
              n1090 = global read "全局 小时数据发送次数.vi" "小时数据发送次数"() -> (w2648:i32)
              n1091 = Increment(x=w2648) -> (x+1=w2647:i32)
              n1092 = global write "全局 小时数据发送次数.vi" "小时数据发送次数"(w2647) -> ()
            }
          }
        }
        frame "返回执行结果" {
        }
      }
    }
    frame "提取加标回收" {
      # "提取加标回收数据"
      n1093 = global read "全局1.vi" "枚举"() -> (w2657:enum16{"返回请求应答", "上传数据", "返回执行结果"})
      n1094 = case shown="\"上传数据\"" w2657 {
        tunnel: ["QnRtn=1" w2679 "ExeRtn=1"] -> w2651
        tunnel: w2655 -> [_ w2681 _]
        tunnel: w2656 -> [_ w2674 _]
        tunnel: w2654 -> [_ w2671 _]
        tunnel: w2653 -> [_ w2668 _]
        tunnel: w2652 -> [_ w2665 _]
        frame "返回请求应答", Default {
          n1095 = global read "全局 数据数组大小.vi" "数据数组大小"() -> (w2658:i32)
          n1096 = Equal To 0?(x=w2658) -> (x = 0?=w2659:bool)
          n1097 = case shown="真" w2659 {
            frame False {
            }
            frame True {
              n1098 = global read "全局 小时数据发送次数.vi" "小时数据发送次数"() -> (w2662:i32)
              n1099 = Increment(x=w2662) -> (x+1=w2661:i32)
              n1100 = global write "全局 小时数据发送次数.vi" "小时数据发送次数"(w2661) -> ()
            }
          }
        }
        frame "上传数据" {
          # "w01001-Check=63.0,w01001-WaterTime=20160801080000,w01001-Water=45.23,w01001-Chroma=1000,w01001-Volume=0.2,w01001-DVolume=200,w01003-Flag=N;"
          # "总氮"
          # "总磷"
          # "CODMn"
          n1101 = global read "全局 小时数据发送次数.vi" "小时数据发送次数"() -> (w2664:i32)
          n1102 = call "加标回收数据组合 (子VI).vi"("小时数据发送次数"=w2664, "数据"=w2665, "污染物编码"="w01018") -> ("组合输出"=w2663:string)  [unwired: 7 in, 1 out]
          n1103 = call "加标回收数据组合 (子VI).vi"("小时数据发送次数"=w2664, "数据"=w2674, "污染物编码"="w21003") -> ("组合输出"=w2673:string)  [unwired: 7 in, 1 out]
          n1104 = call "加标回收数据组合 (子VI).vi"("小时数据发送次数"=w2664, "数据"=w2668, "污染物编码"="w21001") -> ("组合输出"=w2667:string)  [unwired: 7 in, 1 out]
          n1105 = call "加标回收数据组合 (子VI).vi"("小时数据发送次数"=w2664, "数据"=w2671, "污染物编码"="w21011") -> ("组合输出"=w2670:string)  [unwired: 7 in, 1 out]
          n1106 = call "加标回收数据组合 (子VI).vi"("小时数据发送次数"=w2664, "数据"=w2681, "污染物编码"="w01019") -> ("组合输出"=w2676:string, "datatime"=w2683:string)  [unwired: 7 in]
          n1107 = call "规范时间戳.vi"("字符串"=w2683) -> ("result string"=w2682:string)  [unwired: 10 in]
          n1108 = Empty String/Path?(string/path=w2682) -> (empty?=w2678:bool)
          n1109 = Format Into String(format string="DataTime=%s;%s%s%s%s%s" ("格式字符串"), w2682, w2676, w2673, w2670, w2667, w2663) -> (resulting string=w2680:string)  [unwired: 2 in, 1 out]
          n1110 = case shown="真" w2678 {
            tunnel: [w2687 ""] -> w2679
            tunnel: w2680 -> [w2687 _]
            frame False {
              n1111 = global read "全局 小时数据发送次数.vi" "小时数据发送次数"() -> (w2686:i32)
              n1112 = Increment(x=w2686) -> (x+1=w2685:i32)
              n1113 = global write "全局 小时数据发送次数.vi" "小时数据发送次数"(w2685) -> ()
            }
            frame True {
              n1114 = global read "全局 小时数据发送次数.vi" "小时数据发送次数"() -> (w2689:i32)
              n1115 = Increment(x=w2689) -> (x+1=w2688:i32)
              n1116 = global write "全局 小时数据发送次数.vi" "小时数据发送次数"(w2688) -> ()
            }
          }
        }
        frame "返回执行结果" {
        }
      }
    }
    frame "提取平行样" {
      # "提取平行样数据"
      n1117 = global read "全局1.vi" "枚举"() -> (w2698:enum16{"返回请求应答", "上传数据", "返回执行结果"})
      n1118 = case shown="\"上传数据\"" w2698 {
        tunnel: ["QnRtn=1" w2725 "ExeRtn=1"] -> w2697
        tunnel: w2696 -> [_ w2718 _]
        tunnel: w2695 -> [_ w2716 _]
        tunnel: w2694 -> [_ w2713 _]
        tunnel: w2692 -> [_ w2710 _]
        tunnel: w2693 -> [_ w2706 _]
        frame "返回请求应答", Default {
          n1119 = global read "全局 数据数组大小.vi" "数据数组大小"() -> (w2699:i32)
          n1120 = Equal To 0?(x=w2699) -> (x = 0?=w2700:bool)
          n1121 = case shown="真" w2700 {
            frame False {
            }
            frame True {
              n1122 = global read "全局 小时数据发送次数.vi" "小时数据发送次数"() -> (w2703:i32)
              n1123 = Increment(x=w2703) -> (x+1=w2702:i32)
              n1124 = global write "全局 小时数据发送次数.vi" "小时数据发送次数"(w2702) -> ()
            }
          }
        }
        frame "上传数据" {
          # "CODMn"
          n1125 = global read "全局 小时数据发送次数.vi" "小时数据发送次数"() -> (w2707:i32)
          n1126 = Index Array(array=w2718, index (row)=w2707) -> (element=w2723:string[])  [unwired: 1 in]
          n1127 = Index Array(array=w2723, index=0 ("索引")) -> (element=w2720:string)
          n1128 = call "规范时间戳.vi"("字符串"=w2720) -> ("result string"=w2721:string)  [unwired: 10 in]
          n1129 = call "平行样集成干预数据组合(子VI).vi"("污染物编码"="w01019", "数据输入"=w2718, "小时数据发送次数"=w2707) -> ("输出组合"=w2717:string)  [unwired: 8 in]
          n1130 = call "平行样集成干预数据组合(子VI).vi"("污染物编码"="w21003", "数据输入"=w2716, "小时数据发送次数"=w2707) -> ("输出组合"=w2714:string)  [unwired: 8 in]
          n1131 = call "平行样集成干预数据组合(子VI).vi"("污染物编码"="w21011", "数据输入"=w2713, "小时数据发送次数"=w2707) -> ("输出组合"=w2711:string)  [unwired: 8 in]
          n1132 = call "平行样集成干预数据组合(子VI).vi"("污染物编码"="w21001", "数据输入"=w2710, "小时数据发送次数"=w2707) -> ("输出组合"=w2708:string)  [unwired: 8 in]
          n1133 = call "平行样集成干预数据组合(子VI).vi"("污染物编码"="w01018", "数据输入"=w2706, "小时数据发送次数"=w2707) -> ("输出组合"=w2704:string)  [unwired: 8 in]
          n1134 = Empty String/Path?(string/path=w2720) -> (empty?=w2724:bool)
          n1135 = Format Into String(format string="DataTime=%s;%s%s%s%s%s" ("格式字符串"), w2721, w2717, w2714, w2711, w2708, w2704) -> (resulting string=w2726:string)  [unwired: 2 in, 1 out]
          n1136 = case shown="真" w2724 {
            tunnel: [w2730 ""] -> w2725
            tunnel: w2726 -> [w2730 _]
            frame False {
              n1137 = global read "全局 小时数据发送次数.vi" "小时数据发送次数"() -> (w2729:i32)
              n1138 = Increment(x=w2729) -> (x+1=w2728:i32)
              n1139 = global write "全局 小时数据发送次数.vi" "小时数据发送次数"(w2728) -> ()
            }
            frame True {
              n1140 = global read "全局 小时数据发送次数.vi" "小时数据发送次数"() -> (w2732:i32)
              n1141 = Increment(x=w2732) -> (x+1=w2731:i32)
              n1142 = global write "全局 小时数据发送次数.vi" "小时数据发送次数"(w2731) -> ()
            }
          }
        }
        frame "返回执行结果" {
        }
      }
    }
    frame "提取集成干预" {
      # "提取平行样数据"
      n1143 = global read "全局1.vi" "枚举"() -> (w2746:enum16{"返回请求应答", "上传数据", "返回执行结果"})
      n1144 = case shown="\"上传数据\"" w2746 {
        tunnel: ["QnRtn=1" w2788 "ExeRtn=1"] -> w2745
        tunnel: w2744 -> [_ w2754 _]
        tunnel: w2743 -> [_ w2760 _]
        tunnel: w2737 -> [_ w2763 _]
        tunnel: w2738 -> [_ w2766 _]
        tunnel: w2739 -> [_ w2770 _]
        tunnel: w2736 -> [_ w2772 _]
        tunnel: w2735 -> [_ w2775 _]
        tunnel: w2740 -> [_ w2778 _]
        tunnel: w2742 -> [_ w2782 _]
        tunnel: w2741 -> [_ w2784 _]
        frame "返回请求应答", Default {
          n1145 = global read "全局 数据数组大小.vi" "数据数组大小"() -> (w2747:i32)
          n1146 = Equal To 0?(x=w2747) -> (x = 0?=w2748:bool)
          n1147 = case shown="真" w2748 {
            frame False {
            }
            frame True {
              n1148 = global read "全局 小时数据发送次数.vi" "小时数据发送次数"() -> (w2751:i32)
              n1149 = Increment(x=w2751) -> (x+1=w2750:i32)
              n1150 = global write "全局 小时数据发送次数.vi" "小时数据发送次数"(w2750) -> ()
            }
          }
        }
        frame "上传数据" {
          # "CODMn"
          n1151 = global read "全局 小时数据发送次数.vi" "小时数据发送次数"() -> (w2755:i32)
          n1152 = Index Array(array=w2754, index (row)=w2755) -> (element=w2758:string[])  [unwired: 1 in]
          n1153 = Index Array(array=w2758, index=0 ("索引")) -> (element=w2756:string)
          n1154 = call "规范时间戳.vi"("字符串"=w2756) -> ("result string"=w2786:string)  [unwired: 10 in]
          n1155 = call "平行样集成干预数据组合(子VI).vi"("污染物编码"="w21001", "数据输入"=w2782, "小时数据发送次数"=w2755) -> ("输出组合"=w2780:string)  [unwired: 8 in]
          n1156 = call "平行样集成干预数据组合(子VI).vi"("污染物编码"="w21011", "数据输入"=w2778, "小时数据发送次数"=w2755) -> ("输出组合"=w2777:string)  [unwired: 8 in]
          n1157 = call "平行样集成干预数据组合(子VI).vi"("污染物编码"="w01014", "数据输入"=w2772, "小时数据发送次数"=w2755) -> ("输出组合"=w2771:string)  [unwired: 8 in]
          n1158 = call "平行样集成干预数据组合(子VI).vi"("污染物编码"="w01019", "数据输入"=w2754, "小时数据发送次数"=w2755) -> ("输出组合"=w2752:string)  [unwired: 8 in]
          n1159 = call "平行样集成干预数据组合(子VI).vi"("污染物编码"="w01009", "数据输入"=w2770, "小时数据发送次数"=w2755) -> ("输出组合"=w2768:string)  [unwired: 8 in]
          n1160 = call "平行样集成干预数据组合(子VI).vi"("污染物编码"="w01001", "数据输入"=w2766, "小时数据发送次数"=w2755) -> ("输出组合"=w2765:string)  [unwired: 8 in]
          n1161 = call "平行样集成干预数据组合(子VI).vi"("污染物编码"="w21003", "数据输入"=w2760, "小时数据发送次数"=w2755) -> ("输出组合"=w2759:string)  [unwired: 8 in]
          n1162 = call "平行样集成干预数据组合(子VI).vi"("污染物编码"="w01010", "数据输入"=w2763, "小时数据发送次数"=w2755) -> ("输出组合"=w2762:string)  [unwired: 8 in]
          n1163 = call "平行样集成干预数据组合(子VI).vi"("污染物编码"="w01003", "数据输入"=w2775, "小时数据发送次数"=w2755) -> ("输出组合"=w2774:string)  [unwired: 8 in]
          n1164 = call "平行样集成干预数据组合(子VI).vi"("污染物编码"="w01018", "数据输入"=w2784, "小时数据发送次数"=w2755) -> ("输出组合"=w2785:string)  [unwired: 8 in]
          n1165 = Empty String/Path?(string/path=w2756) -> (empty?=w2787:bool)
          n1166 = Format Into String(format string="DataTime=%s;%s%s%s%s%s%s%s%s%s%s" ("格式字符串"), w2786, w2752, w2759, w2762, w2765, w2768, w2771, w2774, w2777, w2780, w2785) -> (resulting string=w2789:string)  [unwired: 2 in, 1 out]
          n1167 = case shown="真" w2787 {
            tunnel: [w2793 ""] -> w2788
            tunnel: w2789 -> [w2793 _]
            frame False {
              n1168 = global read "全局 小时数据发送次数.vi" "小时数据发送次数"() -> (w2792:i32)
              n1169 = Increment(x=w2792) -> (x+1=w2791:i32)
              n1170 = global write "全局 小时数据发送次数.vi" "小时数据发送次数"(w2791) -> ()
            }
            frame True {
              n1171 = global read "全局 小时数据发送次数.vi" "小时数据发送次数"() -> (w2795:i32)
              n1172 = Increment(x=w2795) -> (x+1=w2794:i32)
              n1173 = global write "全局 小时数据发送次数.vi" "小时数据发送次数"(w2794) -> ()
            }
          }
        }
        frame "返回执行结果" {
        }
      }
    }
    frame "操作日志" {
      n1174 = global read "全局 小时数据发送次数.vi" "小时数据发送次数"() -> (w2808:i32)
      n1175 = global read "全局 小时数据发送次数.vi" "小时数据发送次数"() -> (w2810:i32)
      n1176 = global read "全局 小时数据发送次数.vi" "小时数据发送次数"() -> (w2806:i32)
      n1177 = global read "全局 小时数据发送次数.vi" "小时数据发送次数"() -> (w2805:i32)
      n1178 = global read "全局 小时数据发送次数.vi" "小时数据发送次数"() -> (w2800:i32)
      n1179 = global read "全局 小时数据发送次数.vi" "小时数据发送次数"() -> (w2802:i32)
      n1180 = Index Array(array=w2816, index (row)=w2808) -> (element=w2807:string[])  [unwired: 1 in]
      n1181 = Index Array(array=w2815, index (row)=w2810) -> (element=w2809:string[])  [unwired: 1 in]
      n1182 = Index Array(array=w2813, index (row)=w2806) -> (element=w2804:string[])  [unwired: 1 in]
      n1183 = Index Array(array=w2812, index (row)=w2805) -> (element=w2803:string[])  [unwired: 1 in]
      n1184 = Index Array(array=w2799, index (row)=w2800) -> (element=w2798:string[])  [unwired: 1 in]
      n1185 = global read "全局1.vi" "枚举"() -> (w2811:enum16{"返回请求应答", "上传数据", "返回执行结果"})
      n1186 = Index Array(array=w2814, index (row)=w2802) -> (element=w2801:string[])  [unwired: 1 in]
      n1187 = case shown="\"上传数据\"" w2811 {
        tunnel: ["QnRtn=1" w2838 "ExeRtn=1"] -> w2817
        tunnel: w2809 -> [_ w2857 _]
        tunnel: w2807 -> [_ w2855 _]
        tunnel: w2804 -> [_ w2854 _]
        tunnel: w2803 -> [_ w2853 _]
        tunnel: w2801 -> [_ w2851 _]
        tunnel: w2798 -> [_ w2824 _]
        frame "返回请求应答", Default {
          n1188 = global read "全局 数据数组大小.vi" "数据数组大小"() -> (w2820:i32)
          n1189 = Equal To 0?(x=w2820) -> (x = 0?=w2819:bool)
          n1190 = case shown="真" w2819 {
            frame False {
            }
            frame True {
              n1191 = global read "全局 小时数据发送次数.vi" "小时数据发送次数"() -> (w2822:i32)
              n1192 = Increment(x=w2822) -> (x+1=w2821:i32)
              n1193 = global write "全局 小时数据发送次数.vi" "小时数据发送次数"(w2821) -> ()
            }
          }
        }
        frame "上传数据" {
          n1194 = Index Array(array=w2824, index #1=0 ("索引"), index #2=2 ("索引")) -> (element #1=w2827:string, element #2=w2829:string)
          n1195 = Index Array(array=w2853, index #1=0 ("索引"), index #2=2 ("索引")) -> (element #1=w2852:string, element #2=w2842:string)
          n1196 = Index Array(array=w2857, index #1=0 ("索引"), index #2=2 ("索引")) -> (element #1=w2856:string, element #2=w2844:string)
          n1197 = Index Array(array=w2851, index #1=0 ("索引"), index #2=2 ("索引")) -> (element #1=w2850:string, element #2=w2846:string)
          n1198 = Index Array(array=w2854, index #1=0 ("索引"), index #2=2 ("索引")) -> (element #1=w2858:string, element #2=w2840:string)
          n1199 = Index Array(array=w2855, index #1=0 ("索引"), index #2=2 ("索引")) -> (element #1=w2833:string, element #2=w2849:string)
          n1200 = Empty String/Path?(string/path=w2829) -> (empty?=w2828:bool)
          n1201 = Empty String/Path?(string/path=w2842) -> (empty?=w2843:bool)
          n1202 = Empty String/Path?(string/path=w2844) -> (empty?=w2845:bool)
          n1203 = Empty String/Path?(string/path=w2840) -> (empty?=w2841:bool)
          n1204 = case shown="假" w2845 {
            tunnel: [w2893 ""] -> w2870
            tunnel: w2844 -> [w2892 _]
            tunnel: w2856 -> [_ _]
            frame False {
              # "氨氮"
              n1205 = Format Into String(format string="PolId=w21003,i11001-Info=//%s//;" ("格式字符串"), w2892) -> (resulting string=w2893:string)  [unwired: 2 in, 1 out]
            }
            frame True {
            }
          }
          n1206 = case shown="假" w2828 {
            tunnel: [w2874 ""] -> w2823
            tunnel: w2827 -> [_ _]
            tunnel: w2829 -> [w2875 _]
            frame False {
              # "CODCr"
              n1207 = Format Into String(format string="PolId=w01018,i11001-Info=//%s//;" ("格式字符串"), w2875) -> (resulting string=w2874:string)  [unwired: 2 in, 1 out]
            }
            frame True {
            }
          }
          n1208 = case shown="假" w2843 {
            tunnel: [w2888 ""] -> w2865
            tunnel: w2852 -> [_ _]
            tunnel: w2842 -> [w2889 _]
            frame False {
              # "总氮"
              n1209 = Format Into String(format string="PolId=w21001,i11001-Info=//%s//;" ("格式字符串"), w2889) -> (resulting string=w2888:string)  [unwired: 2 in, 1 out]
            }
            frame True {
            }
          }
          n1210 = Empty String/Path?(string/path=w2846) -> (empty?=w2847:bool)
          n1211 = case shown="假" w2841 {
            tunnel: [w2886 ""] -> w2866
            tunnel: w2858 -> [_ _]
            tunnel: w2840 -> [w2884 _]
            frame False {
              # "总磷"
              n1212 = Format Into String(format string="PolId=w21011,i11001-Info=//%s//;" ("格式字符串"), w2884) -> (resulting string=w2886:string)  [unwired: 2 in, 1 out]
            }
            frame True {
            }
          }
          n1213 = case shown="假" w2847 {
            tunnel: [w2898 ""] -> w2869
            tunnel: w2850 -> [_ _]
            tunnel: w2846 -> [w2896 _]
            frame False {
              # "系统日志"
              n1214 = Format Into String(format string="PolId=w00000,i21001-Info=//%s//;" ("格式字符串"), w2896) -> (resulting string=w2898:string)  [unwired: 2 in, 1 out]
            }
            frame True {
            }
          }
          n1215 = Empty String/Path?(string/path=w2849) -> (empty?=w2848:bool)
          n1216 = case shown="假" w2848 {
            tunnel: [w2901 ""] -> w2871
            tunnel: w2833 -> [_ _]
            tunnel: w2849 -> [w2900 _]
            frame False {
              # "高锰酸钾盐"
              n1217 = Format Into String(format string="PolId=w01019,i11001-Info=//%s//;" ("格式字符串"), w2900) -> (resulting string=w2901:string)  [unwired: 2 in, 1 out]
            }
            frame True {
            }
          }
          n1218 = call "规范时间戳.vi"("字符串"=w2833) -> ("result string"=w2831:string)  [unwired: 10 in]
          n1219 = Format Into String(format string="DataTime=%s;", w2831) -> (resulting string=w2830:string)  [unwired: 2 in, 1 out]
          n1220 = Concatenate Strings(w2830, w2871, w2870, w2869, w2866, w2865, w2823) -> (w2835:string)
          n1221 = String Length(string=w2835) -> (length=w2837:i32)
          n1222 = Empty String/Path?(string/path=w2835) -> (empty?=w2839:bool)
          n1223 = Decrement(x=w2837) -> (x-1=w2836:i32)
          n1224 = String Subset(string=w2835, length (rest)=w2836) -> (substring=w2834:string)  [unwired: 1 in]
          n1225 = case shown="假" w2839 {
            tunnel: [w2880 ""] -> w2838
            tunnel: w2834 -> [w2880 _]
            frame False {
              n1226 = global read "全局 小时数据发送次数.vi" "小时数据发送次数"() -> (w2879:i32)
              n1227 = Increment(x=w2879) -> (x+1=w2878:i32)
              n1228 = global write "全局 小时数据发送次数.vi" "小时数据发送次数"(w2878) -> ()
            }
            frame True {
              n1229 = global read "全局 小时数据发送次数.vi" "小时数据发送次数"() -> (w2882:i32)
              n1230 = Increment(x=w2882) -> (x+1=w2881:i32)
              n1231 = global write "全局 小时数据发送次数.vi" "小时数据发送次数"(w2881) -> ()
            }
          }
        }
        frame "返回执行结果" {
        }
      }
    }
    frame "仪器参数" {
      n1232 = global read "全局 小时数据发送次数.vi" "小时数据发送次数"() -> (w2936:i32)
      n1233 = global read "全局 小时数据发送次数.vi" "小时数据发送次数"() -> (w2938:i32)
      n1234 = global read "全局 小时数据发送次数.vi" "小时数据发送次数"() -> (w2934:i32)
      n1235 = global read "全局 小时数据发送次数.vi" "小时数据发送次数"() -> (w2919:i32)
      n1236 = global read "全局 小时数据发送次数.vi" "小时数据发送次数"() -> (w2913:i32)
      n1237 = global read "全局 小时数据发送次数.vi" "小时数据发送次数"() -> (w2915:i32)
      n1238 = global read "全局 小时数据发送次数.vi" "小时数据发送次数"() -> (w2914:i32)
      n1239 = global read "全局 小时数据发送次数.vi" "小时数据发送次数"() -> (w2930:i32)
      n1240 = global read "全局 小时数据发送次数.vi" "小时数据发送次数"() -> (w2916:i32)
      n1241 = global read "全局 小时数据发送次数.vi" "小时数据发送次数"() -> (w2925:i32)
      n1242 = global read "全局 小时数据发送次数.vi" "小时数据发送次数"() -> (w2933:i32)
      n1243 = global read "全局 小时数据发送次数.vi" "小时数据发送次数"() -> (w2929:i32)
      n1244 = global read "全局 小时数据发送次数.vi" "小时数据发送次数"() -> (w2922:i32)
      n1245 = Index Array(array=w2944, index (row)=w2936) -> (element=w2935:string[])  [unwired: 1 in]
      n1246 = Index Array(array=w2943, index (row)=w2938) -> (element=w2937:string[])  [unwired: 1 in]
      n1247 = Index Array(array=w2918, index (row)=w2919) -> (element=w2917:string[])  [unwired: 1 in]
      n1248 = Index Array(array=w2906, index (row)=w2913) -> (element=w2905:string[])  [unwired: 1 in]
      n1249 = Index Array(array=w2910, index (row)=w2915) -> (element=w2909:string[])  [unwired: 1 in]
      n1250 = Index Array(array=w2908, index (row)=w2914) -> (element=w2907:string[])  [unwired: 1 in]
      n1251 = Index Array(array=w2942, index (row)=w2930) -> (element=w2926:string[])  [unwired: 1 in]
      n1252 = Index Array(array=w2941, index (row)=w2934) -> (element=w2932:string[])  [unwired: 1 in]
      n1253 = Index Array(array=w2912, index (row)=w2916) -> (element=w2911:string[])  [unwired: 1 in]
      n1254 = Index Array(array=w2924, index (row)=w2925) -> (element=w2923:string[])  [unwired: 1 in]
      n1255 = Index Array(array=w2940, index (row)=w2933) -> (element=w2931:string[])  [unwired: 1 in]
      n1256 = Index Array(array=w2928, index (row)=w2929) -> (element=w2927:string[])  [unwired: 1 in]
      n1257 = Index Array(array=w2921, index (row)=w2922) -> (element=w2920:string[])  [unwired: 1 in]
      n1258 = global read "全局1.vi" "枚举"() -> (w2939:enum16{"返回请求应答", "上传数据", "返回执行结果"})
      n1259 = case shown="\"上传数据\"" w2939 {
        tunnel: ["QnRtn=1" w3010 "ExeRtn=1"] -> w2945
        tunnel: w2937 -> [_ w2973 _]
        tunnel: w2935 -> [_ w2970 _]
        tunnel: w2932 -> [_ w2976 _]
        tunnel: w2931 -> [_ w2979 _]
        tunnel: w2927 -> [_ w2982 _]
        tunnel: w2926 -> [_ w3007 _]
        tunnel: w2923 -> [_ w3003 _]
        tunnel: w2920 -> [_ w3001 _]
        tunnel: w2917 -> [_ w2999 _]
        tunnel: w2911 -> [_ w2997 _]
        tunnel: w2909 -> [_ w2995 _]
        tunnel: w2907 -> [_ w2993 _]
        tunnel: w2905 -> [_ w2991 _]
        frame "返回请求应答", Default {
          n1260 = global read "全局 数据数组大小.vi" "数据数组大小"() -> (w2948:i32)
          n1261 = Equal To 0?(x=w2948) -> (x = 0?=w2947:bool)
          n1262 = case shown="真" w2947 {
            frame False {
            }
            frame True {
              n1263 = global read "全局 小时数据发送次数.vi" "小时数据发送次数"() -> (w2950:i32)
              n1264 = Increment(x=w2950) -> (x+1=w2949:i32)
              n1265 = global write "全局 小时数据发送次数.vi" "小时数据发送次数"(w2949) -> ()
            }
          }
        }
        frame "上传数据" {
          n1266 = call "关键参数组合 (子VI).vi"("table"="仪器参数", "因子编码"="w21001", "DO"=w2979) -> ("字符串"=w2978:string)  [unwired: 8 in]
          n1267 = call "关键参数组合 (子VI).vi"("table"="仪器参数", "因子编码"="w01001", "DO"=w3003) -> ("字符串"=w2990:string)  [unwired: 8 in]
          n1268 = call "关键参数组合 (子VI).vi"("table"="仪器参数", "因子编码"="w01019", "DO"=w2970) -> ("字符串"=w2968:string)  [unwired: 8 in]
          n1269 = call "关键参数组合 (子VI).vi"("table"="仪器参数", "因子编码"="w01014", "DO"=w3001) -> ("字符串"=w2989:string)  [unwired: 8 in]
          n1270 = call "关键参数组合 (子VI).vi"("table"="仪器参数", "因子编码"="w01003", "DO"=w2997) -> ("字符串"=w2987:string)  [unwired: 8 in]
          n1271 = call "关键参数组合 (子VI).vi"("table"="仪器参数", "因子编码"="w01010", "DO"=w2999) -> ("字符串"=w2988:string)  [unwired: 8 in]
          n1272 = call "关键参数组合 (子VI).vi"("table"="仪器参数", "因子编码"="w01018", "DO"=w2982) -> ("字符串"=w2981:string)  [unwired: 8 in]
          n1273 = call "关键参数组合 (子VI).vi"("table"="仪器参数", "因子编码"="w01009", "DO"=w3007) -> ("字符串"=w3006:string)  [unwired: 8 in]
          n1274 = call "关键参数组合 (子VI).vi"("table"="仪器参数", "因子编码"="w21011", "DO"=w2976) -> ("字符串"=w2975:string)  [unwired: 8 in]
          n1275 = call "关键参数组合 (子VI).vi"("table"="仪器参数", "因子编码"="w01016", "DO"=w2995) -> ("字符串"=w2986:string)  [unwired: 8 in]
          n1276 = call "关键参数组合 (子VI).vi"("table"="仪器参数", "因子编码"="w21003", "DO"=w2973) -> ("字符串"=w2972:string)  [unwired: 8 in]
          n1277 = call "关键参数组合 (子VI).vi"("table"="仪器参数", "因子编码"="w01100", "DO"=w2991) -> ("字符串"=w2984:string)  [unwired: 8 in]
          n1278 = call "关键参数组合 (子VI).vi"("table"="仪器参数", "因子编码"="w19011", "DO"=w2993) -> ("字符串"=w2985:string)  [unwired: 8 in]
          n1279 = Index Array(array=w2970) -> (element=w2969:string)  [unwired: 1 in]
          n1280 = call "规范时间戳.vi"("字符串"=w2969) -> ("result string"=w3008:string)  [unwired: 10 in]
          n1281 = Format Into String(format string="DataTime=%s;%s%s%s%s%s%s%s%s%s%s%s%s%s" ("格式字符串"), w3008, w2968, w2972, w2975, w2978, w2981, w3006, w2990, w2989, w2988, w2987, w2986, w2985, w2984) -> (resulting string=w2952:string)  [unwired: 2 in, 1 out]
          n1282 = String Length(string=w2952) -> (length=w2953:i32)
          n1283 = Decrement(x=w2953) -> (x-1=w2954:i32)
          n1284 = String Subset(string=w2952, length (rest)=w2954) -> (substring=w2951:string)  [unwired: 1 in]
          n1285 = Empty String/Path?(string/path=w2951) -> (empty?=w3011:bool)
          n1286 = case shown="假" w3011 {
            tunnel: [w3014 ""] -> w3010
            tunnel: w2951 -> [w3014 _]
            frame False {
              n1287 = global read "全局 小时数据发送次数.vi" "小时数据发送次数"() -> (w3013:i32)
              n1288 = Increment(x=w3013) -> (x+1=w3012:i32)
              n1289 = global write "全局 小时数据发送次数.vi" "小时数据发送次数"(w3012) -> ()
            }
            frame True {
              n1290 = global read "全局 小时数据发送次数.vi" "小时数据发送次数"() -> (w3016:i32)
              n1291 = Increment(x=w3016) -> (x+1=w3015:i32)
              n1292 = global write "全局 小时数据发送次数.vi" "小时数据发送次数"(w3015) -> ()
            }
          }
        }
        frame "返回执行结果" {
        }
      }
    }
    frame "3090仪器参数" {
      n1293 = global read "全局 小时数据发送次数.vi" "小时数据发送次数"() -> (w3050:i32)
      n1294 = global read "全局 小时数据发送次数.vi" "小时数据发送次数"() -> (w3052:i32)
      n1295 = global read "全局 小时数据发送次数.vi" "小时数据发送次数"() -> (w3048:i32)
      n1296 = global read "全局 小时数据发送次数.vi" "小时数据发送次数"() -> (w3033:i32)
      n1297 = global read "全局 小时数据发送次数.vi" "小时数据发送次数"() -> (w3027:i32)
      n1298 = global read "全局 小时数据发送次数.vi" "小时数据发送次数"() -> (w3029:i32)
      n1299 = global read "全局 小时数据发送次数.vi" "小时数据发送次数"() -> (w3028:i32)
      n1300 = global read "全局 小时数据发送次数.vi" "小时数据发送次数"() -> (w3044:i32)
      n1301 = global read "全局 小时数据发送次数.vi" "小时数据发送次数"() -> (w3030:i32)
      n1302 = global read "全局 小时数据发送次数.vi" "小时数据发送次数"() -> (w3039:i32)
      n1303 = global read "全局 小时数据发送次数.vi" "小时数据发送次数"() -> (w3047:i32)
      n1304 = global read "全局 小时数据发送次数.vi" "小时数据发送次数"() -> (w3043:i32)
      n1305 = global read "全局 小时数据发送次数.vi" "小时数据发送次数"() -> (w3036:i32)
      n1306 = Index Array(array=w3058, index (row)=w3050) -> (element=w3049:string[])  [unwired: 1 in]
      n1307 = Index Array(array=w3057, index (row)=w3052) -> (element=w3051:string[])  [unwired: 1 in]
      n1308 = Index Array(array=w3032, index (row)=w3033) -> (element=w3031:string[])  [unwired: 1 in]
      n1309 = Index Array(array=w3020, index (row)=w3027) -> (element=w3019:string[])  [unwired: 1 in]
      n1310 = Index Array(array=w3024, index (row)=w3029) -> (element=w3023:string[])  [unwired: 1 in]
      n1311 = Index Array(array=w3022, index (row)=w3028) -> (element=w3021:string[])  [unwired: 1 in]
      n1312 = Index Array(array=w3056, index (row)=w3044) -> (element=w3040:string[])  [unwired: 1 in]
      n1313 = Index Array(array=w3055, index (row)=w3048) -> (element=w3046:string[])  [unwired: 1 in]
      n1314 = Index Array(array=w3026, index (row)=w3030) -> (element=w3025:string[])  [unwired: 1 in]
      n1315 = Index Array(array=w3038, index (row)=w3039) -> (element=w3037:string[])  [unwired: 1 in]
      n1316 = Index Array(array=w3054, index (row)=w3047) -> (element=w3045:string[])  [unwired: 1 in]
      n1317 = Index Array(array=w3042, index (row)=w3043) -> (element=w3041:string[])  [unwired: 1 in]
      n1318 = Index Array(array=w3035, index (row)=w3036) -> (element=w3034:string[])  [unwired: 1 in]
      n1319 = global read "全局1.vi" "枚举"() -> (w3053:enum16{"返回请求应答", "上传数据", "返回执行结果"})
      n1320 = case shown="\"上传数据\"" w3053 {
        tunnel: ["QnRtn=1" w3124 "ExeRtn=1"] -> w3059
        tunnel: w3051 -> [_ w3087 _]
        tunnel: w3049 -> [_ w3084 _]
        tunnel: w3046 -> [_ w3090 _]
        tunnel: w3045 -> [_ w3093 _]
        tunnel: w3041 -> [_ w3096 _]
        tunnel: w3040 -> [_ w3121 _]
        tunnel: w3037 -> [_ w3117 _]
        tunnel: w3034 -> [_ w3115 _]
        tunnel: w3031 -> [_ w3113 _]
        tunnel: w3025 -> [_ w3111 _]
        tunnel: w3023 -> [_ w3109 _]
        tunnel: w3021 -> [_ w3107 _]
        tunnel: w3019 -> [_ w3105 _]
        frame "返回请求应答", Default {
          n1321 = global read "全局 数据数组大小.vi" "数据数组大小"() -> (w3062:i32)
          n1322 = Equal To 0?(x=w3062) -> (x = 0?=w3061:bool)
          n1323 = case shown="真" w3061 {
            frame False {
            }
            frame True {
              n1324 = global read "全局 小时数据发送次数.vi" "小时数据发送次数"() -> (w3064:i32)
              n1325 = Increment(x=w3064) -> (x+1=w3063:i32)
              n1326 = global write "全局 小时数据发送次数.vi" "小时数据发送次数"(w3063) -> ()
            }
          }
        }
        frame "上传数据" {
          n1327 = call "关键参数组合 (子VI).vi"("table"="3090仪器参数", "因子编码"="w21001", "DO"=w3093) -> ("字符串"=w3092:string)  [unwired: 8 in]
          n1328 = call "关键参数组合 (子VI).vi"("table"="3090仪器参数", "因子编码"="w01001", "DO"=w3117) -> ("字符串"=w3104:string)  [unwired: 8 in]
          n1329 = call "关键参数组合 (子VI).vi"("table"="3090仪器参数", "因子编码"="w01019", "DO"=w3084) -> ("字符串"=w3082:string)  [unwired: 8 in]
          n1330 = call "关键参数组合 (子VI).vi"("table"="3090仪器参数", "因子编码"="w01014", "DO"=w3115) -> ("字符串"=w3103:string)  [unwired: 8 in]
          n1331 = call "关键参数组合 (子VI).vi"("table"="3090仪器参数", "因子编码"="w01003", "DO"=w3111) -> ("字符串"=w3101:string)  [unwired: 8 in]
          n1332 = call "关键参数组合 (子VI).vi"("table"="3090仪器参数", "因子编码"="w01010", "DO"=w3113) -> ("字符串"=w3102:string)  [unwired: 8 in]
          n1333 = call "关键参数组合 (子VI).vi"("table"="3090仪器参数", "因子编码"="w01018", "DO"=w3096) -> ("字符串"=w3095:string)  [unwired: 8 in]
          n1334 = call "关键参数组合 (子VI).vi"("table"="3090仪器参数", "因子编码"="w01009", "DO"=w3121) -> ("字符串"=w3120:string)  [unwired: 8 in]
          n1335 = call "关键参数组合 (子VI).vi"("table"="3090仪器参数", "因子编码"="w21011", "DO"=w3090) -> ("字符串"=w3089:string)  [unwired: 8 in]
          n1336 = call "关键参数组合 (子VI).vi"("table"="3090仪器参数", "因子编码"="w01016", "DO"=w3109) -> ("字符串"=w3100:string)  [unwired: 8 in]
          n1337 = call "关键参数组合 (子VI).vi"("table"="3090仪器参数", "因子编码"="w21003", "DO"=w3087) -> ("字符串"=w3086:string)  [unwired: 8 in]
          n1338 = call "关键参数组合 (子VI).vi"("table"="3090仪器参数", "因子编码"="w01100", "DO"=w3105) -> ("字符串"=w3098:string)  [unwired: 8 in]
          n1339 = call "关键参数组合 (子VI).vi"("table"="3090仪器参数", "因子编码"="w19011", "DO"=w3107) -> ("字符串"=w3099:string)  [unwired: 8 in]
          n1340 = Index Array(array=w3084) -> (element=w3083:string)  [unwired: 1 in]
          n1341 = call "规范时间戳.vi"("字符串"=w3083) -> ("result string"=w3122:string)  [unwired: 10 in]
          n1342 = Format Into String(format string="DataTime=%s;%s%s%s%s%s%s%s%s%s%s%s%s%s" ("格式字符串"), w3122, w3082, w3086, w3089, w3092, w3095, w3120, w3104, w3103, w3102, w3101, w3100, w3099, w3098) -> (resulting string=w3066:string)  [unwired: 2 in, 1 out]
          n1343 = String Length(string=w3066) -> (length=w3067:i32)
          n1344 = Decrement(x=w3067) -> (x-1=w3068:i32)
          n1345 = String Subset(string=w3066, length (rest)=w3068) -> (substring=w3065:string)  [unwired: 1 in]
          n1346 = Empty String/Path?(string/path=w3065) -> (empty?=w3125:bool)
          n1347 = case shown="假" w3125 {
            tunnel: [w3128 ""] -> w3124
            tunnel: w3065 -> [w3128 _]
            frame False {
              n1348 = global read "全局 小时数据发送次数.vi" "小时数据发送次数"() -> (w3127:i32)
              n1349 = Increment(x=w3127) -> (x+1=w3126:i32)
              n1350 = global write "全局 小时数据发送次数.vi" "小时数据发送次数"(w3126) -> ()
            }
            frame True {
              n1351 = global read "全局 小时数据发送次数.vi" "小时数据发送次数"() -> (w3130:i32)
              n1352 = Increment(x=w3130) -> (x+1=w3129:i32)
              n1353 = global write "全局 小时数据发送次数.vi" "小时数据发送次数"(w3129) -> ()
            }
          }
        }
        frame "返回执行结果" {
        }
      }
    }
    frame "提取仪器参数" {
      n1354 = global read "全局 小时数据发送次数.vi" "小时数据发送次数"() -> (w3164:i32)
      n1355 = global read "全局 小时数据发送次数.vi" "小时数据发送次数"() -> (w3166:i32)
      n1356 = global read "全局 小时数据发送次数.vi" "小时数据发送次数"() -> (w3147:i32)
      n1357 = global read "全局 小时数据发送次数.vi" "小时数据发送次数"() -> (w3150:i32)
      n1358 = global read "全局 小时数据发送次数.vi" "小时数据发送次数"() -> (w3149:i32)
      n1359 = global read "全局 小时数据发送次数.vi" "小时数据发送次数"() -> (w3148:i32)
      n1360 = global read "全局 小时数据发送次数.vi" "小时数据发送次数"() -> (w3158:i32)
      n1361 = global read "全局 小时数据发送次数.vi" "小时数据发送次数"() -> (w3152:i32)
      n1362 = global read "全局 小时数据发送次数.vi" "小时数据发送次数"() -> (w3153:i32)
      n1363 = global read "全局 小时数据发送次数.vi" "小时数据发送次数"() -> (w3151:i32)
      n1364 = global read "全局 小时数据发送次数.vi" "小时数据发送次数"() -> (w3162:i32)
      n1365 = global read "全局 小时数据发送次数.vi" "小时数据发送次数"() -> (w3157:i32)
      n1366 = global read "全局 小时数据发送次数.vi" "小时数据发送次数"() -> (w3161:i32)
      n1367 = Index Array(array=w3136, index (row)=w3147) -> (element=w3133:string[])  [unwired: 1 in]
      n1368 = Index Array(array=w3140, index (row)=w3150) -> (element=w3139:string[])  [unwired: 1 in]
      n1369 = Index Array(array=w3138, index (row)=w3149) -> (element=w3135:string[])  [unwired: 1 in]
      n1370 = Index Array(array=w3137, index (row)=w3148) -> (element=w3134:string[])  [unwired: 1 in]
      n1371 = Index Array(array=w3170, index (row)=w3158) -> (element=w3154:string[])  [unwired: 1 in]
      n1372 = Index Array(array=w3145, index (row)=w3152) -> (element=w3142:string[])  [unwired: 1 in]
      n1373 = Index Array(array=w3172, index (row)=w3164) -> (element=w3163:string[])  [unwired: 1 in]
      n1374 = Index Array(array=w3146, index (row)=w3153) -> (element=w3143:string[])  [unwired: 1 in]
      n1375 = Index Array(array=w3144, index (row)=w3151) -> (element=w3141:string[])  [unwired: 1 in]
      n1376 = Index Array(array=w3171, index (row)=w3166) -> (element=w3165:string[])  [unwired: 1 in]
      n1377 = Index Array(array=w3169, index (row)=w3162) -> (element=w3160:string[])  [unwired: 1 in]
      n1378 = Index Array(array=w3156, index (row)=w3157) -> (element=w3155:string[])  [unwired: 1 in]
      n1379 = Index Array(array=w3168, index (row)=w3161) -> (element=w3159:string[])  [unwired: 1 in]
      n1380 = global read "全局1.vi" "枚举"() -> (w3167:enum16{"返回请求应答", "上传数据", "返回执行结果"})
      n1381 = case shown="\"上传数据\"" w3167 {
        tunnel: ["QnRtn=1" w3219 "ExeRtn=1"] -> w3173
        tunnel: w3165 -> [_ w3186 _]
        tunnel: w3163 -> [_ w3180 _]
        tunnel: w3160 -> [_ w3190 _]
        tunnel: w3159 -> [_ w3218 _]
        tunnel: w3155 -> [_ w3183 _]
        tunnel: w3154 -> [_ w3214 _]
        tunnel: w3143 -> [_ w3206 _]
        tunnel: w3142 -> [_ w3205 _]
        tunnel: w3141 -> [_ w3204 _]
        tunnel: w3139 -> [_ w3203 _]
        tunnel: w3135 -> [_ w3202 _]
        tunnel: w3134 -> [_ w3201 _]
        tunnel: w3133 -> [_ w3200 _]
        frame "返回请求应答", Default {
          n1382 = global read "全局 数据数组大小.vi" "数据数组大小"() -> (w3176:i32)
          n1383 = Equal To 0?(x=w3176) -> (x = 0?=w3175:bool)
          n1384 = case shown="假" w3175 {
            frame False {
            }
            frame True {
              n1385 = global read "全局 小时数据发送次数.vi" "小时数据发送次数"() -> (w3178:i32)
              n1386 = Increment(x=w3178) -> (x+1=w3177:i32)
              n1387 = global write "全局 小时数据发送次数.vi" "小时数据发送次数"(w3177) -> ()
            }
          }
        }
        frame "上传数据" {
          n1388 = call "提取仪器参数 (子VI).vi"("因子编码"="w01016", "数据输入"=w3202) -> ("字符串"=w3192:string)  [unwired: 9 in]
          n1389 = call "提取仪器参数 (子VI).vi"("因子编码"="w01100", "数据输入"=w3200) -> ("字符串"=w3194:string)  [unwired: 9 in]
          n1390 = call "提取仪器参数 (子VI).vi"("因子编码"="w01014", "数据输入"=w3204) -> ("字符串"=w3196:string)  [unwired: 9 in]
          n1391 = call "提取仪器参数 (子VI).vi"("因子编码"="w01003", "数据输入"=w3203) -> ("字符串"=w3195:string)  [unwired: 9 in]
          n1392 = call "提取仪器参数 (子VI).vi"("因子编码"="w19011", "数据输入"=w3201) -> ("字符串"=w3193:string)  [unwired: 9 in]
          n1393 = call "提取仪器参数 (子VI).vi"("因子编码"="w21011", "数据输入"=w3190) -> ("字符串"=w3188:string)  [unwired: 9 in]
          n1394 = call "提取仪器参数 (子VI).vi"("因子编码"="w01010", "数据输入"=w3205) -> ("字符串"=w3197:string)  [unwired: 9 in]
          n1395 = call "提取仪器参数 (子VI).vi"("因子编码"="w21003", "数据输入"=w3186) -> ("字符串"=w3185:string)  [unwired: 9 in]
          n1396 = call "提取仪器参数 (子VI).vi"("因子编码"="w01001", "数据输入"=w3206) -> ("字符串"=w3198:string)  [unwired: 9 in]
          n1397 = call "提取仪器参数 (子VI).vi"("因子编码"="w01009", "数据输入"=w3214) -> ("字符串"=w3199:string)  [unwired: 9 in]
          n1398 = call "提取仪器参数 (子VI).vi"("因子编码"="w21001", "数据输入"=w3218) -> ("字符串"=w3217:string)  [unwired: 9 in]
          n1399 = call "提取仪器参数 (子VI).vi"("因子编码"="w01018", "数据输入"=w3183) -> ("字符串"=w3182:string)  [unwired: 9 in]
          n1400 = call "提取仪器参数 (子VI).vi"("因子编码"="w01019", "数据输入"=w3180) -> ("字符串"=w3179:string)  [unwired: 9 in]
          n1401 = Concatenate Strings(w3199, w3198, w3197, w3196, w3195, w3192, w3193, w3194) -> (w3191:string)
          n1402 = Concatenate Strings(w3179, w3182, w3185, w3188, w3217, w3191) -> (w3220:string)
          n1403 = Empty String/Path?(string/path=w3220) -> (empty?=w3221:bool)
          n1404 = case shown="假" w3221 {
            tunnel: [w3224 ""] -> w3219
            tunnel: w3220 -> [w3224 _]
            frame False {
              n1405 = global read "全局 小时数据发送次数.vi" "小时数据发送次数"() -> (w3223:i32)
              n1406 = Increment(x=w3223) -> (x+1=w3222:i32)
              n1407 = global write "全局 小时数据发送次数.vi" "小时数据发送次数"(w3222) -> ()
            }
            frame True {
              n1408 = global read "全局 小时数据发送次数.vi" "小时数据发送次数"() -> (w3226:i32)
              n1409 = Increment(x=w3226) -> (x+1=w3225:i32)
              n1410 = global write "全局 小时数据发送次数.vi" "小时数据发送次数"(w3225) -> ()
            }
          }
        }
        frame "返回执行结果" {
        }
      }
    }
    frame "报警信息" {
      n1411 = global read "全局 小时数据发送次数.vi" "小时数据发送次数"() -> (w3237:i32)
      n1412 = global read "全局 小时数据发送次数.vi" "小时数据发送次数"() -> (w3236:i32)
      n1413 = global read "全局 小时数据发送次数.vi" "小时数据发送次数"() -> (w3243:i32)
      n1414 = global read "全局 小时数据发送次数.vi" "小时数据发送次数"() -> (w3240:i32)
      n1415 = global read "全局 小时数据发送次数.vi" "小时数据发送次数"() -> (w3235:i32)
      n1416 = global read "全局 小时数据发送次数.vi" "小时数据发送次数"() -> (w3258:i32)
      n1417 = global read "全局 小时数据发送次数.vi" "小时数据发送次数"() -> (w3246:i32)
      n1418 = global read "全局 小时数据发送次数.vi" "小时数据发送次数"() -> (w3260:i32)
      n1419 = global read "全局 小时数据发送次数.vi" "小时数据发送次数"() -> (w3250:i32)
      n1420 = global read "全局 小时数据发送次数.vi" "小时数据发送次数"() -> (w3256:i32)
      n1421 = global read "全局 小时数据发送次数.vi" "小时数据发送次数"() -> (w3255:i32)
      n1422 = global read "全局 小时数据发送次数.vi" "小时数据发送次数"() -> (w3252:i32)
      n1423 = Index Array(array=w3234, index (row)=w3237) -> (element=w3231:string[])  [unwired: 1 in]
      n1424 = Index Array(array=w3233, index (row)=w3236) -> (element=w3230:string[])  [unwired: 1 in]
      n1425 = Index Array(array=w3242, index (row)=w3243) -> (element=w3241:string[])  [unwired: 1 in]
      n1426 = Index Array(array=w3239, index (row)=w3240) -> (element=w3238:string[])  [unwired: 1 in]
      n1427 = Index Array(array=w3232, index (row)=w3235) -> (element=w3229:string[])  [unwired: 1 in]
      n1428 = Index Array(array=w3265, index (row)=w3258) -> (element=w3257:string[])  [unwired: 1 in]
      n1429 = Index Array(array=w3244, index (row)=w3246) -> (element=w3245:string[])  [unwired: 1 in]
      n1430 = Index Array(array=w3264, index (row)=w3260) -> (element=w3259:string[])  [unwired: 1 in]
      n1431 = Index Array(array=w3249, index (row)=w3250) -> (element=w3248:string[])  [unwired: 1 in]
      n1432 = Index Array(array=w3263, index (row)=w3256) -> (element=w3254:string[])  [unwired: 1 in]
      n1433 = Index Array(array=w3262, index (row)=w3255) -> (element=w3253:string[])  [unwired: 1 in]
      n1434 = global read "全局1.vi" "枚举"() -> (w3261:enum16{"返回请求应答", "上传数据", "返回执行结果"})
      n1435 = Index Array(array=w3247, index (row)=w3252) -> (element=w3251:string[])  [unwired: 1 in]
      n1436 = case shown="\"上传数据\"" w3261 {
        tunnel: ["QnRtn=1" w3341 "ExeRtn=1"] -> w3266
        tunnel: w3259 -> [_ w3360 _]
        tunnel: w3257 -> [_ w3358 _]
        tunnel: w3254 -> [_ w3357 _]
        tunnel: w3253 -> [_ w3356 _]
        tunnel: w3251 -> [_ w3354 _]
        tunnel: w3248 -> [_ w3305 _]
        tunnel: w3245 -> [_ w3302 _]
        tunnel: w3241 -> [_ w3301 _]
        tunnel: w3238 -> [_ w3300 _]
        tunnel: w3231 -> [_ w3299 _]
        tunnel: w3230 -> [_ w3298 _]
        tunnel: w3229 -> [_ w3297 _]
        frame "返回请求应答", Default {
          n1437 = global read "全局 数据数组大小.vi" "数据数组大小"() -> (w3269:i32)
          n1438 = Equal To 0?(x=w3269) -> (x = 0?=w3268:bool)
          n1439 = case shown="真" w3268 {
            frame False {
            }
            frame True {
              n1440 = global read "全局 小时数据发送次数.vi" "小时数据发送次数"() -> (w3271:i32)
              n1441 = Increment(x=w3271) -> (x+1=w3270:i32)
              n1442 = global write "全局 小时数据发送次数.vi" "小时数据发送次数"(w3270) -> ()
            }
          }
        }
        frame "上传数据" {
          n1443 = global read "全局1.vi" "register values"() -> (w3291:u16[])
          n1444 = Index Array(array=w3291, index #1=1 ("索引")) -> (element #1=w3289:u16, element #2=w3287:u16, element #3=w3285:u16, element #4=w3284:u16, element #5=w3283:u16)  [unwired: 4 in]
          n1445 = Number To Decimal String(number=w3283) -> (decimal integer string=w3280:string)  [unwired: 1 in]
          n1446 = Number To Decimal String(number=w3289) -> (decimal integer string=w3288:string)  [unwired: 1 in]
          n1447 = Number To Decimal String(number=w3287) -> (decimal integer string=w3286:string)  [unwired: 1 in]
          n1448 = Number To Decimal String(number=w3285) -> (decimal integer string=w3282:string)  [unwired: 1 in]
          n1449 = Number To Decimal String(number=w3284) -> (decimal integer string=w3281:string)  [unwired: 1 in]
          n1450 = Index Array(array=w3297, index #1=0 ("索引"), index #2=2 ("索引")) -> (element #1=w3310:string, element #2=w3308:string)
          n1451 = Index Array(array=w3299, index #1=0 ("索引"), index #2=2 ("索引")) -> (element #1=w3329:string, element #2=w3338:string)
          n1452 = Index Array(array=w3301, index #1=0 ("索引"), index #2=2 ("索引")) -> (element #1=w3327:string, element #2=w3336:string)
          n1453 = Index Array(array=w3356, index #1=0 ("索引"), index #2=2 ("索引")) -> (element #1=w3355:string, element #2=w3345:string)
          n1454 = Index Array(array=w3360, index #1=0 ("索引"), index #2=2 ("索引")) -> (element #1=w3359:string, element #2=w3347:string)
          n1455 = Empty String/Path?(string/path=w3336) -> (empty?=w3335:bool)
          n1456 = Index Array(array=w3298, index #1=0 ("索引"), index #2=2 ("索引")) -> (element #1=w3311:string, element #2=w3306:string)
          n1457 = Empty String/Path?(string/path=w3308) -> (empty?=w3309:bool)
          n1458 = Empty String/Path?(string/path=w3347) -> (empty?=w3348:bool)
          n1459 = Index Array(array=w3302, index #1=0 ("索引"), index #2=2 ("索引")) -> (element #1=w3330:string, element #2=w3334:string)
          n1460 = Index Array(array=w3300, index #1=0 ("索引"), index #2=2 ("索引")) -> (element #1=w3326:string, element #2=w3340:string)
          n1461 = Index Array(array=w3305, index #1=0 ("索引"), index #2=2 ("索引")) -> (element #1=w3328:string, element #2=w3331:string)
          n1462 = Empty String/Path?(string/path=w3338) -> (empty?=w3337:bool)
          n1463 = case shown="假" w3335 {
            tunnel: [w3492 ""] -> w3296
            tunnel: w3336 -> [w3490 _]
            tunnel: w3327 -> [_ _]
            frame False {
              # "PH"
              n1464 = case shown="\"溶解氧光强异常\"" w3490 {
                tunnel: ["0" ("输入 3") "1" ("输入 3") "2" ("输入 3") "3" ("输入 3") "4" ("输入 3") "5" ("输入 3") "6" ("输入 3") "7" ("输入 3") "8" ("输入 3") "9" ("输入 3") "10" ("输入 3") "11" ("输入 3") "12" ("输入 3") "13" ("输入 3") "14" ("输入 3") "15" ("输入 3") "16" ("输入 3") "17" ("输入 3") "18" ("输入 3") "19" ("输入 3") "20" ("输入 3") "21" ("输入 3")] -> w3489
                frame "无告警" {
                }
                frame "缺试剂告警" {
                }
                frame "缺水样告警" {
                }
                frame "缺蒸馏水告警" {
                }
                frame "缺标液告警" {
                }
                frame "仪表漏液告警" {
                }
                frame "标定异常告警" {
                }
                frame "超量程告警" {
                }
                frame "加热异常" {
                }
                frame "低试剂预警" {
                }
                frame "超上限告警" {
                }
                frame "超下限告警" {
                }
                frame "仪表内部其他异常", Default {
                }
                frame "滴定异常告警" {
                }
                frame "电极异常告警" {
                }
                frame "量程切换告警" {
                }
                frame "参数设置告警" {
                }
                frame "PH电极电位异常" {
                }
                frame "电导率电极异常" {
                }
                frame "浊度光度异常" {
                }
                frame "溶解氧电极异常" {
                }
                frame "溶解氧光强异常" {
                }
              }
              n1465 = Format Into String(format string="PolId=w01001,i12001-Info=%s,i12031-Info=%s;" ("格式字符串"), "0" ("输入 2"), w3489) -> (resulting string=w3492:string)  [unwired: 2 in, 1 out]
            }
            frame True {
            }
          }
          n1466 = Index Array(array=w3354, index #1=0 ("索引"), index #2=2 ("索引")) -> (element #1=w3353:string, element #2=w3349:string)
          n1467 = Empty String/Path?(string/path=w3334) -> (empty?=w3333:bool)
          n1468 = Index Array(array=w3357, index #1=0 ("索引"), index #2=2 ("索引")) -> (element #1=w3361:string, element #2=w3343:string)
          n1469 = Index Array(array=w3358, index #1=0 ("索引"), index #2=2 ("索引")) -> (element #1=w3272:string, element #2=w3352:string)
          n1470 = Empty String/Path?(string/path=w3345) -> (empty?=w3346:bool)
          n1471 = case shown="假" w3348 {
            tunnel: [w3638 ""] -> w3373
            tunnel: w3347 -> [w3637 _]
            tunnel: w3359 -> [_ _]
            tunnel: w3286 -> [w3635 _]
            frame False {
              # "氨氮"
              n1472 = case shown="\"溶解氧光强异常\"" w3637 {
                tunnel: ["0" ("输入 3") "1" ("输入 3") "2" ("输入 3") "3" ("输入 3") "4" ("输入 3") "5" ("输入 3") "6" ("输入 3") "7" ("输入 3") "8" ("输入 3") "9" ("输入 3") "10" ("输入 3") "11" ("输入 3") "12" ("输入 3") "13" ("输入 3") "14" ("输入 3") "15" ("输入 3") "16" ("输入 3") "17" ("输入 3") "18" ("输入 3") "19" ("输入 3") "20" ("输入 3") "21" ("输入 3")] -> w3636
                frame "无告警" {
                }
                frame "缺试剂告警" {
                }
                frame "缺水样告警" {
                }
                frame "缺蒸馏水告警" {
                }
                frame "缺标液告警" {
                }
                frame "仪表漏液告警" {
                }
                frame "标定异常告警" {
                }
                frame "超量程告警" {
                }
                frame "加热异常" {
                }
                frame "低试剂预警" {
                }
                frame "超上限告警" {
                }
                frame "超下限告警" {
                }
                frame "仪表内部其他异常", Default {
                }
                frame "滴定异常告警" {
                }
                frame "电极异常告警" {
                }
                frame "量程切换告警" {
                }
                frame "参数设置告警" {
                }
                frame "PH电极电位异常" {
                }
                frame "电导率电极异常" {
                }
                frame "浊度光度异常" {
                }
                frame "溶解氧电极异常" {
                }
                frame "溶解氧光强异常" {
                }
              }
              n1473 = Format Into String(format string="PolId=w21003,i12001-Info=%s,i12031-Info=%s;" ("格式字符串"), w3635, w3636) -> (resulting string=w3638:string)  [unwired: 2 in, 1 out]
            }
            frame True {
            }
          }
          n1474 = Empty String/Path?(string/path=w3306) -> (empty?=w3307:bool)
          n1475 = Empty String/Path?(string/path=w3349) -> (empty?=w3350:bool)
          n1476 = Empty String/Path?(string/path=w3331) -> (empty?=w3332:bool)
          n1477 = Empty String/Path?(string/path=w3340) -> (empty?=w3339:bool)
          n1478 = case shown="假" w3309 {
            tunnel: [w3408 ""] -> w3292
            tunnel: w3310 -> [_ _]
            tunnel: w3308 -> [w3406 _]
            frame False {
              # "叶绿素"
              n1479 = case shown="\"溶解氧光强异常\"" w3406 {
                tunnel: ["0" ("输入 3") "1" ("输入 3") "2" ("输入 3") "3" ("输入 3") "4" ("输入 3") "5" ("输入 3") "6" ("输入 3") "7" ("输入 3") "8" ("输入 3") "9" ("输入 3") "10" ("输入 3") "11" ("输入 3") "12" ("输入 3") "13" ("输入 3") "14" ("输入 3") "15" ("输入 3") "16" ("输入 3") "17" ("输入 3") "18" ("输入 3") "19" ("输入 3") "20" ("输入 3") "21" ("输入 3")] -> w3405
                frame "无告警" {
                }
                frame "缺试剂告警" {
                }
                frame "缺水样告警" {
                }
                frame "缺蒸馏水告警" {
                }
                frame "缺标液告警" {
                }
                frame "仪表漏液告警" {
                }
                frame "标定异常告警" {
                }
                frame "超量程告警" {
                }
                frame "加热异常" {
                }
                frame "低试剂预警" {
                }
                frame "超上限告警" {
                }
                frame "超下限告警" {
                }
                frame "仪表内部其他异常", Default {
                }
                frame "滴定异常告警" {
                }
                frame "电极异常告警" {
                }
                frame "量程切换告警" {
                }
                frame "参数设置告警" {
                }
                frame "PH电极电位异常" {
                }
                frame "电导率电极异常" {
                }
                frame "浊度光度异常" {
                }
                frame "溶解氧电极异常" {
                }
                frame "溶解氧光强异常" {
                }
              }
              n1480 = Format Into String(format string="PolId=w01016,i12001-Info=%s,i12031-Info=%s;" ("格式字符串"), "0" ("输入 2"), w3405) -> (resulting string=w3408:string)  [unwired: 2 in, 1 out]
            }
            frame True {
            }
          }
          n1481 = case shown="假" w3333 {
            tunnel: [w3521 ""] -> w3303
            tunnel: w3330 -> [_ _]
            tunnel: w3334 -> [w3518 _]
            frame False {
              # "DO"
              n1482 = case shown="\"溶解氧光强异常\"" w3518 {
                tunnel: ["0" ("输入 3") "1" ("输入 3") "2" ("输入 3") "3" ("输入 3") "4" ("输入 3") "5" ("输入 3") "6" ("输入 3") "7" ("输入 3") "8" ("输入 3") "9" ("输入 3") "10" ("输入 3") "11" ("输入 3") "12" ("输入 3") "13" ("输入 3") "14" ("输入 3") "15" ("输入 3") "16" ("输入 3") "17" ("输入 3") "18" ("输入 3") "19" ("输入 3") "20" ("输入 3") "21" ("输入 3")] -> w3517
                frame "无告警" {
                }
                frame "缺试剂告警" {
                }
                frame "缺水样告警" {
                }
                frame "缺蒸馏水告警" {
                }
                frame "缺标液告警" {
                }
                frame "仪表漏液告警" {
                }
                frame "标定异常告警" {
                }
                frame "超量程告警" {
                }
                frame "加热异常" {
                }
                frame "低试剂预警" {
                }
                frame "超上限告警" {
                }
                frame "超下限告警" {
                }
                frame "仪表内部其他异常", Default {
                }
                frame "滴定异常告警" {
                }
                frame "电极异常告警" {
                }
                frame "量程切换告警" {
                }
                frame "参数设置告警" {
                }
                frame "PH电极电位异常" {
                }
                frame "电导率电极异常" {
                }
                frame "浊度光度异常" {
                }
                frame "溶解氧电极异常" {
                }
                frame "溶解氧光强异常" {
                }
              }
              n1483 = Format Into String(format string="PolId=w01009,i22001-Info=%s,i22003-Info=%s;" ("格式字符串"), "0" ("输入 2"), w3517) -> (resulting string=w3521:string)  [unwired: 2 in, 1 out]
            }
            frame True {
            }
          }
          n1484 = Empty String/Path?(string/path=w3352) -> (empty?=w3351:bool)
          n1485 = case shown="假" w3337 {
            tunnel: [w3464 ""] -> w3294
            tunnel: w3329 -> [_ _]
            tunnel: w3338 -> [w3462 _]
            frame False {
              # "水温"
              n1486 = case shown="\"溶解氧光强异常\"" w3462 {
                tunnel: ["0" ("输入 3") "1" ("输入 3") "2" ("输入 3") "3" ("输入 3") "4" ("输入 3") "5" ("输入 3") "6" ("输入 3") "7" ("输入 3") "8" ("输入 3") "9" ("输入 3") "10" ("输入 3") "11" ("输入 3") "12" ("输入 3") "13" ("输入 3") "14" ("输入 3") "15" ("输入 3") "16" ("输入 3") "17" ("输入 3") "18" ("输入 3") "19" ("输入 3") "20" ("输入 3") "21" ("输入 3")] -> w3461
                frame "无告警" {
                }
                frame "缺试剂告警" {
                }
                frame "缺水样告警" {
                }
                frame "缺蒸馏水告警" {
                }
                frame "缺标液告警" {
                }
                frame "仪表漏液告警" {
                }
                frame "标定异常告警" {
                }
                frame "超量程告警" {
                }
                frame "加热异常" {
                }
                frame "低试剂预警" {
                }
                frame "超上限告警" {
                }
                frame "超下限告警" {
                }
                frame "仪表内部其他异常", Default {
                }
                frame "滴定异常告警" {
                }
                frame "电极异常告警" {
                }
                frame "量程切换告警" {
                }
                frame "参数设置告警" {
                }
                frame "PH电极电位异常" {
                }
                frame "电导率电极异常" {
                }
                frame "浊度光度异常" {
                }
                frame "溶解氧电极异常" {
                }
                frame "溶解氧光强异常" {
                }
              }
              n1487 = Format Into String(format string="PolId=w01010,i12001-Info=%s,i12031-Info=%s;" ("格式字符串"), "0" ("输入 2"), w3461) -> (resulting string=w3464:string)  [unwired: 2 in, 1 out]
            }
            frame True {
            }
          }
          n1488 = case shown="假" w3307 {
            tunnel: [w3381 ""] -> w3293
            tunnel: w3311 -> [_ _]
            tunnel: w3306 -> [w3378 _]
            frame False {
              # "浊度"
              n1489 = case shown="\"溶解氧光强异常\"" w3378 {
                tunnel: ["0" ("输入 3") "1" ("输入 3") "2" ("输入 3") "3" ("输入 3") "4" ("输入 3") "5" ("输入 3") "6" ("输入 3") "7" ("输入 3") "8" ("输入 3") "9" ("输入 3") "10" ("输入 3") "11" ("输入 3") "12" ("输入 3") "13" ("输入 3") "14" ("输入 3") "15" ("输入 3") "16" ("输入 3") "17" ("输入 3") "18" ("输入 3") "19" ("输入 3") "20" ("输入 3") "21" ("输入 3")] -> w3377
                frame "无告警" {
                }
                frame "缺试剂告警" {
                }
                frame "缺水样告警" {
                }
                frame "缺蒸馏水告警" {
                }
                frame "缺标液告警" {
                }
                frame "仪表漏液告警" {
                }
                frame "标定异常告警" {
                }
                frame "超量程告警" {
                }
                frame "加热异常" {
                }
                frame "低试剂预警" {
                }
                frame "超上限告警" {
                }
                frame "超下限告警" {
                }
                frame "仪表内部其他异常", Default {
                }
                frame "滴定异常告警" {
                }
                frame "电极异常告警" {
                }
                frame "量程切换告警" {
                }
                frame "参数设置告警" {
                }
                frame "PH电极电位异常" {
                }
                frame "电导率电极异常" {
                }
                frame "浊度光度异常" {
                }
                frame "溶解氧电极异常" {
                }
                frame "溶解氧光强异常" {
                }
              }
              n1490 = Format Into String(format string="PolId=w01003,i12001-Info=%s,i12031-Info=%s;" ("格式字符串"), "0" ("输入 2"), w3377) -> (resulting string=w3381:string)  [unwired: 2 in, 1 out]
            }
            frame True {
            }
          }
          n1491 = Empty String/Path?(string/path=w3343) -> (empty?=w3344:bool)
          n1492 = case shown="假" w3350 {
            tunnel: [w3667 ""] -> w3372
            tunnel: w3353 -> [_ _]
            tunnel: w3349 -> [w3664 _]
            frame False {
              # "系统日志"
              n1493 = case shown="\"仪表内部其他异常\", 默认" w3664 {
                tunnel: ["0" ("输入 3") "1" ("输入 3") "2" ("输入 3") "3" ("输入 3") "4" ("输入 3") "5" ("输入 3") "6" ("输入 3") "7" ("输入 3") "8" ("输入 3") "9" ("输入 3") "10" ("输入 3") "11" ("输入 3") "12" ("输入 3") "13" ("输入 3") "14" ("输入 3") "15" ("输入 3") "16" ("输入 3") "17" ("输入 3") "18" ("输入 3") "19" ("输入 3") "20" ("输入 3") "21" ("输入 3")] -> w3663
                frame "无告警" {
                }
                frame "缺试剂告警" {
                }
                frame "缺水样告警" {
                }
                frame "缺蒸馏水告警" {
                }
                frame "缺标液告警" {
                }
                frame "仪表漏液告警" {
                }
                frame "标定异常告警" {
                }
                frame "超量程告警" {
                }
                frame "加热异常" {
                }
                frame "低试剂预警" {
                }
                frame "超上限告警" {
                }
                frame "超下限告警" {
                }
                frame "仪表内部其他异常", Default {
                }
                frame "滴定异常告警" {
                }
                frame "电极异常告警" {
                }
                frame "量程切换告警" {
                }
                frame "参数设置告警" {
                }
                frame "PH电极电位异常" {
                }
                frame "电导率电极异常" {
                }
                frame "浊度光度异常" {
                }
                frame "溶解氧电极异常" {
                }
                frame "溶解氧光强异常" {
                }
              }
              n1494 = Format Into String(format string="PolId=w00000,i22001-Info=%s,i22003-Info=%s;" ("格式字符串"), "0" ("输入 2"), w3663) -> (resulting string=w3667:string)  [unwired: 2 in, 1 out]
            }
            frame True {
            }
          }
          n1495 = case shown="假" w3339 {
            tunnel: [w3437 ""] -> w3295
            tunnel: w3326 -> [_ _]
            tunnel: w3340 -> [w3434 _]
            frame False {
              # "比电导率"
              n1496 = case shown="\"溶解氧光强异常\"" w3434 {
                tunnel: ["0" ("输入 3") "1" ("输入 3") "2" ("输入 3") "3" ("输入 3") "4" ("输入 3") "5" ("输入 3") "6" ("输入 3") "7" ("输入 3") "8" ("输入 3") "9" ("输入 3") "10" ("输入 3") "11" ("输入 3") "12" ("输入 3") "13" ("输入 3") "14" ("输入 3") "15" ("输入 3") "16" ("输入 3") "17" ("输入 3") "18" ("输入 3") "19" ("输入 3") "20" ("输入 3") "21" ("输入 3")] -> w3433
                frame "无告警" {
                }
                frame "缺试剂告警" {
                }
                frame "缺水样告警" {
                }
                frame "缺蒸馏水告警" {
                }
                frame "缺标液告警" {
                }
                frame "仪表漏液告警" {
                }
                frame "标定异常告警" {
                }
                frame "超量程告警" {
                }
                frame "加热异常" {
                }
                frame "低试剂预警" {
                }
                frame "超上限告警" {
                }
                frame "超下限告警" {
                }
                frame "仪表内部其他异常", Default {
                }
                frame "滴定异常告警" {
                }
                frame "电极异常告警" {
                }
                frame "量程切换告警" {
                }
                frame "参数设置告警" {
                }
                frame "PH电极电位异常" {
                }
                frame "电导率电极异常" {
                }
                frame "浊度光度异常" {
                }
                frame "溶解氧电极异常" {
                }
                frame "溶解氧光强异常" {
                }
              }
              n1497 = Format Into String(format string="PolId=w01014,i12001-Info=%s,i12031-Info=%s;" ("格式字符串"), "0" ("输入 2"), w3433) -> (resulting string=w3437:string)  [unwired: 2 in, 1 out]
            }
            frame True {
            }
          }
          n1498 = case shown="假" w3346 {
            tunnel: [w3610 ""] -> w3368
            tunnel: w3355 -> [_ _]
            tunnel: w3345 -> [w3609 _]
            tunnel: w3281 -> [w3607 _]
            frame False {
              # "总氮"
              n1499 = case shown="\"溶解氧光强异常\"" w3609 {
                tunnel: ["0" ("输入 3") "1" ("输入 3") "2" ("输入 3") "3" ("输入 3") "4" ("输入 3") "5" ("输入 3") "6" ("输入 3") "7" ("输入 3") "8" ("输入 3") "9" ("输入 3") "10" ("输入 3") "11" ("输入 3") "12" ("输入 3") "13" ("输入 3") "14" ("输入 3") "15" ("输入 3") "16" ("输入 3") "17" ("输入 3") "18" ("输入 3") "19" ("输入 3") "20" ("输入 3") "21" ("输入 3")] -> w3608
                frame "无告警" {
                }
                frame "缺试剂告警" {
                }
                frame "缺水样告警" {
                }
                frame "缺蒸馏水告警" {
                }
                frame "缺标液告警" {
                }
                frame "仪表漏液告警" {
                }
                frame "标定异常告警" {
                }
                frame "超量程告警" {
                }
                frame "加热异常" {
                }
                frame "低试剂预警" {
                }
                frame "超上限告警" {
                }
                frame "超下限告警" {
                }
                frame "仪表内部其他异常", Default {
                }
                frame "滴定异常告警" {
                }
                frame "电极异常告警" {
                }
                frame "量程切换告警" {
                }
                frame "参数设置告警" {
                }
                frame "PH电极电位异常" {
                }
                frame "电导率电极异常" {
                }
                frame "浊度光度异常" {
                }
                frame "溶解氧电极异常" {
                }
                frame "溶解氧光强异常" {
                }
              }
              n1500 = Format Into String(format string="PolId=w21001,i12001-Info=%s,i12031-Info=%s;" ("格式字符串"), w3607, w3608) -> (resulting string=w3610:string)  [unwired: 2 in, 1 out]
            }
            frame True {
            }
          }
          n1501 = case shown="假" w3332 {
            tunnel: [w3548 ""] -> w3304
            tunnel: w3328 -> [_ _]
            tunnel: w3331 -> [w3546 _]
            tunnel: w3280 -> [w3545 _]
            frame False {
              # "CODCr"
              n1502 = case shown="\"溶解氧光强异常\"" w3546 {
                tunnel: ["0" ("输入 3") "1" ("输入 3") "2" ("输入 3") "3" ("输入 3") "4" ("输入 3") "5" ("输入 3") "6" ("输入 3") "7" ("输入 3") "8" ("输入 3") "9" ("输入 3") "10" ("输入 3") "11" ("输入 3") "12" ("输入 3") "13" ("输入 3") "14" ("输入 3") "15" ("输入 3") "16" ("输入 3") "17" ("输入 3") "18" ("输入 3") "19" ("输入 3") "20" ("输入 3") "21" ("输入 3")] -> w3547
                frame "无告警" {
                }
                frame "缺试剂告警" {
                }
                frame "缺水样告警" {
                }
                frame "缺蒸馏水告警" {
                }
                frame "缺标液告警" {
                }
                frame "仪表漏液告警" {
                }
                frame "标定异常告警" {
                }
                frame "超量程告警" {
                }
                frame "加热异常" {
                }
                frame "低试剂预警" {
                }
                frame "超上限告警" {
                }
                frame "超下限告警" {
                }
                frame "仪表内部其他异常", Default {
                }
                frame "滴定异常告警" {
                }
                frame "电极异常告警" {
                }
                frame "量程切换告警" {
                }
                frame "参数设置告警" {
                }
                frame "PH电极电位异常" {
                }
                frame "电导率电极异常" {
                }
                frame "浊度光度异常" {
                }
                frame "溶解氧电极异常" {
                }
                frame "溶解氧光强异常" {
                }
              }
              n1503 = Format Into String(format string="PolId=w01018,i12001-Info=%s,i12031-Info=%s;" ("格式字符串"), w3545, w3547) -> (resulting string=w3548:string)  [unwired: 2 in, 1 out]
            }
            frame True {
            }
          }
          n1504 = case shown="假" w3344 {
            tunnel: [w3583 ""] -> w3369
            tunnel: w3361 -> [_ _]
            tunnel: w3343 -> [w3581 _]
            tunnel: w3282 -> [w3579 _]
            frame False {
              # "总磷"
              n1505 = case shown="\"溶解氧光强异常\"" w3581 {
                tunnel: ["0" ("输入 3") "1" ("输入 3") "2" ("输入 3") "3" ("输入 3") "4" ("输入 3") "5" ("输入 3") "6" ("输入 3") "7" ("输入 3") "8" ("输入 3") "9" ("输入 3") "10" ("输入 3") "11" ("输入 3") "12" ("输入 3") "13" ("输入 3") "14" ("输入 3") "15" ("输入 3") "16" ("输入 3") "17" ("输入 3") "18" ("输入 3") "19" ("输入 3") "20" ("输入 3") "21" ("输入 3")] -> w3580
                frame "无告警" {
                }
                frame "缺试剂告警" {
                }
                frame "缺水样告警" {
                }
                frame "缺蒸馏水告警" {
                }
                frame "缺标液告警" {
                }
                frame "仪表漏液告警" {
                }
                frame "标定异常告警" {
                }
                frame "超量程告警" {
                }
                frame "加热异常" {
                }
                frame "低试剂预警" {
                }
                frame "超上限告警" {
                }
                frame "超下限告警" {
                }
                frame "仪表内部其他异常", Default {
                }
                frame "滴定异常告警" {
                }
                frame "电极异常告警" {
                }
                frame "量程切换告警" {
                }
                frame "参数设置告警" {
                }
                frame "PH电极电位异常" {
                }
                frame "电导率电极异常" {
                }
                frame "浊度光度异常" {
                }
                frame "溶解氧电极异常" {
                }
                frame "溶解氧光强异常" {
                }
              }
              n1506 = Format Into String(format string="PolId=w21011,i12001-Info=%s,i12031-Info=%s;" ("格式字符串"), w3579, w3580) -> (resulting string=w3583:string)  [unwired: 2 in, 1 out]
            }
            frame True {
            }
          }
          n1507 = case shown="假" w3351 {
            tunnel: [w3694 ""] -> w3374
            tunnel: w3272 -> [_ _]
            tunnel: w3352 -> [w3692 _]
            tunnel: w3288 -> [w3691 _]
            frame False {
              # "高锰酸钾盐"
              n1508 = case shown="\"缺试剂告警\"" w3692 {
                tunnel: ["0" ("输入 3") "1" ("输入 3") "2" ("输入 3") "3" ("输入 3") "4" ("输入 3") "5" ("输入 3") "6" ("输入 3") "7" ("输入 3") "8" ("输入 3") "9" ("输入 3") "10" ("输入 3") "11" ("输入 3") "12" ("输入 3") "13" ("输入 3") "14" ("输入 3") "15" ("输入 3") "16" ("输入 3") "17" ("输入 3") "18" ("输入 3") "19" ("输入 3") "20" ("输入 3") "21" ("输入 3")] -> w3693
                frame "无告警" {
                }
                frame "缺试剂告警" {
                }
                frame "缺水样告警" {
                }
                frame "缺蒸馏水告警" {
                }
                frame "缺标液告警" {
                }
                frame "仪表漏液告警" {
                }
                frame "标定异常告警" {
                }
                frame "超量程告警" {
                }
                frame "加热异常" {
                }
                frame "低试剂预警" {
                }
                frame "超上限告警" {
                }
                frame "超下限告警" {
                }
                frame "仪表内部其他异常", Default {
                }
                frame "滴定异常告警" {
                }
                frame "电极异常告警" {
                }
                frame "量程切换告警" {
                }
                frame "参数设置告警" {
                }
                frame "PH电极电位异常" {
                }
                frame "电导率电极异常" {
                }
                frame "浊度光度异常" {
                }
                frame "溶解氧电极异常" {
                }
                frame "溶解氧光强异常" {
                }
              }
              n1509 = Format Into String(format string="PolId=w01019,i12001-Info=%s,i12031-Info=%s;" ("格式字符串"), w3691, w3693) -> (resulting string=w3694:string)  [unwired: 2 in, 1 out]
            }
            frame True {
            }
          }
          n1510 = call "规范时间戳.vi"("字符串"=w3272) -> ("result string"=w3274:string)  [unwired: 10 in]
          n1511 = Format Into String(format string="DataTime=%s;", w3274) -> (resulting string=w3273:string)  [unwired: 2 in, 1 out]
          n1512 = Concatenate Strings(w3273, w3374, w3373, w3372, w3369, w3368, w3304, w3303, w3296, w3295, w3294, w3293, w3292) -> (w3277:string)
          n1513 = Empty String/Path?(string/path=w3277) -> (empty?=w3342:bool)
          n1514 = String Length(string=w3277) -> (length=w3279:i32)
          n1515 = Decrement(x=w3279) -> (x-1=w3278:i32)
          n1516 = String Subset(string=w3277, length (rest)=w3278) -> (substring=w3276:string)  [unwired: 1 in]
          n1517 = case shown="假" w3342 {
            tunnel: [w3575 ""] -> w3341
            tunnel: w3276 -> [w3575 _]
            frame False {
              n1518 = global read "全局 小时数据发送次数.vi" "小时数据发送次数"() -> (w3574:i32)
              n1519 = Increment(x=w3574) -> (x+1=w3573:i32)
              n1520 = global write "全局 小时数据发送次数.vi" "小时数据发送次数"(w3573) -> ()
            }
            frame True {
              n1521 = global read "全局 小时数据发送次数.vi" "小时数据发送次数"() -> (w3577:i32)
              n1522 = Increment(x=w3577) -> (x+1=w3576:i32)
              n1523 = global write "全局 小时数据发送次数.vi" "小时数据发送次数"(w3576) -> ()
            }
          }
        }
        frame "返回执行结果" {
        }
      }
    }
    frame "系统状态" {
      # "DataTime=20100301145000;PolId=w01018,i12001-Info=1,i12003-Info=0"
      # "100  当前模式\n101  CODMn状态  （0待机，1运行）\n102  氨氮状态\n103  总磷状态\n104  总氮状态\n105  CODCr状态\n106  运行周期"
      n1524 = global read "全局1.vi" "register values"() -> (w3748:u16[])
      n1525 = Index Array(array=w3748, index #1=1 ("索引")) -> (element #1=w3744:u16, element #2=w3740:u16, element #3=w3734:u16, element #4=w3733:u16, element #5=w3729:u16)  [unwired: 4 in]
      n1526 = Number To Decimal String(number=w3744) -> (decimal integer string=w3743:string)  [unwired: 1 in]
      n1527 = Number To Decimal String(number=w3729) -> (decimal integer string=w3731:string)  [unwired: 1 in]
      n1528 = Number To Decimal String(number=w3734) -> (decimal integer string=w3735:string)  [unwired: 1 in]
      n1529 = Number To Decimal String(number=w3740) -> (decimal integer string=w3739:string)  [unwired: 1 in]
      n1530 = Number To Decimal String(number=w3733) -> (decimal integer string=w3732:string)  [unwired: 1 in]
      n1531 = Format Into String(format string="PolId=w01019,i12001-Info=%s;" ("格式字符串"), w3743) -> (resulting string=w3742:string)  [unwired: 2 in, 1 out]
      n1532 = Format Into String(format string="PolId=w01018,i12001-Info=%s;" ("格式字符串"), w3731) -> (resulting string=w3726:string)  [unwired: 2 in, 1 out]
      n1533 = Format Into String(format string="PolId=w21003,i12001-Info=%s;" ("格式字符串"), w3739) -> (resulting string=w3738:string)  [unwired: 2 in, 1 out]
      n1534 = Format Into String(format string="PolId=w21011,i12001-Info=%s;" ("格式字符串"), w3735) -> (resulting string=w3728:string)  [unwired: 2 in, 1 out]
      n1535 = Format Into String(format string="PolId=w21001,i12001-Info=%s;" ("格式字符串"), w3732) -> (resulting string=w3727:string)  [unwired: 2 in, 1 out]
      n1536 = Get Date/Time In Seconds() -> (seconds since 1Jan1904=w3746:timestamp)
      n1537 = Format Date/Time String(time format string (%c)="%Y%m%d%H%M%S" ("时间格式字符串(%c)"), seconds (now)=w3746) -> (date/time string=w3724:string)  [unwired: 1 in]
      n1538 = Format Into String(format string="DataTime=%s;%s%s%s%s%s" ("格式字符串"), w3724, w3742, w3738, w3728, w3727, w3726) -> (resulting string=w3721:string)  [unwired: 2 in, 1 out]
      n1539 = String Length(string=w3721) -> (length=w3723:i32)
      n1540 = Decrement(x=w3723) -> (x-1=w3722:i32)
      n1541 = String Subset(string=w3721, length (rest)=w3722) -> (substring=w3720:string)  [unwired: 1 in]
    }
    frame "运行模式" {
      # "DataTime=20100301145000;PolId=w01018,i12001-Info=1,i12003-Info=0"
      # "100  当前模式\n101  CODMn状态  （0待机，1运行）\n102  氨氮状态\n103  总磷状态\n104  总氮状态\n105  CODCr状态\n106  运行周期"
      n1542 = global read "全局1.vi" "register values"() -> (w3759:u16[])
      n1543 = Index Array(array=w3759, index=0 ("索引")) -> (element=w3751:u16)
      n1544 = Number To Decimal String(number=w3751) -> (decimal integer string=w3753:string)  [unwired: 1 in]
      n1545 = Format Into String(format string="RunMode=%s;" ("格式字符串"), w3753) -> (resulting string=w3750:string)  [unwired: 2 in, 1 out]
      n1546 = Get Date/Time In Seconds() -> (seconds since 1Jan1904=w3757:timestamp)
      n1547 = Format Date/Time String(time format string (%c)="%Y%m%d%H%M%S" ("时间格式字符串(%c)"), seconds (now)=w3757) -> (date/time string=w3754:string)  [unwired: 1 in]
      n1548 = Format Into String(format string="DataTime=%s;%s" ("格式字符串"), w3754, w3750) -> (resulting string=w3756:string)  [unwired: 2 in, 1 out]
    }
    frame "测量周期" {
      # "DataTime=20100301145000;PolId=w01018,i12001-Info=1,i12003-Info=0"
      # "100  当前模式\n101  CODMn状态  （0待机，1运行）\n102  氨氮状态\n103  总磷状态\n104  总氮状态\n105  CODCr状态\n106  运行周期"
      n1549 = global read "全局1.vi" "register values"() -> (w3770:u16[])
      n1550 = Index Array(array=w3770, index=6 ("索引")) -> (element=w3762:u16)
      n1551 = Number To Decimal String(number=w3762) -> (decimal integer string=w3763:string)  [unwired: 1 in]
      n1552 = Format Into String(format string="RunInterval=%s;" ("格式字符串"), w3763) -> (resulting string=w3761:string)  [unwired: 2 in, 1 out]
      n1553 = Get Date/Time In Seconds() -> (seconds since 1Jan1904=w3768:timestamp)
      n1554 = Format Date/Time String(time format string (%c)="%Y%m%d%H%M%S" ("时间格式字符串(%c)"), seconds (now)=w3768) -> (date/time string=w3765:string)  [unwired: 1 in]
      n1555 = Format Into String(format string="DataTime=%s;%s" ("格式字符串"), w3765, w3761) -> (resulting string=w3767:string)  [unwired: 2 in, 1 out]
    }
    frame "超标留样" {
      # "DataTime=20100301145000;PolId=w01018,i12001-Info=1,i12003-Info=0"
      # "100  当前模式\n101  CODMn状态  （0待机，1运行）\n102  氨氮状态\n103  总磷状态\n104  总氮状态\n105  CODCr状态\n106  运行周期"
      n1556 = global read "全局1.vi" "register values"() -> (w3781:u16[])
      n1557 = Index Array(array=w3781, index=7 ("索引")) -> (element=w3773:u16)
      n1558 = Number To Decimal String(number=w3773) -> (decimal integer string=w3774:string)  [unwired: 1 in]
      n1559 = Format Into String(format string="VaseNo=%s;" ("格式字符串"), w3774) -> (resulting string=w3772:string)  [unwired: 2 in, 1 out]
      n1560 = Get Date/Time In Seconds() -> (seconds since 1Jan1904=w3779:timestamp)
      n1561 = Format Date/Time String(time format string (%c)="%Y%m%d%H%M%S" ("时间格式字符串(%c)"), seconds (now)=w3779) -> (date/time string=w3776:string)  [unwired: 1 in]
      n1562 = Format Into String(format string="DataTime=%s;%s" ("格式字符串"), w3776, w3772) -> (resulting string=w3778:string)  [unwired: 2 in, 1 out]
    }
  }
  n1563 = Equal?(x="table输入", y="反控命令") -> (x = y?=w46:bool)
  n1564 = case shown="假" w46 {
    tunnel: [w3784 w3788] -> w2
    frame False {
      n1565 = global read "全局1.vi" "枚举"() -> (w3783:enum16{"返回请求应答", "上传数据", "返回执行结果"})
      n1566 = case shown="\"上传数据\"" w3783 {
        tunnel: ["91" ("CN") w3786 "91" ("CN")] -> w3784
        frame "返回请求应答", Default {
        }
        frame "上传数据" {
          n1567 = global read "全局1.vi" "系统编码ST"() -> (w3786:string)
        }
        frame "返回执行结果" {
        }
      }
    }
    frame True {
      n1568 = global read "全局 反控命令枚举.vi" "反控命令枚举"() -> (w3789:enum16{"返回请求应答", "返回执行结果"})
      n1569 = case shown="\"返回执行结果\"" w3789 {
        tunnel: ["91" "91"] -> w3788
        frame "返回请求应答", Default {
        }
        frame "返回执行结果" {
        }
      }
    }
  }
  n1570 = case shown="\"实时数据\"" "table输入" {
    tunnel: ["9021" ("ST") w3802 w3810 w3818 w3825 w3832 w3840 w3848 w3857 w3872 w3880 w3888 w3897 w3906 w3923 w3931 w3939 w3947 w3955 w3963 w3974 w3986 w3994 "3020" ("ST") "3042" ("ST") "3056" ("ST") "3015" ("ST")] -> w51
    tunnel: ["1" ("ST") "8" ("ST") "8" ("ST") "8" ("ST") "8" ("ST") "8" ("ST") "8" ("ST") "8" ("ST") "9" ("ST") "9" ("ST") "9" ("ST") "9" ("ST") w3900 "8" ("ST") "9" ("ST") "8" ("ST") "8" ("ST") "9" ("ST") "9" ("ST") "8" ("ST") "9" ("ST") "9" ("ST") "8" ("ST") "9" ("ST") "9" ("ST") "9" ("ST") "9" ("ST")] -> w50
    tunnel: w37 -> [_ w3800 w3808 w3819 w3826 w3833 w3841 w3849 w3858 w3874 w3882 w3890 w3899 w3909 w3925 w3933 w3941 w3949 w3957 w3965 w3976 w3988 w3996 w4002 w4006 w4010 w4014]
    tunnel: [_ w3800 w3808 w3819 w3826 w3833 w3841 w3849 w3858 w3874 w3882 w3890 w3899 w3909 w3925 w3933 w3941 w3949 w3957 w3965 w3976 w3988 w3996 w4002 w4006 w4010 w4014] -> w49
    tunnel: [w3792 w3799 w3807 w3815 w3823 w3830 w3838 w3846 w3854 w3871 w3879 w3887 w3896 w3908 w3921 w3929 w3937 w3945 w3953 w3961 w3969 w3981 w3993 w4001 w4005 w4009 w4013] -> w38
    frame "心跳包", Default {
      # "心跳包"
      n1571 = Get Date/Time In Seconds() -> (seconds since 1Jan1904=w3795:timestamp)
      n1572 = Format Date/Time String(time format string (%c)="%Y%m%d%H%M%S%3u" ("时间格式字符串(%c)"), seconds (now)=w3795) -> (date/time string=w3794:string)  [unwired: 1 in]
      n1573 = Search and Replace String(input string=w3794, search string="." ("搜索字符串")) -> (result string=w3792:string)  [unwired: 6 in, 3 out]
    }
    frame "提取数采仪时间" {
      n1574 = global read "全局1.vi" "枚举"() -> (w3803:enum16{"返回请求应答", "上传数据", "返回执行结果"})
      n1575 = case shown="\"返回执行结果\"" w3803 {
        tunnel: ["9011" ("CN") "1014" ("CN") "9012" ("CN")] -> w3802
        frame "返回请求应答", Default {
        }
        frame "上传数据" {
        }
        frame "返回执行结果" {
        }
      }
      n1576 = local read "QN"() -> (w3799:string)
    }
    frame "提取实时数据间隔" {
      n1577 = global read "全局1.vi" "枚举"() -> (w3811:enum16{"返回请求应答", "上传数据", "返回执行结果"})
      n1578 = case shown="\"上传数据\"" w3811 {
        tunnel: ["9011" ("CN") "1061" ("CN") "9012" ("CN")] -> w3810
        frame "返回请求应答", Default {
        }
        frame "上传数据" {
        }
        frame "返回执行结果" {
        }
      }
      n1579 = local read "QN"() -> (w3807:string)
    }
    frame "反控命令" {
      n1580 = global read "全局 反控命令枚举.vi" "反控命令枚举"() -> (w3816:enum16{"返回请求应答", "返回执行结果"})
      n1581 = case shown="\"返回请求应答\", 默认" w3816 {
        tunnel: ["9011" ("CN") "9012" ("CN")] -> w3818
        frame "返回请求应答", Default {
        }
        frame "返回执行结果" {
        }
      }
      n1582 = local read "QN"() -> (w3815:string)
    }
    frame "超标留样返回" {
      n1583 = global read "全局1.vi" "枚举"() -> (w3822:enum16{"返回请求应答", "上传数据", "返回执行结果"})
      n1584 = case shown="\"上传数据\"" w3822 {
        tunnel: ["9011" ("CN") "3015" ("CN") "9012" ("CN")] -> w3825
        frame "返回请求应答", Default {
        }
        frame "上传数据" {
        }
        frame "返回执行结果" {
        }
      }
      n1585 = local read "QN"() -> (w3823:string)
    }
    frame "提取经纬度环境信息" {
      n1586 = global read "全局1.vi" "枚举"() -> (w3834:enum16{"返回请求应答", "上传数据", "返回执行结果"})
      n1587 = case shown="\"上传数据\"" w3834 {
        tunnel: ["9011" ("CN") "3041" ("CN") "9012" ("CN")] -> w3832
        frame "返回请求应答", Default {
        }
        frame "上传数据" {
        }
        frame "返回执行结果" {
        }
      }
      n1588 = local read "QN"() -> (w3830:string)
    }
    frame "提取现场系统信息" {
      n1589 = global read "全局1.vi" "枚举"() -> (w3842:enum16{"返回请求应答", "上传数据", "返回执行结果"})
      n1590 = case shown="\"上传数据\"" w3842 {
        tunnel: ["9011" ("CN") "3040" ("CN") "9012" ("CN")] -> w3840
        frame "返回请求应答", Default {
        }
        frame "上传数据" {
        }
        frame "返回执行结果" {
        }
      }
      n1591 = local read "QN"() -> (w3838:string)
    }
    frame "提取监测仪表时间" {
      n1592 = global read "全局1.vi" "枚举"() -> (w3850:enum16{"返回请求应答", "上传数据", "返回执行结果"})
      n1593 = case shown="\"返回执行结果\"" w3850 {
        tunnel: ["9011" ("CN") "1011" ("CN") "9012" ("CN")] -> w3848
        frame "返回请求应答", Default {
        }
        frame "上传数据" {
        }
        frame "返回执行结果" {
        }
      }
      n1594 = local read "QN"() -> (w3846:string)
    }
    frame "实时数据" {
      n1595 = global read "全局1.vi" "枚举"() -> (w3856:enum16{"返回请求应答", "上传数据", "返回执行结果"})
      n1596 = case shown="\"上传数据\"" w3856 {
        tunnel: ["9011" ("CN") w3861 "9012" ("CN")] -> w3857
        frame "返回请求应答", Default {
        }
        frame "上传数据" {
          n1597 = global read "全局 实时数据参数.vi" "实时数据参数"() -> (w3860:string)
          n1598 = case shown="\"水样测试\", 默认" w3860 {
            tunnel: ["2011" ("CN") "2064" ("CN") "2082" ("CN") "2063" ("CN") "2062" ("CN") "2065" ("CN") "2066" ("CN") "fff" ("CN")] -> w3861
            frame "水样测试", Default {
            }
            frame "平行样测试" {
            }
            frame "集成干预测试" {
            }
            frame "加标回收测试" {
            }
            frame "核查数据" {
            }
            frame "空白测试" {
            }
            frame "跨度核查" {
            }
            frame "" {
            }
          }
        }
        frame "返回执行结果" {
        }
      }
      n1599 = local read "QN"() -> (w3854:string)
    }
    frame "小时数据" {
      # "监测小时数据"
      n1600 = global read "全局1.vi" "枚举"() -> (w3873:enum16{"返回请求应答", "上传数据", "返回执行结果"})
      n1601 = case shown="\"上传数据\"" w3873 {
        tunnel: ["9011" ("CN") "2061" ("CN") "9012" ("CN")] -> w3872
        frame "返回请求应答", Default {
        }
        frame "上传数据" {
        }
        frame "返回执行结果" {
        }
      }
      n1602 = local read "QN"() -> (w3871:string)
    }
    frame "剖面多参数H" {
      # "监测小时数据"
      n1603 = global read "全局1.vi" "枚举"() -> (w3881:enum16{"返回请求应答", "上传数据", "返回执行结果"})
      n1604 = case shown="\"上传数据\"" w3881 {
        tunnel: ["9011" ("CN") "2061" ("CN") "9012" ("CN")] -> w3880
        frame "返回请求应答", Default {
        }
        frame "上传数据" {
        }
        frame "返回执行结果" {
        }
      }
      n1605 = local read "QN"() -> (w3879:string)
    }
    frame "剖面多参数S" {
      # "监测小时数据"
      n1606 = global read "全局1.vi" "枚举"() -> (w3889:enum16{"返回请求应答", "上传数据", "返回执行结果"})
      n1607 = case shown="\"上传数据\"" w3889 {
        tunnel: ["9011" ("CN") "2011" ("CN") "9012" ("CN")] -> w3888
        frame "返回请求应答", Default {
        }
        frame "上传数据" {
        }
        frame "返回执行结果" {
        }
      }
      n1608 = local read "QN"() -> (w3887:string)
    }
    frame "提取小时数据" {
      # "监测小时数据"
      n1609 = global read "断电保存全局.vi" "数据组合发送"() -> (w3895:bool)
      n1610 = global read "全局1.vi" "枚举"() -> (w3898:enum16{"返回请求应答", "上传数据", "返回执行结果"})
      n1611 = case shown="\"上传数据\"" w3898 {
        tunnel: ["9011" ("CN") "2061" ("CN") "9012" ("CN")] -> w3897
        frame "返回请求应答", Default {
        }
        frame "上传数据" {
        }
        frame "返回执行结果" {
        }
      }
      n1612 = case shown="真" w3895 {
        tunnel: ["8" ("ST") "9" ("ST")] -> w3900
        frame False {
        }
        frame True {
        }
      }
      n1613 = local read "QN"() -> (w3896:string)
    }
    frame "提取实时数据" {
      # "提取实时数据"
      n1614 = global read "全局1.vi" "枚举"() -> (w3907:enum16{"返回请求应答", "上传数据", "返回执行结果"})
      n1615 = case shown="\"上传数据\"" w3907 {
        tunnel: ["9011" ("CN") w3913 "9012" ("CN")] -> w3906
        frame "返回请求应答", Default {
        }
        frame "上传数据" {
          n1616 = global read "全局 实时数据参数.vi" "实时数据参数"() -> (w3912:string)
          n1617 = case shown="\"平行样测试\"" w3912 {
            tunnel: ["2011" ("CN") "2064" ("CN") "2063" ("CN") "2065" ("CN") "2066" ("CN") "fff" ("CN")] -> w3913
            frame "水样测试", Default {
            }
            frame "平行样测试" {
            }
            frame "加标回收测试" {
            }
            frame "空白测试" {
            }
            frame "跨度核查" {
            }
            frame "" {
            }
          }
        }
        frame "返回执行结果" {
        }
      }
      n1618 = local read "QN"() -> (w3908:string)
    }
    frame "跨度核查" {
      # "跨度核查"
      n1619 = global read "全局1.vi" "枚举"() -> (w3924:enum16{"返回请求应答", "上传数据", "返回执行结果"})
      n1620 = case shown="\"上传数据\"" w3924 {
        tunnel: ["9011" ("CN") "2066" ("ST") "9012" ("CN")] -> w3923
        frame "返回请求应答", Default {
        }
        frame "上传数据" {
        }
        frame "返回执行结果" {
        }
      }
      n1621 = local read "QN"() -> (w3921:string)
    }
    frame "提取加标回收" {
      # "提取加标回收"
      n1622 = global read "全局1.vi" "枚举"() -> (w3932:enum16{"返回请求应答", "上传数据", "返回执行结果"})
      n1623 = case shown="\"上传数据\"" w3932 {
        tunnel: ["9011" ("CN") "2063" ("ST") "9012" ("CN")] -> w3931
        frame "返回请求应答", Default {
        }
        frame "上传数据" {
        }
        frame "返回执行结果" {
        }
      }
      n1624 = local read "QN"() -> (w3929:string)
    }
    frame "提取平行样" {
      # "提取平行样"
      n1625 = global read "全局1.vi" "枚举"() -> (w3940:enum16{"返回请求应答", "上传数据", "返回执行结果"})
      n1626 = case shown="\"上传数据\"" w3940 {
        tunnel: ["9011" ("CN") "2064" ("ST") "9012" ("CN")] -> w3939
        frame "返回请求应答", Default {
        }
        frame "上传数据" {
        }
        frame "返回执行结果" {
        }
      }
      n1627 = local read "QN"() -> (w3937:string)
    }
    frame "空白测试", "零点核查" {
      # "零点核查"
      n1628 = global read "全局1.vi" "枚举"() -> (w3948:enum16{"返回请求应答", "上传数据", "返回执行结果"})
      n1629 = case shown="\"上传数据\"" w3948 {
        tunnel: ["9011" ("CN") "2065" ("ST") "9012" ("CN")] -> w3947
        frame "返回请求应答", Default {
        }
        frame "上传数据" {
        }
        frame "返回执行结果" {
        }
      }
      n1630 = local read "QN"() -> (w3945:string)
    }
    frame "核查数据" {
      # "核查数据"
      n1631 = global read "全局1.vi" "枚举"() -> (w3956:enum16{"返回请求应答", "上传数据", "返回执行结果"})
      n1632 = case shown="\"上传数据\"" w3956 {
        tunnel: ["9011" ("CN") "2062" ("ST") "9012" ("CN")] -> w3955
        frame "返回请求应答", Default {
        }
        frame "上传数据" {
        }
        frame "返回执行结果" {
        }
      }
      n1633 = local read "QN"() -> (w3953:string)
    }
    frame "提取集成干预" {
      # "核查数据"
      n1634 = global read "全局1.vi" "枚举"() -> (w3964:enum16{"返回请求应答", "上传数据", "返回执行结果"})
      n1635 = case shown="\"上传数据\"" w3964 {
        tunnel: ["9011" ("CN") "2082" ("ST") "9012" ("CN")] -> w3963
        frame "返回请求应答", Default {
        }
        frame "上传数据" {
        }
        frame "返回执行结果" {
        }
      }
      n1636 = local read "QN"() -> (w3961:string)
    }
    frame "报警信息", "操作日志", "仪器参数" {
      n1637 = global read "全局1.vi" "枚举"() -> (w3975:enum16{"返回请求应答", "上传数据", "返回执行结果"})
      n1638 = case shown="\"上传数据\"" w3975 {
        tunnel: ["9011" ("CN") "3020" ("CN") "9012" ("CN")] -> w3974
        frame "返回请求应答", Default {
        }
        frame "上传数据" {
        }
        frame "返回执行结果" {
        }
      }
      n1639 = Get Date/Time In Seconds() -> (seconds since 1Jan1904=w3972:timestamp)
      n1640 = Format Date/Time String(time format string (%c)="%Y%m%d%H%M%S%3u" ("时间格式字符串(%c)"), seconds (now)=w3972) -> (date/time string=w3971:string)  [unwired: 1 in]
      n1641 = Search and Replace String(input string=w3971, search string="." ("搜索字符串")) -> (result string=w3969:string)  [unwired: 6 in, 3 out]
    }
    frame "3090仪器参数" {
      n1642 = global read "全局1.vi" "枚举"() -> (w3987:enum16{"返回请求应答", "上传数据", "返回执行结果"})
      n1643 = case shown="\"上传数据\"" w3987 {
        tunnel: ["9011" ("CN") "3090" ("CN") "9012" ("CN")] -> w3986
        frame "返回请求应答", Default {
        }
        frame "上传数据" {
        }
        frame "返回执行结果" {
        }
      }
      n1644 = Get Date/Time In Seconds() -> (seconds since 1Jan1904=w3984:timestamp)
      n1645 = Format Date/Time String(time format string (%c)="%Y%m%d%H%M%S%3u" ("时间格式字符串(%c)"), seconds (now)=w3984) -> (date/time string=w3983:string)  [unwired: 1 in]
      n1646 = Search and Replace String(input string=w3983, search string="." ("搜索字符串")) -> (result string=w3981:string)  [unwired: 6 in, 3 out]
    }
    frame "提取仪器参数" {
      n1647 = global read "全局1.vi" "枚举"() -> (w3995:enum16{"返回请求应答", "上传数据", "返回执行结果"})
      n1648 = case shown="\"上传数据\"" w3995 {
        tunnel: ["9011" ("CN") "3020" ("CN") "9012" ("CN")] -> w3994
        frame "返回请求应答", Default {
        }
        frame "上传数据" {
        }
        frame "返回执行结果" {
        }
      }
      n1649 = local read "QN"() -> (w3993:string)
    }
    frame "系统状态" {
      n1650 = local read "QN"() -> (w4001:string)
    }
    frame "运行模式" {
      n1651 = local read "QN"() -> (w4005:string)
    }
    frame "测量周期" {
      n1652 = local read "QN"() -> (w4009:string)
    }
    frame "超标留样" {
      n1653 = local read "QN"() -> (w4013:string)
    }
  }
  n1654 = case shown="\"假\", 默认" "table输入" {
    tunnel: [w4017 "91" ("ST")] -> w4
    tunnel: w2 -> [w4017 _]
    frame "假", Default {
    }
    frame "心跳包" {
    }
  }
  n1655 = Bundle By Name(cluster="数据块", "ST"=w4, "CN"=w51, "FLAG"=w50, "CP"=w49, "QN"=w38, "MN"="MN", "PW"="PW", "PNUM"=w42, "PNO"=w42) -> (w48:T1)
  n1656 = call "HJ212-2017.vi"("PWD？"=FALSE, "数据段"=w48) -> ("通讯包字符串"=w55:string, "通讯包"=→"通讯包":T2)  [unwired: 7 in, 1 out]
  "通讯包字符串" <- w55
  n1657 = String Length(string=w55) -> (length=→"长度":i32)
  "错误常量" <- "错误常量 2"
  "小时数据发送次数" <- 0 ("小时数据发送次数")
  "核查数据发送次数" <- 0 ("核查数据发送次数")
